vi "App Linker Info.vi"() -> ()   [LabVIEW 2020]
panel:
  out "Array 2":T1(array[cluster])=[{"Paths"=path "C:/dev/Vireo/PicoG/PicoG-App/picoG/Main UI.vi/38877c1a-f453-4dae-9d92-84bd5ba51cbc.vi", "error out"={"status"=TRUE, "code"=7, "source"="Invoke Node in App Linker Info.vi\n<APPEND>\nMethod Name: <b>Linker:Read Info From File</b>\n\nC:\\dev\\Vireo\\PicoG\\PicoG-App\\picoG\\Main UI.vi\\38877c1a-f453-4dae-9d92-84bd5ba51cbc.vi"}}, {"Paths"=path "C:/dev/Vireo/PicoG/PicoG-App/picoG/_Add App.vi/4267f4de-baa5-4d76-a96e-fc062378f624.vi", "error out"={"status"=TRUE, "code"=7, "source"="Invoke Node in App Linker Info.vi\n<APPEND>\nMethod Name: <b>Linker:Read Info From File</b>\n\nC:\\dev\\Vireo\\PicoG\\PicoG-App\\picoG\\_Add App.vi\\4267f4de-baa5-4d76-a96e-fc062378f624.vi"}}, {"Paths"=path "C:/dev/Vireo/PicoG/PicoG-App/picoG/_Add App.vi/0", "error out"={"status"=TRUE, "code"=7, "source"="Invoke Node in App Linker Info.vi\n<APPEND>\nMethod Name: <b>Linker:Read Info From File</b>\n\nC:\\dev\\Vireo\\PicoG\\PicoG-App\\picoG\\_Add App.vi\\0"}}, {"Paths"=path "C:/dev/Vireo/PicoG/Builds/picoG/ppl/PicoG-Core.lvlibp/PicoG-Processor/PicoG-Core/PlatformPluginManager/Platform by Name.vi", "error out"={"status"=TRUE, "code"=7, "source"="Invoke Node in App Linker Info.vi\n<APPEND>\nMethod Name: <b>Linker:Read Info From File</b>\n\nC:\\dev\\Vireo\\PicoG\\Builds\\picoG\\ppl\\PicoG-Core.lvlibp\\PicoG-Processor\\PicoG-Core\\PlatformPluginManager\\Platform by Name.vi"}}, {"Paths"=path "C:/dev/Vireo/PicoG/Builds/picoG/ppl/PicoG-Core.lvlibp/1abvi3w/vi.lib/Utility/LVClass/Get LV Class Default Value.vi/LabVIEW", "error out"={"status"=TRUE, "code"=7, "source"="Invoke Node in App Linker Info.vi\n<APPEND>\nMethod Name: <b>Linker:Read Info From File</b>\n\nC:\\dev\\Vireo\\PicoG\\Builds\\picoG\\ppl\\PicoG-Core.lvlibp\\1abvi3w\\vi.lib\\Utility\\LVClass\\Get LV Class Default Value.vi\\LabVIEW"}}]
  out "Array":T2(array[cluster])=[{"Path"=path "C:/dev/Vireo/PicoG/PicoG-App/picoG Main.vi", "Name"="PicoG-App.lvlib:picoG Main.vi", "Referrer"=path "C:/dev/Vireo/PicoG/PicoG-App/picoG Main.vi"}, {"Path"=path "../PicoG-App.lvlib", "Name"="PicoG-App.lvlib", "Referrer"=path "C:/dev/Vireo/PicoG/PicoG-App/picoG Main.vi"}, {"Path"=path "<vilib>/Utility/error.llb/Clear Errors.vi", "Name"="Clear Errors.vi", "Referrer"=path "C:/dev/Vireo/PicoG/PicoG-App/picoG Main.vi"}, {"Path"=path "../picoG/Ctor.vi", "Name"="PicoG-App.lvlib:picoG.lvclass:Ctor.vi", "Referrer"=path "C:/dev/Vireo/PicoG/PicoG-App/picoG Main.vi"}, {"Path"=path "../picoG/Run.vi", "Name"="PicoG-App.lvlib:picoG.lvclass:Run.vi", "Referrer"=path "C:/dev/Vireo/PicoG/PicoG-App/picoG Main.vi"}, {"Path"=path "../picoG/Cleanup.vi", "Name"="PicoG-App.lvlib:picoG.lvclass:Cleanup.vi", "Referrer"=path "C:/dev/Vireo/PicoG/PicoG-App/picoG Main.vi"}, {"Path"=path "<vilib>/Utility/error.llb/Simple Error Handler.vi", "Name"="Simple Error Handler.vi", "Referrer"=path "C:/dev/Vireo/PicoG/PicoG-App/picoG Main.vi"}, {"Path"=path "C:/dev/Vireo/PicoG/PicoG-App/PicoG-App.lvlib", "Name"="PicoG-App.lvlib", "Referrer"=path "C:/dev/Vireo/PicoG/PicoG-App/PicoG-App.lvlib"}, {"Path"=path "C:/dev/Vireo/PicoG/PicoG-App/Device/Device.lvclass", "Name"="PicoG-App.lvlib:Device.lvclass", "Referrer"=path "C:/dev/Vireo/PicoG/PicoG-App/PicoG-App.lvlib"}, {"Path"=path "C:/dev/Vireo/PicoG/PicoG-App/ViaApp/ViaApp.lvclass", "Name"="PicoG-App.lvlib:ViaApp.lvclass", "Referrer"=path "C:/dev/Vireo/PicoG/PicoG-App/PicoG-App.lvlib"}, {"Path"=path "C:/dev/Vireo/PicoG/PicoG-App/AppDetailPanel/AppDetailPanel.lvclass", "Name"="PicoG-App.lvlib:AppDetailPanel.lvclass", "Referrer"=path "C:/dev/Vireo/PicoG/PicoG-App/PicoG-App.lvlib"}, {"Path"=path "C:/dev/Vireo/PicoG/PicoG-App/DeviceDetailPanel/DeviceDetailPanel.lvclass", "Name"="PicoG-App.lvlib:DeviceDetailPanel.lvclass", "Referrer"=path "C:/dev/Vireo/PicoG/PicoG-App/PicoG-App.lvlib"}, {"Path"=path "C:/dev/Vireo/PicoG/PicoG-App/PlatformConfigPanel/PlatformConfigPanel.lvclass", "Name"="PicoG-App.lvlib:PlatformConfigPanel.lvclass", "Referrer"=path "C:/dev/Vireo/PicoG/PicoG-App/PicoG-App.lvlib"}, {"Path"=path "C:/dev/Vireo/PicoG/PicoG-App/AppListPanel/AppListPanel.lvclass", "Name"="PicoG-App.lvlib:AppListPanel.lvclass", "Referrer"=path "C:/dev/Vireo/PicoG/PicoG-App/PicoG-App.lvlib"}, {"Path"=path "C:/dev/Vireo/PicoG/PicoG-App/DeviceListPanel/DeviceListPanel.lvclass", "Name"="PicoG-App.lvlib:DeviceListPanel.lvclass", "Referrer"=path "C:/dev/Vireo/PicoG/PicoG-App/PicoG-App.lvlib"}, {"Path"=path "C:/dev/Vireo/PicoG/PicoG-App/PlatformListPanel/PlatformListPanel.lvclass", "Name"="PicoG-App.lvlib:PlatformListPanel.lvclass", "Referrer"=path "C:/dev/Vireo/PicoG/PicoG-App/PicoG-App.lvlib"}, {"Path"=path "C:/dev/Vireo/PicoG/PicoG-App/BoardArrayPanel/BoardArrayPanel.lvclass", "Name"="PicoG-App.lvlib:BoardArrayPanel.lvclass", "Referrer"=path "C:/dev/Vireo/PicoG/PicoG-App/PicoG-App.lvlib"}, {"Path"=path "C:/dev/Vireo/PicoG/PicoG-App/DeviceArrayPanel/DeviceArrayPanel.lvclass", "Name"="PicoG-App.lvlib:DeviceArrayPanel.lvclass", "Referrer"=path "C:/dev/Vireo/PicoG/PicoG-App/PicoG-App.lvlib"}, {"Path"=path "C:/dev/Vireo/PicoG/PicoG-App/GWebAppArrayPanel/GWebAppArrayPanel.lvclass", "Name"="PicoG-App.lvlib:GWebAppArrayPanel.lvclass", "Referrer"=path "C:/dev/Vireo/PicoG/PicoG-App/PicoG-App.lvlib"}, {"Path"=path "C:/dev/Vireo/PicoG/PicoG-App/PlatformArrayPanel/PlatformArrayPanel.lvclass", "Name"="PicoG-App.lvlib:PlatformArrayPanel.lvclass", "Referrer"=path "C:/dev/Vireo/PicoG/PicoG-App/PicoG-App.lvlib"}, {"Path"=path "C:/dev/Vireo/PicoG/PicoG-App/GettingStarted/GettingStarted.lvclass", "Name"="PicoG-App.lvlib:GettingStarted.lvclass", "Referrer"=path "C:/dev/Vireo/PicoG/PicoG-App/PicoG-App.lvlib"}, {"Path"=path "C:/dev/Vireo/PicoG/PicoG-App/Config Paths.vi", "Name"="PicoG-App.lvlib:Config Paths.vi", "Referrer"=path "C:/dev/Vireo/PicoG/PicoG-App/PicoG-App.lvlib"}, {"Path"=path "C:/dev/Vireo/PicoG/PicoG-App/Paths.ctl", "Name"="PicoG-App.lvlib:Paths.ctl", "Referrer"=path "C:/dev/Vireo/PicoG/PicoG-App/PicoG-App.lvlib"}, {"Path"=path "C:/dev/Vireo/PicoG/PicoG-App/picoG/Top VI FG.vi", "Name"="PicoG-App.lvlib:Top VI FG.vi", "Referrer"=path "C:/dev/Vireo/PicoG/PicoG-App/PicoG-App.lvlib"}, {"Path"=path "C:/dev/Vireo/PicoG/PicoG-App/App Watcher/App Watcher.lvclass", "Name"="PicoG-App.lvlib:App Watcher.lvclass", "Referrer"=path "C:/dev/Vireo/PicoG/PicoG-App/PicoG-App.lvlib"}, {"Path"=path "C:/dev/Vireo/PicoG/PicoG-App/Device Watcher/Device Watcher.lvclass", "Name"="PicoG-App.lvlib:Device Watcher.lvclass", "Referrer"=path "C:/dev/Vireo/PicoG/PicoG-App/PicoG-App.lvlib"}, {"Path"=path "C:/dev/Vireo/PicoG/PicoG-App/picoG Main.vi", "Name"="PicoG-App.lvlib:picoG Main.vi", "Referrer"=path "C:/dev/Vireo/PicoG/PicoG-App/PicoG-App.lvlib"}, {"Path"=path "C:/dev/Vireo/PicoG/PicoG-App/picoG/picoG.lvclass", "Name"="PicoG-App.lvlib:picoG.lvclass", "Referrer"=path "C:/dev/Vireo/PicoG/PicoG-App/PicoG-App.lvlib"}, {"Path"=path "C:/dev/Vireo/PicoG/PicoG-App/picoG/Ctor.vi", "Name"="PicoG-App.lvlib:picoG.lvclass:Ctor.vi", "Referrer"=path "C:/dev/Vireo/PicoG/PicoG-App/picoG/Ctor.vi"}, {"Path"=path "../picoG.lvclass", "Name"="PicoG-App.lvlib:picoG.lvclass", "Referrer"=path "C:/dev/Vireo/PicoG/PicoG-App/picoG/Ctor.vi"}, {"Path"=path "../picoG.lvclass/picoG.ctl", "Name"="PicoG-App.lvlib:picoG.lvclass:picoG.ctl", "Referrer"=path "C:/dev/Vireo/PicoG/PicoG-App/picoG/Ctor.vi"}, {"Path"=path "../Init Platform Plugins.vi", "Name"="PicoG-App.lvlib:picoG.lvclass:Init Platform Plugins.vi", "Referrer"=path "C:/dev/Vireo/PicoG/PicoG-App/picoG/Ctor.vi"}, {"Path"=path "../Init Events.vi", "Name"="PicoG-App.lvlib:picoG.lvclass:Init Events.vi", "Referrer"=path "C:/dev/Vireo/PicoG/PicoG-App/picoG/Ctor.vi"}, {"Path"=path "../Init Panels.vi", "Name"="PicoG-App.lvlib:picoG.lvclass:Init Panels.vi", "Referrer"=path "C:/dev/Vireo/PicoG/PicoG-App/picoG/Ctor.vi"}, {"Path"=path "../Init App Watcher.vi", "Name"="PicoG-App.lvlib:picoG.lvclass:Init App Watcher.vi", "Referrer"=path "C:/dev/Vireo/PicoG/PicoG-App/picoG/Ctor.vi"}, {"Path"=path "../Init Device Watcher.vi", "Name"="PicoG-App.lvlib:picoG.lvclass:Init Device Watcher.vi", "Referrer"=path "C:/dev/Vireo/PicoG/PicoG-App/picoG/Ctor.vi"}, {"Path"=path "../Init Config.vi", "Name"="PicoG-App.lvlib:picoG.lvclass:Init Config.vi", "Referrer"=path "C:/dev/Vireo/PicoG/PicoG-App/picoG/Ctor.vi"}, {"Path"=path "../Instance FG.vi", "Name"="PicoG-App.lvlib:picoG.lvclass:Instance FG.vi", "Referrer"=path "C:/dev/Vireo/PicoG/PicoG-App/picoG/Ctor.vi"}, {"Path"=path "C:/dev/Vireo/PicoG/PicoG-App/picoG/Run.vi", "Name"="PicoG-App.lvlib:picoG.lvclass:Run.vi", "Referrer"=path "C:/dev/Vireo/PicoG/PicoG-App/picoG/Run.vi"}, {"Path"=path "../picoG.lvclass", "Name"="PicoG-App.lvlib:picoG.lvclass", "Referrer"=path "C:/dev/Vireo/PicoG/PicoG-App/picoG/Run.vi"}, {"Path"=path "../Main UI.vi", "Name"="PicoG-App.lvlib:picoG.lvclass:Main UI.vi", "Referrer"=path "C:/dev/Vireo/PicoG/PicoG-App/picoG/Run.vi"}, {"Path"=path "../../App Watcher/Start.vi", "Name"="PicoG-App.lvlib:App Watcher.lvclass:Start.vi", "Referrer"=path "C:/dev/Vireo/PicoG/PicoG-App/picoG/Run.vi"}, {"Path"=path "C:/dev/Vireo/PicoG/PicoG-App/picoG/Cleanup.vi", "Name"="PicoG-App.lvlib:picoG.lvclass:Cleanup.vi", "Referrer"=path "C:/dev/Vireo/PicoG/PicoG-App/picoG/Cleanup.vi"}, {"Path"=path "../picoG.lvclass", "Name"="PicoG-App.lvlib:picoG.lvclass", "Referrer"=path "C:/dev/Vireo/PicoG/PicoG-App/picoG/Cleanup.vi"}, {"Path"=path "../picoG.lvclass/picoG.ctl", "Name"="PicoG-App.lvlib:picoG.lvclass:picoG.ctl", "Referrer"=path "C:/dev/Vireo/PicoG/PicoG-App/picoG/Cleanup.vi"}, {"Path"=path "../../App Watcher/Cleanup.vi", "Name"="PicoG-App.lvlib:App Watcher.lvclass:Cleanup.vi", "Referrer"=path "C:/dev/Vireo/PicoG/PicoG-App/picoG/Cleanup.vi"}, {"Path"=path "<vilib>/IlluminatedG/IG OOPanel/OOPanel/Manager/Cleanup.vi", "Name"="OOPanel.lvlib:Manager.lvclass:Cleanup.vi", "Referrer"=path "C:/dev/Vireo/PicoG/PicoG-App/picoG/Cleanup.vi"}, {"Path"=path "../../../Builds/picoG/ppl/PicoG-Core.lvlibp/PicoG-Processor/PicoG-Core/PlatformManager/Cleanup.vi", "Name"="PicoG-Core.lvlibp:PlatformManager.lvclass:Cleanup.vi", "Referrer"=path "C:/dev/Vireo/PicoG/PicoG-App/picoG/Cleanup.vi"}, {"Path"=path "C:/dev/Vireo/PicoG/PicoG-App/picoG/picoG.lvclass", "Name"="PicoG-App.lvlib:picoG.lvclass", "Referrer"=path "C:/dev/Vireo/PicoG/PicoG-App/picoG/picoG.lvclass"}, {"Path"=path "C:/dev/Vireo/PicoG/PicoG-App/PicoG-App.lvlib", "Name"="PicoG-App.lvlib", "Referrer"=path "C:/dev/Vireo/PicoG/PicoG-App/picoG/picoG.lvclass"}, {"Path"=path "C:/dev/Vireo/PicoG/PicoG-App/picoG/picoG.lvclass/picoG.ctl", "Name"="PicoG-App.lvlib:picoG.lvclass:picoG.ctl", "Referrer"=path "C:/dev/Vireo/PicoG/PicoG-App/picoG/picoG.lvclass"}, {"Path"=path "C:/dev/Vireo/PicoG/PicoG-App/picoG/Check Configs Exist.vi", "Name"="PicoG-App.lvlib:picoG.lvclass:Check Configs Exist.vi", "Referrer"=path "C:/dev/Vireo/PicoG/PicoG-App/picoG/picoG.lvclass"}, {"Path"=path "C:/dev/Vireo/PicoG/PicoG-App/picoG/Create Default System Config.vi", "Name"="PicoG-App.lvlib:picoG.lvclass:Create Default System Config.vi", "Referrer"=path "C:/dev/Vireo/PicoG/PicoG-App/picoG/picoG.lvclass"}, {"Path"=path "C:/dev/Vireo/PicoG/PicoG-App/picoG/Create Default User Config.vi", "Name"="PicoG-App.lvlib:picoG.lvclass:Create Default User Config.vi", "Referrer"=path "C:/dev/Vireo/PicoG/PicoG-App/picoG/picoG.lvclass"}, {"Path"=path "C:/dev/Vireo/PicoG/PicoG-App/picoG/Init Config.vi", "Name"="PicoG-App.lvlib:picoG.lvclass:Init Config.vi", "Referrer"=path "C:/dev/Vireo/PicoG/PicoG-App/picoG/picoG.lvclass"}, {"Path"=path "C:/dev/Vireo/PicoG/PicoG-App/picoG/Load Platform Config.vi", "Name"="PicoG-App.lvlib:picoG.lvclass:Load Platform Config.vi", "Referrer"=path "C:/dev/Vireo/PicoG/PicoG-App/picoG/picoG.lvclass"}, {"Path"=path "C:/dev/Vireo/PicoG/PicoG-App/picoG/Load User Apps.vi", "Name"="PicoG-App.lvlib:picoG.lvclass:Load User Apps.vi", "Referrer"=path "C:/dev/Vireo/PicoG/PicoG-App/picoG/picoG.lvclass"}, {"Path"=path "C:/dev/Vireo/PicoG/PicoG-App/picoG/Load User Devices.vi", "Name"="PicoG-App.lvlib:picoG.lvclass:Load User Devices.vi", "Referrer"=path "C:/dev/Vireo/PicoG/PicoG-App/picoG/picoG.lvclass"}, {"Path"=path "C:/dev/Vireo/PicoG/PicoG-App/picoG/Load User Preferences.vi", "Name"="PicoG-App.lvlib:picoG.lvclass:Load User Preferences.vi", "Referrer"=path "C:/dev/Vireo/PicoG/PicoG-App/picoG/picoG.lvclass"}, {"Path"=path "C:/dev/Vireo/PicoG/PicoG-App/picoG/Read Single Device.vi", "Name"="PicoG-App.lvlib:picoG.lvclass:Read Single Device.vi", "Referrer"=path "C:/dev/Vireo/PicoG/PicoG-App/picoG/picoG.lvclass"}, {"Path"=path "C:/dev/Vireo/PicoG/PicoG-App/picoG/Read User Apps.vi", "Name"="PicoG-App.lvlib:picoG.lvclass:Read User Apps.vi", "Referrer"=path "C:/dev/Vireo/PicoG/PicoG-App/picoG/picoG.lvclass"}, {"Path"=path "C:/dev/Vireo/PicoG/PicoG-App/picoG/Read User Devices.vi", "Name"="PicoG-App.lvlib:picoG.lvclass:Read User Devices.vi", "Referrer"=path "C:/dev/Vireo/PicoG/PicoG-App/picoG/picoG.lvclass"}, {"Path"=path "C:/dev/Vireo/PicoG/PicoG-App/picoG/Save Config.vi", "Name"="PicoG-App.lvlib:picoG.lvclass:Save Config.vi", "Referrer"=path "C:/dev/Vireo/PicoG/PicoG-App/picoG/picoG.lvclass"}, {"Path"=path "C:/dev/Vireo/PicoG/PicoG-App/picoG/Save User Apps.vi", "Name"="PicoG-App.lvlib:picoG.lvclass:Save User Apps.vi", "Referrer"=path "C:/dev/Vireo/PicoG/PicoG-App/picoG/picoG.lvclass"}, {"Path"=path "C:/dev/Vireo/PicoG/PicoG-App/picoG/Save User Devices.vi", "Name"="PicoG-App.lvlib:picoG.lvclass:Save User Devices.vi", "Referrer"=path "C:/dev/Vireo/PicoG/PicoG-App/picoG/picoG.lvclass"}, {"Path"=path "C:/dev/Vireo/PicoG/PicoG-App/picoG/Write Single Device.vi", "Name"="PicoG-App.lvlib:picoG.lvclass:Write Single Device.vi", "Referrer"=path "C:/dev/Vireo/PicoG/PicoG-App/picoG/picoG.lvclass"}, {"Path"=path "C:/dev/Vireo/PicoG/PicoG-App/picoG/Inbound Events.ctl", "Name"="PicoG-App.lvlib:picoG.lvclass:Inbound Events.ctl", "Referrer"=path "C:/dev/Vireo/PicoG/PicoG-App/picoG/picoG.lvclass"}, {"Path"=path "C:/dev/Vireo/PicoG/PicoG-App/picoG/List Panels.ctl", "Name"="PicoG-App.lvlib:picoG.lvclass:List Panels.ctl", "Referrer"=path "C:/dev/Vireo/PicoG/PicoG-App/picoG/picoG.lvclass"}, {"Path"=path "C:/dev/Vireo/PicoG/PicoG-App/picoG/Main Panels.ctl", "Name"="PicoG-App.lvlib:picoG.lvclass:Main Panels.ctl", "Referrer"=path "C:/dev/Vireo/PicoG/PicoG-App/picoG/picoG.lvclass"}, {"Path"=path "C:/dev/Vireo/PicoG/PicoG-App/picoG/Panels.ctl", "Name"="PicoG-App.lvlib:picoG.lvclass:Panels.ctl", "Referrer"=path "C:/dev/Vireo/PicoG/PicoG-App/picoG/picoG.lvclass"}, {"Path"=path "C:/dev/Vireo/PicoG/PicoG-App/picoG/UI State.ctl", "Name"="PicoG-App.lvlib:picoG.lvclass:UI State.ctl", "Referrer"=path "C:/dev/Vireo/PicoG/PicoG-App/picoG/picoG.lvclass"}, {"Path"=path "C:/dev/Vireo/PicoG/PicoG-App/picoG/Add Device.vi", "Name"="PicoG-App.lvlib:picoG.lvclass:Add Device.vi", "Referrer"=path "C:/dev/Vireo/PicoG/PicoG-App/picoG/picoG.lvclass"}, {"Path"=path "C:/dev/Vireo/PicoG/PicoG-App/picoG/Init Device Watcher.vi", "Name"="PicoG-App.lvlib:picoG.lvclass:Init Device Watcher.vi", "Referrer"=path "C:/dev/Vireo/PicoG/PicoG-App/picoG/picoG.lvclass"}, {"Path"=path "C:/dev/Vireo/PicoG/PicoG-App/picoG/Init Events.vi", "Name"="PicoG-App.lvlib:picoG.lvclass:Init Events.vi", "Referrer"=path "C:/dev/Vireo/PicoG/PicoG-App/picoG/picoG.lvclass"}, {"Path"=path "C:/dev/Vireo/PicoG/PicoG-App/picoG/Confirm Device UI.vi", "Name"="PicoG-App.lvlib:picoG.lvclass:Confirm Device UI.vi", "Referrer"=path "C:/dev/Vireo/PicoG/PicoG-App/picoG/picoG.lvclass"}, {"Path"=path "C:/dev/Vireo/PicoG/PicoG-App/picoG/Dock UI.vi", "Name"="PicoG-App.lvlib:picoG.lvclass:Dock UI.vi", "Referrer"=path "C:/dev/Vireo/PicoG/PicoG-App/picoG/picoG.lvclass"}, {"Path"=path "C:/dev/Vireo/PicoG/PicoG-App/picoG/Main UI.vi", "Name"="PicoG-App.lvlib:picoG.lvclass:Main UI.vi", "Referrer"=path "C:/dev/Vireo/PicoG/PicoG-App/picoG/picoG.lvclass"}, {"Path"=path "C:/dev/Vireo/PicoG/PicoG-App/picoG/Select Platform UI.vi", "Name"="PicoG-App.lvlib:picoG.lvclass:Select Platform UI.vi", "Referrer"=path "C:/dev/Vireo/PicoG/PicoG-App/picoG/picoG.lvclass"}, {"Path"=path "C:/dev/Vireo/PicoG/PicoG-App/picoG/Init List Panels.vi", "Name"="PicoG-App.lvlib:picoG.lvclass:Init List Panels.vi", "Referrer"=path "C:/dev/Vireo/PicoG/PicoG-App/picoG/picoG.lvclass"}, {"Path"=path "C:/dev/Vireo/PicoG/PicoG-App/picoG/Init Main Panels.vi", "Name"="PicoG-App.lvlib:picoG.lvclass:Init Main Panels.vi", "Referrer"=path "C:/dev/Vireo/PicoG/PicoG-App/picoG/picoG.lvclass"}, {"Path"=path "C:/dev/Vireo/PicoG/PicoG-App/picoG/Init Panels.vi", "Name"="PicoG-App.lvlib:picoG.lvclass:Init Panels.vi", "Referrer"=path "C:/dev/Vireo/PicoG/PicoG-App/picoG/picoG.lvclass"}, {"Path"=path "C:/dev/Vireo/PicoG/PicoG-App/picoG/Init Platform Plugins.vi", "Name"="PicoG-App.lvlib:picoG.lvclass:Init Platform Plugins.vi", "Referrer"=path "C:/dev/Vireo/PicoG/PicoG-App/picoG/picoG.lvclass"}, {"Path"=path "C:/dev/Vireo/PicoG/PicoG-App/picoG/Init App Watcher.vi", "Name"="PicoG-App.lvlib:picoG.lvclass:Init App Watcher.vi", "Referrer"=path "C:/dev/Vireo/PicoG/PicoG-App/picoG/picoG.lvclass"}, {"Path"=path "C:/dev/Vireo/PicoG/PicoG-App/picoG/_Add App.vi", "Name"="PicoG-App.lvlib:picoG.lvclass:_Add App.vi", "Referrer"=path "C:/dev/Vireo/PicoG/PicoG-App/picoG/picoG.lvclass"}, {"Path"=path "C:/dev/Vireo/PicoG/PicoG-App/picoG/Check Broken VIs.vi", "Name"="PicoG-App.lvlib:picoG.lvclass:Check Broken VIs.vi", "Referrer"=path "C:/dev/Vireo/PicoG/PicoG-App/picoG/picoG.lvclass"}, {"Path"=path "C:/dev/Vireo/PicoG/PicoG-App/picoG/Close Splash.vi", "Name"="PicoG-App.lvlib:picoG.lvclass:Close Splash.vi", "Referrer"=path "C:/dev/Vireo/PicoG/PicoG-App/picoG/picoG.lvclass"}, {"Path"=path "C:/dev/Vireo/PicoG/PicoG-App/picoG/Instance FG.vi", "Name"="PicoG-App.lvlib:picoG.lvclass:Instance FG.vi", "Referrer"=path "C:/dev/Vireo/PicoG/PicoG-App/picoG/picoG.lvclass"}, {"Path"=path "C:/dev/Vireo/PicoG/PicoG-App/picoG/Main Menu.rtm", "Name"="PicoG-App.lvlib:picoG.lvclass:Main Menu.rtm", "Referrer"=path "C:/dev/Vireo/PicoG/PicoG-App/picoG/picoG.lvclass"}, {"Path"=path "C:/dev/Vireo/PicoG/PicoG-App/picoG/Add App.vi", "Name"="PicoG-App.lvlib:picoG.lvclass:Add App.vi", "Referrer"=path "C:/dev/Vireo/PicoG/PicoG-App/picoG/picoG.lvclass"}, {"Path"=path "C:/dev/Vireo/PicoG/PicoG-App/picoG/Remove App.vi", "Name"="PicoG-App.lvlib:picoG.lvclass:Remove App.vi", "Referrer"=path "C:/dev/Vireo/PicoG/PicoG-App/picoG/picoG.lvclass"}, {"Path"=path "C:/dev/Vireo/PicoG/PicoG-App/picoG/Select Device.vi", "Name"="PicoG-App.lvlib:picoG.lvclass:Select Device.vi", "Referrer"=path "C:/dev/Vireo/PicoG/PicoG-App/picoG/picoG.lvclass"}, {"Path"=path "C:/dev/Vireo/PicoG/PicoG-App/picoG/Cleanup.vi", "Name"="PicoG-App.lvlib:picoG.lvclass:Cleanup.vi", "Referrer"=path "C:/dev/Vireo/PicoG/PicoG-App/picoG/picoG.lvclass"}, {"Path"=path "C:/dev/Vireo/PicoG/PicoG-App/picoG/Ctor.vi", "Name"="PicoG-App.lvlib:picoG.lvclass:Ctor.vi", "Referrer"=path "C:/dev/Vireo/PicoG/PicoG-App/picoG/picoG.lvclass"}, {"Path"=path "C:/dev/Vireo/PicoG/PicoG-App/picoG/Instance.vi", "Name"="PicoG-App.lvlib:picoG.lvclass:Instance.vi", "Referrer"=path "C:/dev/Vireo/PicoG/PicoG-App/picoG/picoG.lvclass"}, {"Path"=path "C:/dev/Vireo/PicoG/PicoG-App/picoG/Run.vi", "Name"="PicoG-App.lvlib:picoG.lvclass:Run.vi", "Referrer"=path "C:/dev/Vireo/PicoG/PicoG-App/picoG/picoG.lvclass"}, {"Path"=path "C:/dev/Vireo/PicoG/PicoG-App/picoG/picoG.lvclass/picoG.ctl", "Name"="PicoG-App.lvlib:picoG.lvclass:picoG.ctl", "Referrer"=path "C:/dev/Vireo/PicoG/PicoG-App/picoG/picoG.lvclass/picoG.ctl"}, {"Path"=path "..", "Name"="PicoG-App.lvlib:picoG.lvclass", "Referrer"=path "C:/dev/Vireo/PicoG/PicoG-App/picoG/picoG.lvclass/picoG.ctl"}, {"Path"=path "../../Inbound Events.ctl", "Name"="PicoG-App.lvlib:picoG.lvclass:Inbound Events.ctl", "Referrer"=path "C:/dev/Vireo/PicoG/PicoG-App/picoG/picoG.lvclass/picoG.ctl"}, {"Path"=path "../../../App Watcher/App Update Data.ctl", "Name"="PicoG-App.lvlib:App Watcher.lvclass:App Update Data.ctl", "Referrer"=path "C:/dev/Vireo/PicoG/PicoG-App/picoG/picoG.lvclass/picoG.ctl"}, {"Path"=path "../../../ViaApp/ViaApp.lvclass", "Name"="PicoG-App.lvlib:ViaApp.lvclass", "Referrer"=path "C:/dev/Vireo/PicoG/PicoG-App/picoG/picoG.lvclass/picoG.ctl"}, {"Path"=path "../../../../Builds/picoG/ppl/PicoG-Core.lvlibp/PicoG-Processor/PicoG-Core/Platform/Platform.lvclass", "Name"="PicoG-Core.lvlibp:Platform.lvclass", "Referrer"=path "C:/dev/Vireo/PicoG/PicoG-App/picoG/picoG.lvclass/picoG.ctl"}, {"Path"=path "../../../Device/Device.lvclass", "Name"="PicoG-App.lvlib:Device.lvclass", "Referrer"=path "C:/dev/Vireo/PicoG/PicoG-App/picoG/picoG.lvclass/picoG.ctl"}, {"Path"=path "../../../../Builds/picoG/ppl/PicoG-Core.lvlibp/PicoG-Processor/PicoG-Core/PlatformManager/PlatformManager.lvclass", "Name"="PicoG-Core.lvlibp:PlatformManager.lvclass", "Referrer"=path "C:/dev/Vireo/PicoG/PicoG-App/picoG/picoG.lvclass/picoG.ctl"}, {"Path"=path "../../Panels.ctl", "Name"="PicoG-App.lvlib:picoG.lvclass:Panels.ctl", "Referrer"=path "C:/dev/Vireo/PicoG/PicoG-App/picoG/picoG.lvclass/picoG.ctl"}, {"Path"=path "<vilib>/IlluminatedG/IG OOPanel/OOPanel/Manager/Manager.lvclass", "Name"="OOPanel.lvlib:Manager.lvclass", "Referrer"=path "C:/dev/Vireo/PicoG/PicoG-App/picoG/picoG.lvclass/picoG.ctl"}, {"Path"=path "../../List Panels.ctl", "Name"="PicoG-App.lvlib:picoG.lvclass:List Panels.ctl", "Referrer"=path "C:/dev/Vireo/PicoG/PicoG-App/picoG/picoG.lvclass/picoG.ctl"}, {"Path"=path "../../../AppListPanel/AppListPanel.lvclass", "Name"="PicoG-App.lvlib:AppListPanel.lvclass", "Referrer"=path "C:/dev/Vireo/PicoG/PicoG-App/picoG/picoG.lvclass/picoG.ctl"}, {"Path"=path "../../../DeviceListPanel/DeviceListPanel.lvclass", "Name"="PicoG-App.lvlib:DeviceListPanel.lvclass", "Referrer"=path "C:/dev/Vireo/PicoG/PicoG-App/picoG/picoG.lvclass/picoG.ctl"}, {"Path"=path "../../../PlatformListPanel/PlatformListPanel.lvclass", "Name"="PicoG-App.lvlib:PlatformListPanel.lvclass", "Referrer"=path "C:/dev/Vireo/PicoG/PicoG-App/picoG/picoG.lvclass/picoG.ctl"}, {"Path"=path "../../Main Panels.ctl", "Name"="PicoG-App.lvlib:picoG.lvclass:Main Panels.ctl", "Referrer"=path "C:/dev/Vireo/PicoG/PicoG-App/picoG/picoG.lvclass/picoG.ctl"}, {"Path"=path "../../../GettingStarted/GettingStarted.lvclass", "Name"="PicoG-App.lvlib:GettingStarted.lvclass", "Referrer"=path "C:/dev/Vireo/PicoG/PicoG-App/picoG/picoG.lvclass/picoG.ctl"}, {"Path"=path "../../../AppDetailPanel/AppDetailPanel.lvclass", "Name"="PicoG-App.lvlib:AppDetailPanel.lvclass", "Referrer"=path "C:/dev/Vireo/PicoG/PicoG-App/picoG/picoG.lvclass/picoG.ctl"}, {"Path"=path "../../../PlatformConfigPanel/PlatformConfigPanel.lvclass", "Name"="PicoG-App.lvlib:PlatformConfigPanel.lvclass", "Referrer"=path "C:/dev/Vireo/PicoG/PicoG-App/picoG/picoG.lvclass/picoG.ctl"}, {"Path"=path "../../../DeviceDetailPanel/DeviceDetailPanel.lvclass", "Name"="PicoG-App.lvlib:DeviceDetailPanel.lvclass", "Referrer"=path "C:/dev/Vireo/PicoG/PicoG-App/picoG/picoG.lvclass/picoG.ctl"}, {"Path"=path "../../../App Watcher/App Watcher.lvclass", "Name"="PicoG-App.lvlib:App Watcher.lvclass", "Referrer"=path "C:/dev/Vireo/PicoG/PicoG-App/picoG/picoG.lvclass/picoG.ctl"}, {"Path"=path "../../../Device Watcher/Device Watcher.lvclass", "Name"="PicoG-App.lvlib:Device Watcher.lvclass", "Referrer"=path "C:/dev/Vireo/PicoG/PicoG-App/picoG/picoG.lvclass/picoG.ctl"}, {"Path"=path "C:/dev/Vireo/PicoG/PicoG-App/picoG/Init Platform Plugins.vi", "Name"="PicoG-App.lvlib:picoG.lvclass:Init Platform Plugins.vi", "Referrer"=path "C:/dev/Vireo/PicoG/PicoG-App/picoG/Init Platform Plugins.vi"}, {"Path"=path "../picoG.lvclass", "Name"="PicoG-App.lvlib:picoG.lvclass", "Referrer"=path "C:/dev/Vireo/PicoG/PicoG-App/picoG/Init Platform Plugins.vi"}, {"Path"=path "../picoG.lvclass/picoG.ctl", "Name"="PicoG-App.lvlib:picoG.lvclass:picoG.ctl", "Referrer"=path "C:/dev/Vireo/PicoG/PicoG-App/picoG/Init Platform Plugins.vi"}, {"Path"=path "../../../Builds/picoG/ppl/PicoG-Core.lvlibp/PicoG-Processor/PicoG-Core/PlatformManager/Ctor.vi", "Name"="PicoG-Core.lvlibp:PlatformManager.lvclass:Ctor.vi", "Referrer"=path "C:/dev/Vireo/PicoG/PicoG-App/picoG/Init Platform Plugins.vi"}, {"Path"=path "C:/dev/Vireo/PicoG/PicoG-App/picoG/Init Events.vi", "Name"="PicoG-App.lvlib:picoG.lvclass:Init Events.vi", "Referrer"=path "C:/dev/Vireo/PicoG/PicoG-App/picoG/Init Events.vi"}, {"Path"=path "../picoG.lvclass", "Name"="PicoG-App.lvlib:picoG.lvclass", "Referrer"=path "C:/dev/Vireo/PicoG/PicoG-App/picoG/Init Events.vi"}, {"Path"=path "../../App Watcher/App Update Data.ctl", "Name"="PicoG-App.lvlib:App Watcher.lvclass:App Update Data.ctl", "Referrer"=path "C:/dev/Vireo/PicoG/PicoG-App/picoG/Init Events.vi"}, {"Path"=path "../../ViaApp/ViaApp.lvclass", "Name"="PicoG-App.lvlib:ViaApp.lvclass", "Referrer"=path "C:/dev/Vireo/PicoG/PicoG-App/picoG/Init Events.vi"}, {"Path"=path "../../../Builds/picoG/ppl/PicoG-Core.lvlibp/PicoG-Processor/PicoG-Core/Platform/Platform.lvclass", "Name"="PicoG-Core.lvlibp:Platform.lvclass", "Referrer"=path "C:/dev/Vireo/PicoG/PicoG-App/picoG/Init Events.vi"}, {"Path"=path "../../Device/Device.lvclass", "Name"="PicoG-App.lvlib:Device.lvclass", "Referrer"=path "C:/dev/Vireo/PicoG/PicoG-App/picoG/Init Events.vi"}, {"Path"=path "../picoG.lvclass/picoG.ctl", "Name"="PicoG-App.lvlib:picoG.lvclass:picoG.ctl", "Referrer"=path "C:/dev/Vireo/PicoG/PicoG-App/picoG/Init Events.vi"}, {"Path"=path "C:/dev/Vireo/PicoG/PicoG-App/picoG/Init Panels.vi", "Name"="PicoG-App.lvlib:picoG.lvclass:Init Panels.vi", "Referrer"=path "C:/dev/Vireo/PicoG/PicoG-App/picoG/Init Panels.vi"}, {"Path"=path "../picoG.lvclass", "Name"="PicoG-App.lvlib:picoG.lvclass", "Referrer"=path "C:/dev/Vireo/PicoG/PicoG-App/picoG/Init Panels.vi"}, {"Path"=path "../picoG.lvclass/picoG.ctl", "Name"="PicoG-App.lvlib:picoG.lvclass:picoG.ctl", "Referrer"=path "C:/dev/Vireo/PicoG/PicoG-App/picoG/Init Panels.vi"}, {"Path"=path "<vilib>/IlluminatedG/IG OOPanel/OOPanel/Manager/Ctor.vi", "Name"="OOPanel.lvlib:Manager.lvclass:Ctor.vi", "Referrer"=path "C:/dev/Vireo/PicoG/PicoG-App/picoG/Init Panels.vi"}, {"Path"=path "../Init List Panels.vi", "Name"="PicoG-App.lvlib:picoG.lvclass:Init List Panels.vi", "Referrer"=path "C:/dev/Vireo/PicoG/PicoG-App/picoG/Init Panels.vi"}, {"Path"=path "../Init Main Panels.vi", "Name"="PicoG-App.lvlib:picoG.lvclass:Init Main Panels.vi", "Referrer"=path "C:/dev/Vireo/PicoG/PicoG-App/picoG/Init Panels.vi"}, {"Path"=path "C:/dev/Vireo/PicoG/PicoG-App/picoG/Init App Watcher.vi", "Name"="PicoG-App.lvlib:picoG.lvclass:Init App Watcher.vi", "Referrer"=path "C:/dev/Vireo/PicoG/PicoG-App/picoG/Init App Watcher.vi"}, {"Path"=path "../picoG.lvclass", "Name"="PicoG-App.lvlib:picoG.lvclass", "Referrer"=path "C:/dev/Vireo/PicoG/PicoG-App/picoG/Init App Watcher.vi"}, {"Path"=path "../picoG.lvclass/picoG.ctl", "Name"="PicoG-App.lvlib:picoG.lvclass:picoG.ctl", "Referrer"=path "C:/dev/Vireo/PicoG/PicoG-App/picoG/Init App Watcher.vi"}, {"Path"=path "../../App Watcher/Ctor.vi", "Name"="PicoG-App.lvlib:App Watcher.lvclass:Ctor.vi", "Referrer"=path "C:/dev/Vireo/PicoG/PicoG-App/picoG/Init App Watcher.vi"}, {"Path"=path "../../App Watcher/Set Update Event.vi", "Name"="PicoG-App.lvlib:App Watcher.lvclass:Set Update Event.vi", "Referrer"=path "C:/dev/Vireo/PicoG/PicoG-App/picoG/Init App Watcher.vi"}, {"Path"=path "C:/dev/Vireo/PicoG/PicoG-App/picoG/Init Device Watcher.vi", "Name"="PicoG-App.lvlib:picoG.lvclass:Init Device Watcher.vi", "Referrer"=path "C:/dev/Vireo/PicoG/PicoG-App/picoG/Init Device Watcher.vi"}, {"Path"=path "../picoG.lvclass", "Name"="PicoG-App.lvlib:picoG.lvclass", "Referrer"=path "C:/dev/Vireo/PicoG/PicoG-App/picoG/Init Device Watcher.vi"}, {"Path"=path "C:/dev/Vireo/PicoG/PicoG-App/picoG/Init Config.vi", "Name"="PicoG-App.lvlib:picoG.lvclass:Init Config.vi", "Referrer"=path "C:/dev/Vireo/PicoG/PicoG-App/picoG/Init Config.vi"}, {"Path"=path "../picoG.lvclass", "Name"="PicoG-App.lvlib:picoG.lvclass", "Referrer"=path "C:/dev/Vireo/PicoG/PicoG-App/picoG/Init Config.vi"}, {"Path"=path "../Check Configs Exist.vi", "Name"="PicoG-App.lvlib:picoG.lvclass:Check Configs Exist.vi", "Referrer"=path "C:/dev/Vireo/PicoG/PicoG-App/picoG/Init Config.vi"}, {"Path"=path "../Load Platform Config.vi", "Name"="PicoG-App.lvlib:picoG.lvclass:Load Platform Config.vi", "Referrer"=path "C:/dev/Vireo/PicoG/PicoG-App/picoG/Init Config.vi"}, {"Path"=path "../Load User Devices.vi", "Name"="PicoG-App.lvlib:picoG.lvclass:Load User Devices.vi", "Referrer"=path "C:/dev/Vireo/PicoG/PicoG-App/picoG/Init Config.vi"}, {"Path"=path "../Load User Apps.vi", "Name"="PicoG-App.lvlib:picoG.lvclass:Load User Apps.vi", "Referrer"=path "C:/dev/Vireo/PicoG/PicoG-App/picoG/Init Config.vi"}, {"Path"=path "../Load User Preferences.vi", "Name"="PicoG-App.lvlib:picoG.lvclass:Load User Preferences.vi", "Referrer"=path "C:/dev/Vireo/PicoG/PicoG-App/picoG/Init Config.vi"}, {"Path"=path "C:/dev/Vireo/PicoG/PicoG-App/picoG/Instance FG.vi", "Name"="PicoG-App.lvlib:picoG.lvclass:Instance FG.vi", "Referrer"=path "C:/dev/Vireo/PicoG/PicoG-App/picoG/Instance FG.vi"}, {"Path"=path "../picoG.lvclass", "Name"="PicoG-App.lvlib:picoG.lvclass", "Referrer"=path "C:/dev/Vireo/PicoG/PicoG-App/picoG/Instance FG.vi"}, {"Path"=path "C:/dev/Vireo/PicoG/PicoG-App/picoG/Main UI.vi", "Name"="PicoG-App.lvlib:picoG.lvclass:Main UI.vi", "Referrer"=path "C:/dev/Vireo/PicoG/PicoG-App/picoG/Main UI.vi"}, {"Path"=path "../picoG.lvclass", "Name"="PicoG-App.lvlib:picoG.lvclass", "Referrer"=path "C:/dev/Vireo/PicoG/PicoG-App/picoG/Main UI.vi"}, {"Path"=path "../UI State.ctl", "Name"="PicoG-App.lvlib:picoG.lvclass:UI State.ctl", "Referrer"=path "C:/dev/Vireo/PicoG/PicoG-App/picoG/Main UI.vi"}, {"Path"=path "../Close Splash.vi", "Name"="PicoG-App.lvlib:picoG.lvclass:Close Splash.vi", "Referrer"=path "C:/dev/Vireo/PicoG/PicoG-App/picoG/Main UI.vi"}, {"Path"=path "<vilib>/IlluminatedG/IG OOPanel/OOPanel/Manager/Insert Panel into SubPanel.vi", "Name"="OOPanel.lvlib:Manager.lvclass:Insert Panel into SubPanel.vi", "Referrer"=path "C:/dev/Vireo/PicoG/PicoG-App/picoG/Main UI.vi"}, {"Path"=path "../_Add App.vi", "Name"="PicoG-App.lvlib:picoG.lvclass:_Add App.vi", "Referrer"=path "C:/dev/Vireo/PicoG/PicoG-App/picoG/Main UI.vi"}, {"Path"=path "../Top VI FG.vi", "Name"="PicoG-App.lvlib:Top VI FG.vi", "Referrer"=path "C:/dev/Vireo/PicoG/PicoG-App/picoG/Main UI.vi"}, {"Path"=path "../../AppListPanel/Update App.vi", "Name"="PicoG-App.lvlib:AppListPanel.lvclass:Update App.vi", "Referrer"=path "C:/dev/Vireo/PicoG/PicoG-App/picoG/Main UI.vi"}, {"Path"=path "../Save Config.vi", "Name"="PicoG-App.lvlib:picoG.lvclass:Save Config.vi", "Referrer"=path "C:/dev/Vireo/PicoG/PicoG-App/picoG/Main UI.vi"}, {"Path"=path "<vilib>/Utility/error.llb/Simple Error Handler.vi", "Name"="Simple Error Handler.vi", "Referrer"=path "C:/dev/Vireo/PicoG/PicoG-App/picoG/Main UI.vi"}, {"Path"=path "../../AppListPanel/Select App.vi", "Name"="PicoG-App.lvlib:AppListPanel.lvclass:Select App.vi", "Referrer"=path "C:/dev/Vireo/PicoG/PicoG-App/picoG/Main UI.vi"}, {"Path"=path "../../PlatformListPanel/Deselect Platform.vi", "Name"="PicoG-App.lvlib:PlatformListPanel.lvclass:Deselect Platform.vi", "Referrer"=path "C:/dev/Vireo/PicoG/PicoG-App/picoG/Main UI.vi"}, {"Path"=path "../../PlatformListPanel/Select Platform.vi", "Name"="PicoG-App.lvlib:PlatformListPanel.lvclass:Select Platform.vi", "Referrer"=path "C:/dev/Vireo/PicoG/PicoG-App/picoG/Main UI.vi"}, {"Path"=path "../../AppListPanel/Deselect Apps.vi", "Name"="PicoG-App.lvlib:AppListPanel.lvclass:Deselect Apps.vi", "Referrer"=path "C:/dev/Vireo/PicoG/PicoG-App/picoG/Main UI.vi"}, {"Path"=path "../../AppDetailPanel/Set App.vi", "Name"="PicoG-App.lvlib:AppDetailPanel.lvclass:Set App.vi", "Referrer"=path "C:/dev/Vireo/PicoG/PicoG-App/picoG/Main UI.vi"}, {"Path"=path "../../AppListPanel/Panel.vi", "Name"="PicoG-App.lvlib:AppListPanel.lvclass:Panel.vi", "Referrer"=path "C:/dev/Vireo/PicoG/PicoG-App/picoG/Main UI.vi"}, {"Path"=path "../Check Broken VIs.vi", "Name"="PicoG-App.lvlib:picoG.lvclass:Check Broken VIs.vi", "Referrer"=path "C:/dev/Vireo/PicoG/PicoG-App/picoG/Main UI.vi"}, {"Path"=path "<vilib>/IlluminatedG/IG OOPanel/OOPanel/Manager/Remove Panel from SubPanel.vi", "Name"="OOPanel.lvlib:Manager.lvclass:Remove Panel from SubPanel.vi", "Referrer"=path "C:/dev/Vireo/PicoG/PicoG-App/picoG/Main UI.vi"}, {"Path"=path "<vilib>/IlluminatedG/IG OOPanel/OOPanel/Manager/Get Panel from SubPanel.vi", "Name"="OOPanel.lvlib:Manager.lvclass:Get Panel from SubPanel.vi", "Referrer"=path "C:/dev/Vireo/PicoG/PicoG-App/picoG/Main UI.vi"}, {"Path"=path "../Add Device.vi", "Name"="PicoG-App.lvlib:picoG.lvclass:Add Device.vi", "Referrer"=path "C:/dev/Vireo/PicoG/PicoG-App/picoG/Main UI.vi"}, {"Path"=path "../../DeviceListPanel/Deselect Devices.vi", "Name"="PicoG-App.lvlib:DeviceListPanel.lvclass:Deselect Devices.vi", "Referrer"=path "C:/dev/Vireo/PicoG/PicoG-App/picoG/Main UI.vi"}, {"Path"=path "../../DeviceListPanel/Select Device.vi", "Name"="PicoG-App.lvlib:DeviceListPanel.lvclass:Select Device.vi", "Referrer"=path "C:/dev/Vireo/PicoG/PicoG-App/picoG/Main UI.vi"}, {"Path"=path "../../DeviceDetailPanel/Set Device.vi", "Name"="PicoG-App.lvlib:DeviceDetailPanel.lvclass:Set Device.vi", "Referrer"=path "C:/dev/Vireo/PicoG/PicoG-App/picoG/Main UI.vi"}, {"Path"=path "../../AppListPanel/Remove App.vi", "Name"="PicoG-App.lvlib:AppListPanel.lvclass:Remove App.vi", "Referrer"=path "C:/dev/Vireo/PicoG/PicoG-App/picoG/Main UI.vi"}, {"Path"=path "../../App Watcher/Remove App.vi", "Name"="PicoG-App.lvlib:App Watcher.lvclass:Remove App.vi", "Referrer"=path "C:/dev/Vireo/PicoG/PicoG-App/picoG/Main UI.vi"}, {"Path"=path "../../DeviceListPanel/Get Devices.vi", "Name"="PicoG-App.lvlib:DeviceListPanel.lvclass:Get Devices.vi", "Referrer"=path "C:/dev/Vireo/PicoG/PicoG-App/picoG/Main UI.vi"}, {"Path"=path "../../AppListPanel/Get Apps.vi", "Name"="PicoG-App.lvlib:AppListPanel.lvclass:Get Apps.vi", "Referrer"=path "C:/dev/Vireo/PicoG/PicoG-App/picoG/Main UI.vi"}, {"Path"=path "../../AppListPanel/AppListPanel.lvclass", "Name"="PicoG-App.lvlib:AppListPanel.lvclass", "Referrer"=path "C:/dev/Vireo/PicoG/PicoG-App/picoG/Main UI.vi"}, {"Path"=path "../../DeviceListPanel/DeviceListPanel.lvclass", "Name"="PicoG-App.lvlib:DeviceListPanel.lvclass", "Referrer"=path "C:/dev/Vireo/PicoG/PicoG-App/picoG/Main UI.vi"}, {"Path"=path "38877c1a-f453-4dae-9d92-84bd5ba51cbc.vi", "Name"="PicoG-App.lvlib:picoG.lvclass:Main UI.vi:Instance:38877c1a-f453-4dae-9d92-84bd5ba51cbc.vi", "Referrer"=path "C:/dev/Vireo/PicoG/PicoG-App/picoG/Main UI.vi"}, {"Path"=path "../../GettingStarted/GettingStarted.lvclass", "Name"="PicoG-App.lvlib:GettingStarted.lvclass", "Referrer"=path "C:/dev/Vireo/PicoG/PicoG-App/picoG/Main UI.vi"}, {"Path"=path "../../PlatformListPanel/PlatformListPanel.lvclass", "Name"="PicoG-App.lvlib:PlatformListPanel.lvclass", "Referrer"=path "C:/dev/Vireo/PicoG/PicoG-App/picoG/Main UI.vi"}, {"Path"=path "../../AppDetailPanel/AppDetailPanel.lvclass", "Name"="PicoG-App.lvlib:AppDetailPanel.lvclass", "Referrer"=path "C:/dev/Vireo/PicoG/PicoG-App/picoG/Main UI.vi"}, {"Path"=path "../../DeviceDetailPanel/DeviceDetailPanel.lvclass", "Name"="PicoG-App.lvlib:DeviceDetailPanel.lvclass", "Referrer"=path "C:/dev/Vireo/PicoG/PicoG-App/picoG/Main UI.vi"}, {"Path"=path "../../PlatformConfigPanel/PlatformConfigPanel.lvclass", "Name"="PicoG-App.lvlib:PlatformConfigPanel.lvclass", "Referrer"=path "C:/dev/Vireo/PicoG/PicoG-App/picoG/Main UI.vi"}, {"Path"=path "../Main Menu.rtm", "Name"="Main Menu.rtm", "Referrer"=path "C:/dev/Vireo/PicoG/PicoG-App/picoG/Main UI.vi"}, {"Path"=path "C:/dev/Vireo/PicoG/PicoG-App/App Watcher/Start.vi", "Name"="PicoG-App.lvlib:App Watcher.lvclass:Start.vi", "Referrer"=path "C:/dev/Vireo/PicoG/PicoG-App/App Watcher/Start.vi"}, {"Path"=path "../App Watcher.lvclass", "Name"="PicoG-App.lvlib:App Watcher.lvclass", "Referrer"=path "C:/dev/Vireo/PicoG/PicoG-App/App Watcher/Start.vi"}, {"Path"=path "../Watcher Loop Async.vi", "Name"="PicoG-App.lvlib:App Watcher.lvclass:Watcher Loop Async.vi", "Referrer"=path "C:/dev/Vireo/PicoG/PicoG-App/App Watcher/Start.vi"}, {"Path"=path "C:/dev/Vireo/PicoG/PicoG-App/App Watcher/Cleanup.vi", "Name"="PicoG-App.lvlib:App Watcher.lvclass:Cleanup.vi", "Referrer"=path "C:/dev/Vireo/PicoG/PicoG-App/App Watcher/Cleanup.vi"}, {"Path"=path "../App Watcher.lvclass", "Name"="PicoG-App.lvlib:App Watcher.lvclass", "Referrer"=path "C:/dev/Vireo/PicoG/PicoG-App/App Watcher/Cleanup.vi"}, {"Path"=path "../App Watcher.lvclass/App Watcher.ctl", "Name"="PicoG-App.lvlib:App Watcher.lvclass:App Watcher.ctl", "Referrer"=path "C:/dev/Vireo/PicoG/PicoG-App/App Watcher/Cleanup.vi"}, {"Path"=path "C:/dev/Vireo/PicoG/Builds/picoG/ppl/PicoG-Core.lvlibp/PicoG-Processor/PicoG-Core/PlatformManager/Cleanup.vi", "Name"="PicoG-Core.lvlibp:PlatformManager.lvclass:Cleanup.vi", "Referrer"=path "C:/dev/Vireo/PicoG/Builds/picoG/ppl/PicoG-Core.lvlibp/PicoG-Processor/PicoG-Core/PlatformManager/Cleanup.vi"}, {"Path"=path "../PlatformManager.lvclass", "Name"="PicoG-Core.lvlibp:PlatformManager.lvclass", "Referrer"=path "C:/dev/Vireo/PicoG/Builds/picoG/ppl/PicoG-Core.lvlibp/PicoG-Processor/PicoG-Core/PlatformManager/Cleanup.vi"}, {"Path"=path "../PlatformManager.lvclass/PlatformManager.ctl", "Name"="PicoG-Core.lvlibp:PlatformManager.lvclass:PlatformManager.ctl", "Referrer"=path "C:/dev/Vireo/PicoG/Builds/picoG/ppl/PicoG-Core.lvlibp/PicoG-Processor/PicoG-Core/PlatformManager/Cleanup.vi"}, {"Path"=path "C:/dev/Vireo/PicoG/PicoG-App/picoG/Inbound Events.ctl", "Name"="PicoG-App.lvlib:picoG.lvclass:Inbound Events.ctl", "Referrer"=path "C:/dev/Vireo/PicoG/PicoG-App/picoG/Inbound Events.ctl"}, {"Path"=path "../picoG.lvclass", "Name"="PicoG-App.lvlib:picoG.lvclass", "Referrer"=path "C:/dev/Vireo/PicoG/PicoG-App/picoG/Inbound Events.ctl"}, {"Path"=path "../../App Watcher/App Update Data.ctl", "Name"="PicoG-App.lvlib:App Watcher.lvclass:App Update Data.ctl", "Referrer"=path "C:/dev/Vireo/PicoG/PicoG-App/picoG/Inbound Events.ctl"}, {"Path"=path "../../ViaApp/ViaApp.lvclass", "Name"="PicoG-App.lvlib:ViaApp.lvclass", "Referrer"=path "C:/dev/Vireo/PicoG/PicoG-App/picoG/Inbound Events.ctl"}, {"Path"=path "../../../Builds/picoG/ppl/PicoG-Core.lvlibp/PicoG-Processor/PicoG-Core/Platform/Platform.lvclass", "Name"="PicoG-Core.lvlibp:Platform.lvclass", "Referrer"=path "C:/dev/Vireo/PicoG/PicoG-App/picoG/Inbound Events.ctl"}, {"Path"=path "../../Device/Device.lvclass", "Name"="PicoG-App.lvlib:Device.lvclass", "Referrer"=path "C:/dev/Vireo/PicoG/PicoG-App/picoG/Inbound Events.ctl"}, {"Path"=path "C:/dev/Vireo/PicoG/PicoG-App/App Watcher/App Update Data.ctl", "Name"="PicoG-App.lvlib:App Watcher.lvclass:App Update Data.ctl", "Referrer"=path "C:/dev/Vireo/PicoG/PicoG-App/App Watcher/App Update Data.ctl"}, {"Path"=path "../App Watcher.lvclass", "Name"="PicoG-App.lvlib:App Watcher.lvclass", "Referrer"=path "C:/dev/Vireo/PicoG/PicoG-App/App Watcher/App Update Data.ctl"}, {"Path"=path "../../ViaApp/ViaApp.lvclass", "Name"="PicoG-App.lvlib:ViaApp.lvclass", "Referrer"=path "C:/dev/Vireo/PicoG/PicoG-App/App Watcher/App Update Data.ctl"}, {"Path"=path "C:/dev/Vireo/PicoG/PicoG-App/ViaApp/ViaApp.lvclass", "Name"="PicoG-App.lvlib:ViaApp.lvclass", "Referrer"=path "C:/dev/Vireo/PicoG/PicoG-App/ViaApp/ViaApp.lvclass"}, {"Path"=path "C:/dev/Vireo/PicoG/PicoG-App/PicoG-App.lvlib", "Name"="PicoG-App.lvlib", "Referrer"=path "C:/dev/Vireo/PicoG/PicoG-App/ViaApp/ViaApp.lvclass"}, {"Path"=path "C:/dev/Vireo/PicoG/PicoG-App/ViaApp/ViaApp.lvclass/ViaApp.ctl", "Name"="PicoG-App.lvlib:ViaApp.lvclass:ViaApp.ctl", "Referrer"=path "C:/dev/Vireo/PicoG/PicoG-App/ViaApp/ViaApp.lvclass"}, {"Path"=path "C:/dev/Vireo/PicoG/PicoG-App/ViaApp/Get Path.vi", "Name"="PicoG-App.lvlib:ViaApp.lvclass:Get Path.vi", "Referrer"=path "C:/dev/Vireo/PicoG/PicoG-App/ViaApp/ViaApp.lvclass"}, {"Path"=path "C:/dev/Vireo/PicoG/PicoG-App/ViaApp/Get Updated.vi", "Name"="PicoG-App.lvlib:ViaApp.lvclass:Get Updated.vi", "Referrer"=path "C:/dev/Vireo/PicoG/PicoG-App/ViaApp/ViaApp.lvclass"}, {"Path"=path "C:/dev/Vireo/PicoG/PicoG-App/ViaApp/Set Updated.vi", "Name"="PicoG-App.lvlib:ViaApp.lvclass:Set Updated.vi", "Referrer"=path "C:/dev/Vireo/PicoG/PicoG-App/ViaApp/ViaApp.lvclass"}, {"Path"=path "C:/dev/Vireo/PicoG/PicoG-App/ViaApp/Init.vi", "Name"="PicoG-App.lvlib:ViaApp.lvclass:Init.vi", "Referrer"=path "C:/dev/Vireo/PicoG/PicoG-App/ViaApp/ViaApp.lvclass"}, {"Path"=path "C:/dev/Vireo/PicoG/Builds/picoG/ppl/PicoG-Core.lvlibp/PicoG-Processor/PicoG-Core/Platform/Platform.lvclass", "Name"="PicoG-Core.lvlibp:Platform.lvclass", "Referrer"=path "C:/dev/Vireo/PicoG/Builds/picoG/ppl/PicoG-Core.lvlibp/PicoG-Processor/PicoG-Core/Platform/Platform.lvclass"}, {"Path"=path "C:/dev/Vireo/PicoG/Builds/picoG/ppl/PicoG-Core.lvlibp", "Name"="PicoG-Core.lvlibp", "Referrer"=path "C:/dev/Vireo/PicoG/Builds/picoG/ppl/PicoG-Core.lvlibp/PicoG-Processor/PicoG-Core/Platform/Platform.lvclass"}, {"Path"=path "C:/dev/Vireo/PicoG/Builds/picoG/ppl/PicoG-Core.lvlibp/PicoG-Processor/PicoG-Core/Platform/Platform.lvclass/Platform.ctl", "Name"="PicoG-Core.lvlibp:Platform.lvclass:Platform.ctl", "Referrer"=path "C:/dev/Vireo/PicoG/Builds/picoG/ppl/PicoG-Core.lvlibp/PicoG-Processor/PicoG-Core/Platform/Platform.lvclass"}, {"Path"=path "C:/dev/Vireo/PicoG/Builds/picoG/ppl/PicoG-Core.lvlibp/PicoG-Processor/PicoG-Core/Platform/Auto Resource.vi", "Name"="PicoG-Core.lvlibp:Platform.lvclass:Auto Resource.vi", "Referrer"=path "C:/dev/Vireo/PicoG/Builds/picoG/ppl/PicoG-Core.lvlibp/PicoG-Processor/PicoG-Core/Platform/Platform.lvclass"}, {"Path"=path "C:/dev/Vireo/PicoG/Builds/picoG/ppl/PicoG-Core.lvlibp/PicoG-Processor/PicoG-Core/Platform/Platform Name.vi", "Name"="PicoG-Core.lvlibp:Platform.lvclass:Platform Name.vi", "Referrer"=path "C:/dev/Vireo/PicoG/Builds/picoG/ppl/PicoG-Core.lvlibp/PicoG-Processor/PicoG-Core/Platform/Platform.lvclass"}, {"Path"=path "C:/dev/Vireo/PicoG/Builds/picoG/ppl/PicoG-Core.lvlibp/PicoG-Processor/PicoG-Core/Platform/Choose Resource.vi", "Name"="PicoG-Core.lvlibp:Platform.lvclass:Choose Resource.vi", "Referrer"=path "C:/dev/Vireo/PicoG/Builds/picoG/ppl/PicoG-Core.lvlibp/PicoG-Processor/PicoG-Core/Platform/Platform.lvclass"}, {"Path"=path "C:/dev/Vireo/PicoG/Builds/picoG/ppl/PicoG-Core.lvlibp/PicoG-Processor/PicoG-Core/Platform/Deploy to Resource.vi", "Name"="PicoG-Core.lvlibp:Platform.lvclass:Deploy to Resource.vi", "Referrer"=path "C:/dev/Vireo/PicoG/Builds/picoG/ppl/PicoG-Core.lvlibp/PicoG-Processor/PicoG-Core/Platform/Platform.lvclass"}, {"Path"=path "C:/dev/Vireo/PicoG/Builds/picoG/ppl/PicoG-Core.lvlibp/PicoG-Processor/PicoG-Core/Platform/List Resources.vi", "Name"="PicoG-Core.lvlibp:Platform.lvclass:List Resources.vi", "Referrer"=path "C:/dev/Vireo/PicoG/Builds/picoG/ppl/PicoG-Core.lvlibp/PicoG-Processor/PicoG-Core/Platform/Platform.lvclass"}, {"Path"=path "C:/dev/Vireo/PicoG/Builds/picoG/ppl/PicoG-Core.lvlibp/PicoG-Processor/PicoG-Core/Platform/Process VIA.vi", "Name"="PicoG-Core.lvlibp:Platform.lvclass:Process VIA.vi", "Referrer"=path "C:/dev/Vireo/PicoG/Builds/picoG/ppl/PicoG-Core.lvlibp/PicoG-Processor/PicoG-Core/Platform/Platform.lvclass"}, {"Path"=path "C:/dev/Vireo/PicoG/PicoG-App/Device/Device.lvclass", "Name"="PicoG-App.lvlib:Device.lvclass", "Referrer"=path "C:/dev/Vireo/PicoG/PicoG-App/Device/Device.lvclass"}, {"Path"=path "C:/dev/Vireo/PicoG/PicoG-App/PicoG-App.lvlib", "Name"="PicoG-App.lvlib", "Referrer"=path "C:/dev/Vireo/PicoG/PicoG-App/Device/Device.lvclass"}, {"Path"=path "C:/dev/Vireo/PicoG/PicoG-App/Device/Device.lvclass/Device.ctl", "Name"="PicoG-App.lvlib:Device.lvclass:Device.ctl", "Referrer"=path "C:/dev/Vireo/PicoG/PicoG-App/Device/Device.lvclass"}, {"Path"=path "C:/dev/Vireo/PicoG/PicoG-App/Device/Ref Data.ctl", "Name"="PicoG-App.lvlib:Device.lvclass:Ref Data.ctl", "Referrer"=path "C:/dev/Vireo/PicoG/PicoG-App/Device/Device.lvclass"}, {"Path"=path "C:/dev/Vireo/PicoG/PicoG-App/Device/Resource Ref.ctl", "Name"="PicoG-App.lvlib:Device.lvclass:Resource Ref.ctl", "Referrer"=path "C:/dev/Vireo/PicoG/PicoG-App/Device/Device.lvclass"}, {"Path"=path "C:/dev/Vireo/PicoG/PicoG-App/Device/Get Alias.vi", "Name"="PicoG-App.lvlib:Device.lvclass:Get Alias.vi", "Referrer"=path "C:/dev/Vireo/PicoG/PicoG-App/Device/Device.lvclass"}, {"Path"=path "C:/dev/Vireo/PicoG/PicoG-App/Device/Set Alias.vi", "Name"="PicoG-App.lvlib:Device.lvclass:Set Alias.vi", "Referrer"=path "C:/dev/Vireo/PicoG/PicoG-App/Device/Device.lvclass"}, {"Path"=path "C:/dev/Vireo/PicoG/PicoG-App/Device/Get Board.vi", "Name"="PicoG-App.lvlib:Device.lvclass:Get Board.vi", "Referrer"=path "C:/dev/Vireo/PicoG/PicoG-App/Device/Device.lvclass"}, {"Path"=path "C:/dev/Vireo/PicoG/PicoG-App/Device/Get Build.vi", "Name"="PicoG-App.lvlib:Device.lvclass:Get Build.vi", "Referrer"=path "C:/dev/Vireo/PicoG/PicoG-App/Device/Device.lvclass"}, {"Path"=path "C:/dev/Vireo/PicoG/PicoG-App/Device/Get ID.vi", "Name"="PicoG-App.lvlib:Device.lvclass:Get ID.vi", "Referrer"=path "C:/dev/Vireo/PicoG/PicoG-App/Device/Device.lvclass"}, {"Path"=path "C:/dev/Vireo/PicoG/PicoG-App/Device/Get Map Key.vi", "Name"="PicoG-App.lvlib:Device.lvclass:Get Map Key.vi", "Referrer"=path "C:/dev/Vireo/PicoG/PicoG-App/Device/Device.lvclass"}, {"Path"=path "C:/dev/Vireo/PicoG/PicoG-App/Device/Get Platform Name.vi", "Name"="PicoG-App.lvlib:Device.lvclass:Get Platform Name.vi", "Referrer"=path "C:/dev/Vireo/PicoG/PicoG-App/Device/Device.lvclass"}, {"Path"=path "C:/dev/Vireo/PicoG/PicoG-App/Device/Get Resource.vi", "Name"="PicoG-App.lvlib:Device.lvclass:Get Resource.vi", "Referrer"=path "C:/dev/Vireo/PicoG/PicoG-App/Device/Device.lvclass"}, {"Path"=path "C:/dev/Vireo/PicoG/PicoG-App/Device/Set Resource.vi", "Name"="PicoG-App.lvlib:Device.lvclass:Set Resource.vi", "Referrer"=path "C:/dev/Vireo/PicoG/PicoG-App/Device/Device.lvclass"}, {"Path"=path "C:/dev/Vireo/PicoG/PicoG-App/Device/Get Version String.vi", "Name"="PicoG-App.lvlib:Device.lvclass:Get Version String.vi", "Referrer"=path "C:/dev/Vireo/PicoG/PicoG-App/Device/Device.lvclass"}, {"Path"=path "C:/dev/Vireo/PicoG/PicoG-App/Device/Device Key.ctl", "Name"="PicoG-App.lvlib:Device.lvclass:Device Key.ctl", "Referrer"=path "C:/dev/Vireo/PicoG/PicoG-App/Device/Device.lvclass"}, {"Path"=path "C:/dev/Vireo/PicoG/PicoG-App/Device/Start Terminal.vi", "Name"="PicoG-App.lvlib:Device.lvclass:Start Terminal.vi", "Referrer"=path "C:/dev/Vireo/PicoG/PicoG-App/Device/Device.lvclass"}, {"Path"=path "C:/dev/Vireo/PicoG/PicoG-App/Device/Ctor.vi", "Name"="PicoG-App.lvlib:Device.lvclass:Ctor.vi", "Referrer"=path "C:/dev/Vireo/PicoG/PicoG-App/Device/Device.lvclass"}, {"Path"=path "C:/dev/Vireo/PicoG/PicoG-App/Device/Init from Config.vi", "Name"="PicoG-App.lvlib:Device.lvclass:Init from Config.vi", "Referrer"=path "C:/dev/Vireo/PicoG/PicoG-App/Device/Device.lvclass"}, {"Path"=path "C:/dev/Vireo/PicoG/PicoG-App/Device/Init.vi", "Name"="PicoG-App.lvlib:Device.lvclass:Init.vi", "Referrer"=path "C:/dev/Vireo/PicoG/PicoG-App/Device/Device.lvclass"}, {"Path"=path "C:/dev/Vireo/PicoG/PicoG-App/Device/Refresh Device Info.vi", "Name"="PicoG-App.lvlib:Device.lvclass:Refresh Device Info.vi", "Referrer"=path "C:/dev/Vireo/PicoG/PicoG-App/Device/Device.lvclass"}, {"Path"=path "C:/dev/Vireo/PicoG/Builds/picoG/ppl/PicoG-Core.lvlibp/PicoG-Processor/PicoG-Core/PlatformManager/PlatformManager.lvclass", "Name"="PicoG-Core.lvlibp:PlatformManager.lvclass", "Referrer"=path "C:/dev/Vireo/PicoG/Builds/picoG/ppl/PicoG-Core.lvlibp/PicoG-Processor/PicoG-Core/PlatformManager/PlatformManager.lvclass"}, {"Path"=path "C:/dev/Vireo/PicoG/Builds/picoG/ppl/PicoG-Core.lvlibp", "Name"="PicoG-Core.lvlibp", "Referrer"=path "C:/dev/Vireo/PicoG/Builds/picoG/ppl/PicoG-Core.lvlibp/PicoG-Processor/PicoG-Core/PlatformManager/PlatformManager.lvclass"}, {"Path"=path "C:/dev/Vireo/PicoG/Builds/picoG/ppl/PicoG-Core.lvlibp/PicoG-Processor/PicoG-Core/PlatformManager/PlatformManager.lvclass/PlatformManager.ctl", "Name"="PicoG-Core.lvlibp:PlatformManager.lvclass:PlatformManager.ctl", "Referrer"=path "C:/dev/Vireo/PicoG/Builds/picoG/ppl/PicoG-Core.lvlibp/PicoG-Processor/PicoG-Core/PlatformManager/PlatformManager.lvclass"}, {"Path"=path "C:/dev/Vireo/PicoG/Builds/picoG/ppl/PicoG-Core.lvlibp/PicoG-Processor/PicoG-Core/PlatformManager/Ref Data.ctl", "Name"="PicoG-Core.lvlibp:PlatformManager.lvclass:Ref Data.ctl", "Referrer"=path "C:/dev/Vireo/PicoG/Builds/picoG/ppl/PicoG-Core.lvlibp/PicoG-Processor/PicoG-Core/PlatformManager/PlatformManager.lvclass"}, {"Path"=path "C:/dev/Vireo/PicoG/Builds/picoG/ppl/PicoG-Core.lvlibp/PicoG-Processor/PicoG-Core/PlatformManager/Load Plugins.vi", "Name"="PicoG-Core.lvlibp:PlatformManager.lvclass:Load Plugins.vi", "Referrer"=path "C:/dev/Vireo/PicoG/Builds/picoG/ppl/PicoG-Core.lvlibp/PicoG-Processor/PicoG-Core/PlatformManager/PlatformManager.lvclass"}, {"Path"=path "C:/dev/Vireo/PicoG/Builds/picoG/ppl/PicoG-Core.lvlibp/PicoG-Processor/PicoG-Core/PlatformManager/Platform Plugin Folder.vi", "Name"="PicoG-Core.lvlibp:PlatformManager.lvclass:Platform Plugin Folder.vi", "Referrer"=path "C:/dev/Vireo/PicoG/Builds/picoG/ppl/PicoG-Core.lvlibp/PicoG-Processor/PicoG-Core/PlatformManager/PlatformManager.lvclass"}, {"Path"=path "C:/dev/Vireo/PicoG/Builds/picoG/ppl/PicoG-Core.lvlibp/PicoG-Processor/PicoG-Core/PlatformManager/Get All Platforms.vi", "Name"="PicoG-Core.lvlibp:PlatformManager.lvclass:Get All Platforms.vi", "Referrer"=path "C:/dev/Vireo/PicoG/Builds/picoG/ppl/PicoG-Core.lvlibp/PicoG-Processor/PicoG-Core/PlatformManager/PlatformManager.lvclass"}, {"Path"=path "C:/dev/Vireo/PicoG/Builds/picoG/ppl/PicoG-Core.lvlibp/PicoG-Processor/PicoG-Core/PlatformManager/Platform Names.vi", "Name"="PicoG-Core.lvlibp:PlatformManager.lvclass:Platform Names.vi", "Referrer"=path "C:/dev/Vireo/PicoG/Builds/picoG/ppl/PicoG-Core.lvlibp/PicoG-Processor/PicoG-Core/PlatformManager/PlatformManager.lvclass"}, {"Path"=path "C:/dev/Vireo/PicoG/Builds/picoG/ppl/PicoG-Core.lvlibp/PicoG-Processor/PicoG-Core/PlatformManager/Cleanup.vi", "Name"="PicoG-Core.lvlibp:PlatformManager.lvclass:Cleanup.vi", "Referrer"=path "C:/dev/Vireo/PicoG/Builds/picoG/ppl/PicoG-Core.lvlibp/PicoG-Processor/PicoG-Core/PlatformManager/PlatformManager.lvclass"}, {"Path"=path "C:/dev/Vireo/PicoG/Builds/picoG/ppl/PicoG-Core.lvlibp/PicoG-Processor/PicoG-Core/PlatformManager/Ctor.vi", "Name"="PicoG-Core.lvlibp:PlatformManager.lvclass:Ctor.vi", "Referrer"=path "C:/dev/Vireo/PicoG/Builds/picoG/ppl/PicoG-Core.lvlibp/PicoG-Processor/PicoG-Core/PlatformManager/PlatformManager.lvclass"}, {"Path"=path "C:/dev/Vireo/PicoG/Builds/picoG/ppl/PicoG-Core.lvlibp/PicoG-Processor/PicoG-Core/PlatformManager/Single Platform.vi", "Name"="PicoG-Core.lvlibp:PlatformManager.lvclass:Single Platform.vi", "Referrer"=path "C:/dev/Vireo/PicoG/Builds/picoG/ppl/PicoG-Core.lvlibp/PicoG-Processor/PicoG-Core/PlatformManager/PlatformManager.lvclass"}, {"Path"=path "C:/dev/Vireo/PicoG/PicoG-App/picoG/Panels.ctl", "Name"="PicoG-App.lvlib:picoG.lvclass:Panels.ctl", "Referrer"=path "C:/dev/Vireo/PicoG/PicoG-App/picoG/Panels.ctl"}, {"Path"=path "../picoG.lvclass", "Name"="PicoG-App.lvlib:picoG.lvclass", "Referrer"=path "C:/dev/Vireo/PicoG/PicoG-App/picoG/Panels.ctl"}, {"Path"=path "<vilib>/IlluminatedG/IG OOPanel/OOPanel/Manager/Manager.lvclass", "Name"="OOPanel.lvlib:Manager.lvclass", "Referrer"=path "C:/dev/Vireo/PicoG/PicoG-App/picoG/Panels.ctl"}, {"Path"=path "../List Panels.ctl", "Name"="PicoG-App.lvlib:picoG.lvclass:List Panels.ctl", "Referrer"=path "C:/dev/Vireo/PicoG/PicoG-App/picoG/Panels.ctl"}, {"Path"=path "../../AppListPanel/AppListPanel.lvclass", "Name"="PicoG-App.lvlib:AppListPanel.lvclass", "Referrer"=path "C:/dev/Vireo/PicoG/PicoG-App/picoG/Panels.ctl"}, {"Path"=path "../../DeviceListPanel/DeviceListPanel.lvclass", "Name"="PicoG-App.lvlib:DeviceListPanel.lvclass", "Referrer"=path "C:/dev/Vireo/PicoG/PicoG-App/picoG/Panels.ctl"}, {"Path"=path "../../PlatformListPanel/PlatformListPanel.lvclass", "Name"="PicoG-App.lvlib:PlatformListPanel.lvclass", "Referrer"=path "C:/dev/Vireo/PicoG/PicoG-App/picoG/Panels.ctl"}, {"Path"=path "../Main Panels.ctl", "Name"="PicoG-App.lvlib:picoG.lvclass:Main Panels.ctl", "Referrer"=path "C:/dev/Vireo/PicoG/PicoG-App/picoG/Panels.ctl"}, {"Path"=path "../../GettingStarted/GettingStarted.lvclass", "Name"="PicoG-App.lvlib:GettingStarted.lvclass", "Referrer"=path "C:/dev/Vireo/PicoG/PicoG-App/picoG/Panels.ctl"}, {"Path"=path "../../AppDetailPanel/AppDetailPanel.lvclass", "Name"="PicoG-App.lvlib:AppDetailPanel.lvclass", "Referrer"=path "C:/dev/Vireo/PicoG/PicoG-App/picoG/Panels.ctl"}, {"Path"=path "../../PlatformConfigPanel/PlatformConfigPanel.lvclass", "Name"="PicoG-App.lvlib:PlatformConfigPanel.lvclass", "Referrer"=path "C:/dev/Vireo/PicoG/PicoG-App/picoG/Panels.ctl"}, {"Path"=path "../../DeviceDetailPanel/DeviceDetailPanel.lvclass", "Name"="PicoG-App.lvlib:DeviceDetailPanel.lvclass", "Referrer"=path "C:/dev/Vireo/PicoG/PicoG-App/picoG/Panels.ctl"}, {"Path"=path "C:/dev/Vireo/PicoG/PicoG-App/picoG/List Panels.ctl", "Name"="PicoG-App.lvlib:picoG.lvclass:List Panels.ctl", "Referrer"=path "C:/dev/Vireo/PicoG/PicoG-App/picoG/List Panels.ctl"}, {"Path"=path "../picoG.lvclass", "Name"="PicoG-App.lvlib:picoG.lvclass", "Referrer"=path "C:/dev/Vireo/PicoG/PicoG-App/picoG/List Panels.ctl"}, {"Path"=path "../../AppListPanel/AppListPanel.lvclass", "Name"="PicoG-App.lvlib:AppListPanel.lvclass", "Referrer"=path "C:/dev/Vireo/PicoG/PicoG-App/picoG/List Panels.ctl"}, {"Path"=path "../../DeviceListPanel/DeviceListPanel.lvclass", "Name"="PicoG-App.lvlib:DeviceListPanel.lvclass", "Referrer"=path "C:/dev/Vireo/PicoG/PicoG-App/picoG/List Panels.ctl"}, {"Path"=path "../../PlatformListPanel/PlatformListPanel.lvclass", "Name"="PicoG-App.lvlib:PlatformListPanel.lvclass", "Referrer"=path "C:/dev/Vireo/PicoG/PicoG-App/picoG/List Panels.ctl"}, {"Path"=path "C:/dev/Vireo/PicoG/PicoG-App/AppListPanel/AppListPanel.lvclass", "Name"="PicoG-App.lvlib:AppListPanel.lvclass", "Referrer"=path "C:/dev/Vireo/PicoG/PicoG-App/AppListPanel/AppListPanel.lvclass"}, {"Path"=path "C:/dev/Vireo/PicoG/PicoG-App/PicoG-App.lvlib", "Name"="PicoG-App.lvlib", "Referrer"=path "C:/dev/Vireo/PicoG/PicoG-App/AppListPanel/AppListPanel.lvclass"}, {"Path"=path "C:/dev/Vireo/PicoG/PicoG-App/AppListPanel/AppListPanel.lvclass/AppListPanel.ctl", "Name"="PicoG-App.lvlib:AppListPanel.lvclass:AppListPanel.ctl", "Referrer"=path "C:/dev/Vireo/PicoG/PicoG-App/AppListPanel/AppListPanel.lvclass"}, {"Path"=path "C:/dev/Vireo/PicoG/PicoG-App/AppListPanel/App Panel.ctl", "Name"="PicoG-App.lvlib:AppListPanel.lvclass:App Panel.ctl", "Referrer"=path "C:/dev/Vireo/PicoG/PicoG-App/AppListPanel/AppListPanel.lvclass"}, {"Path"=path "C:/dev/Vireo/PicoG/PicoG-App/AppListPanel/Inbound Events.ctl", "Name"="PicoG-App.lvlib:AppListPanel.lvclass:Inbound Events.ctl", "Referrer"=path "C:/dev/Vireo/PicoG/PicoG-App/AppListPanel/AppListPanel.lvclass"}, {"Path"=path "C:/dev/Vireo/PicoG/PicoG-App/AppListPanel/Outbound Events.ctl", "Name"="PicoG-App.lvlib:AppListPanel.lvclass:Outbound Events.ctl", "Referrer"=path "C:/dev/Vireo/PicoG/PicoG-App/AppListPanel/AppListPanel.lvclass"}, {"Path"=path "C:/dev/Vireo/PicoG/PicoG-App/AppListPanel/Ref Data.ctl", "Name"="PicoG-App.lvlib:AppListPanel.lvclass:Ref Data.ctl", "Referrer"=path "C:/dev/Vireo/PicoG/PicoG-App/AppListPanel/AppListPanel.lvclass"}, {"Path"=path "C:/dev/Vireo/PicoG/PicoG-App/AppListPanel/Sort Order.ctl", "Name"="PicoG-App.lvlib:AppListPanel.lvclass:Sort Order.ctl", "Referrer"=path "C:/dev/Vireo/PicoG/PicoG-App/AppListPanel/AppListPanel.lvclass"}, {"Path"=path "C:/dev/Vireo/PicoG/PicoG-App/AppListPanel/Init Events.vi", "Name"="PicoG-App.lvlib:AppListPanel.lvclass:Init Events.vi", "Referrer"=path "C:/dev/Vireo/PicoG/PicoG-App/AppListPanel/AppListPanel.lvclass"}, {"Path"=path "C:/dev/Vireo/PicoG/PicoG-App/AppListPanel/Handle Update App.vi", "Name"="PicoG-App.lvlib:AppListPanel.lvclass:Handle Update App.vi", "Referrer"=path "C:/dev/Vireo/PicoG/PicoG-App/AppListPanel/AppListPanel.lvclass"}, {"Path"=path "C:/dev/Vireo/PicoG/PicoG-App/AppListPanel/Sort Panels.vi", "Name"="PicoG-App.lvlib:AppListPanel.lvclass:Sort Panels.vi", "Referrer"=path "C:/dev/Vireo/PicoG/PicoG-App/AppListPanel/AppListPanel.lvclass"}, {"Path"=path "C:/dev/Vireo/PicoG/PicoG-App/AppListPanel/Get Apps.vi", "Name"="PicoG-App.lvlib:AppListPanel.lvclass:Get Apps.vi", "Referrer"=path "C:/dev/Vireo/PicoG/PicoG-App/AppListPanel/AppListPanel.lvclass"}, {"Path"=path "C:/dev/Vireo/PicoG/PicoG-App/AppListPanel/Get PanelArray.vi", "Name"="PicoG-App.lvlib:AppListPanel.lvclass:Get PanelArray.vi", "Referrer"=path "C:/dev/Vireo/PicoG/PicoG-App/AppListPanel/AppListPanel.lvclass"}, {"Path"=path "C:/dev/Vireo/PicoG/PicoG-App/AppListPanel/Set Select App Event.vi", "Name"="PicoG-App.lvlib:AppListPanel.lvclass:Set Select App Event.vi", "Referrer"=path "C:/dev/Vireo/PicoG/PicoG-App/AppListPanel/AppListPanel.lvclass"}, {"Path"=path "C:/dev/Vireo/PicoG/PicoG-App/AppListPanel/Cleanup.vi", "Name"="PicoG-App.lvlib:AppListPanel.lvclass:Cleanup.vi", "Referrer"=path "C:/dev/Vireo/PicoG/PicoG-App/AppListPanel/AppListPanel.lvclass"}, {"Path"=path "C:/dev/Vireo/PicoG/PicoG-App/AppListPanel/Ctor.vi", "Name"="PicoG-App.lvlib:AppListPanel.lvclass:Ctor.vi", "Referrer"=path "C:/dev/Vireo/PicoG/PicoG-App/AppListPanel/AppListPanel.lvclass"}, {"Path"=path "C:/dev/Vireo/PicoG/PicoG-App/AppListPanel/Deselect Apps.vi", "Name"="PicoG-App.lvlib:AppListPanel.lvclass:Deselect Apps.vi", "Referrer"=path "C:/dev/Vireo/PicoG/PicoG-App/AppListPanel/AppListPanel.lvclass"}, {"Path"=path "C:/dev/Vireo/PicoG/PicoG-App/AppListPanel/Remove App.vi", "Name"="PicoG-App.lvlib:AppListPanel.lvclass:Remove App.vi", "Referrer"=path "C:/dev/Vireo/PicoG/PicoG-App/AppListPanel/AppListPanel.lvclass"}, {"Path"=path "C:/dev/Vireo/PicoG/PicoG-App/AppListPanel/Select App.vi", "Name"="PicoG-App.lvlib:AppListPanel.lvclass:Select App.vi", "Referrer"=path "C:/dev/Vireo/PicoG/PicoG-App/AppListPanel/AppListPanel.lvclass"}, {"Path"=path "C:/dev/Vireo/PicoG/PicoG-App/AppListPanel/Update App.vi", "Name"="PicoG-App.lvlib:AppListPanel.lvclass:Update App.vi", "Referrer"=path "C:/dev/Vireo/PicoG/PicoG-App/AppListPanel/AppListPanel.lvclass"}, {"Path"=path "C:/dev/Vireo/PicoG/PicoG-App/AppListPanel/Sort By Name.vi", "Name"="PicoG-App.lvlib:AppListPanel.lvclass:Sort By Name.vi", "Referrer"=path "C:/dev/Vireo/PicoG/PicoG-App/AppListPanel/AppListPanel.lvclass"}, {"Path"=path "C:/dev/Vireo/PicoG/PicoG-App/AppListPanel/Sort By Updated.vi", "Name"="PicoG-App.lvlib:AppListPanel.lvclass:Sort By Updated.vi", "Referrer"=path "C:/dev/Vireo/PicoG/PicoG-App/AppListPanel/AppListPanel.lvclass"}, {"Path"=path "C:/dev/Vireo/PicoG/PicoG-App/AppListPanel/Panel.vi", "Name"="PicoG-App.lvlib:AppListPanel.lvclass:Panel.vi", "Referrer"=path "C:/dev/Vireo/PicoG/PicoG-App/AppListPanel/AppListPanel.lvclass"}, {"Path"=path "C:/Program Files (x86)/National Instruments/LabVIEW 2020/vi.lib/IlluminatedG/IG OOPanel/OOPanel/Panel/Panel.lvclass", "Name"="OOPanel.lvlib:Panel.lvclass", "Referrer"=path "C:/dev/Vireo/PicoG/PicoG-App/AppListPanel/AppListPanel.lvclass"}, {"Path"=path "C:/dev/Vireo/PicoG/PicoG-App/DeviceListPanel/DeviceListPanel.lvclass", "Name"="PicoG-App.lvlib:DeviceListPanel.lvclass", "Referrer"=path "C:/dev/Vireo/PicoG/PicoG-App/DeviceListPanel/DeviceListPanel.lvclass"}, {"Path"=path "C:/dev/Vireo/PicoG/PicoG-App/PicoG-App.lvlib", "Name"="PicoG-App.lvlib", "Referrer"=path "C:/dev/Vireo/PicoG/PicoG-App/DeviceListPanel/DeviceListPanel.lvclass"}, {"Path"=path "C:/dev/Vireo/PicoG/PicoG-App/DeviceListPanel/DeviceListPanel.lvclass/DeviceListPanel.ctl", "Name"="PicoG-App.lvlib:DeviceListPanel.lvclass:DeviceListPanel.ctl", "Referrer"=path "C:/dev/Vireo/PicoG/PicoG-App/DeviceListPanel/DeviceListPanel.lvclass"}, {"Path"=path "C:/dev/Vireo/PicoG/PicoG-App/DeviceListPanel/Device and Panel.ctl", "Name"="PicoG-App.lvlib:DeviceListPanel.lvclass:Device and Panel.ctl", "Referrer"=path "C:/dev/Vireo/PicoG/PicoG-App/DeviceListPanel/DeviceListPanel.lvclass"}, {"Path"=path "C:/dev/Vireo/PicoG/PicoG-App/DeviceListPanel/Device Update Action.ctl", "Name"="PicoG-App.lvlib:DeviceListPanel.lvclass:Device Update Action.ctl", "Referrer"=path "C:/dev/Vireo/PicoG/PicoG-App/DeviceListPanel/DeviceListPanel.lvclass"}, {"Path"=path "C:/dev/Vireo/PicoG/PicoG-App/DeviceListPanel/Inbound Events.ctl", "Name"="PicoG-App.lvlib:DeviceListPanel.lvclass:Inbound Events.ctl", "Referrer"=path "C:/dev/Vireo/PicoG/PicoG-App/DeviceListPanel/DeviceListPanel.lvclass"}, {"Path"=path "C:/dev/Vireo/PicoG/PicoG-App/DeviceListPanel/Outbound Events.ctl", "Name"="PicoG-App.lvlib:DeviceListPanel.lvclass:Outbound Events.ctl", "Referrer"=path "C:/dev/Vireo/PicoG/PicoG-App/DeviceListPanel/DeviceListPanel.lvclass"}, {"Path"=path "C:/dev/Vireo/PicoG/PicoG-App/DeviceListPanel/Ref Data.ctl", "Name"="PicoG-App.lvlib:DeviceListPanel.lvclass:Ref Data.ctl", "Referrer"=path "C:/dev/Vireo/PicoG/PicoG-App/DeviceListPanel/DeviceListPanel.lvclass"}, {"Path"=path "C:/dev/Vireo/PicoG/PicoG-App/DeviceListPanel/Init Events.vi", "Name"="PicoG-App.lvlib:DeviceListPanel.lvclass:Init Events.vi", "Referrer"=path "C:/dev/Vireo/PicoG/PicoG-App/DeviceListPanel/DeviceListPanel.lvclass"}, {"Path"=path "C:/dev/Vireo/PicoG/PicoG-App/DeviceListPanel/Confirm Device Update.vi", "Name"="PicoG-App.lvlib:DeviceListPanel.lvclass:Confirm Device Update.vi", "Referrer"=path "C:/dev/Vireo/PicoG/PicoG-App/DeviceListPanel/DeviceListPanel.lvclass"}, {"Path"=path "C:/dev/Vireo/PicoG/PicoG-App/DeviceListPanel/_Add Device.vi", "Name"="PicoG-App.lvlib:DeviceListPanel.lvclass:_Add Device.vi", "Referrer"=path "C:/dev/Vireo/PicoG/PicoG-App/DeviceListPanel/DeviceListPanel.lvclass"}, {"Path"=path "C:/dev/Vireo/PicoG/PicoG-App/DeviceListPanel/Set Add Device Event.vi", "Name"="PicoG-App.lvlib:DeviceListPanel.lvclass:Set Add Device Event.vi", "Referrer"=path "C:/dev/Vireo/PicoG/PicoG-App/DeviceListPanel/DeviceListPanel.lvclass"}, {"Path"=path "C:/dev/Vireo/PicoG/PicoG-App/DeviceListPanel/Get Devices.vi", "Name"="PicoG-App.lvlib:DeviceListPanel.lvclass:Get Devices.vi", "Referrer"=path "C:/dev/Vireo/PicoG/PicoG-App/DeviceListPanel/DeviceListPanel.lvclass"}, {"Path"=path "C:/dev/Vireo/PicoG/PicoG-App/DeviceListPanel/Set Select Device Event.vi", "Name"="PicoG-App.lvlib:DeviceListPanel.lvclass:Set Select Device Event.vi", "Referrer"=path "C:/dev/Vireo/PicoG/PicoG-App/DeviceListPanel/DeviceListPanel.lvclass"}, {"Path"=path "C:/dev/Vireo/PicoG/PicoG-App/DeviceListPanel/Cleanup.vi", "Name"="PicoG-App.lvlib:DeviceListPanel.lvclass:Cleanup.vi", "Referrer"=path "C:/dev/Vireo/PicoG/PicoG-App/DeviceListPanel/DeviceListPanel.lvclass"}, {"Path"=path "C:/dev/Vireo/PicoG/PicoG-App/DeviceListPanel/Ctor.vi", "Name"="PicoG-App.lvlib:DeviceListPanel.lvclass:Ctor.vi", "Referrer"=path "C:/dev/Vireo/PicoG/PicoG-App/DeviceListPanel/DeviceListPanel.lvclass"}, {"Path"=path "C:/dev/Vireo/PicoG/PicoG-App/DeviceListPanel/Add Device.vi", "Name"="PicoG-App.lvlib:DeviceListPanel.lvclass:Add Device.vi", "Referrer"=path "C:/dev/Vireo/PicoG/PicoG-App/DeviceListPanel/DeviceListPanel.lvclass"}, {"Path"=path "C:/dev/Vireo/PicoG/PicoG-App/DeviceListPanel/Deselect Devices.vi", "Name"="PicoG-App.lvlib:DeviceListPanel.lvclass:Deselect Devices.vi", "Referrer"=path "C:/dev/Vireo/PicoG/PicoG-App/DeviceListPanel/DeviceListPanel.lvclass"}, {"Path"=path "C:/dev/Vireo/PicoG/PicoG-App/DeviceListPanel/Select Device.vi", "Name"="PicoG-App.lvlib:DeviceListPanel.lvclass:Select Device.vi", "Referrer"=path "C:/dev/Vireo/PicoG/PicoG-App/DeviceListPanel/DeviceListPanel.lvclass"}, {"Path"=path "C:/dev/Vireo/PicoG/PicoG-App/DeviceListPanel/Panel.vi", "Name"="PicoG-App.lvlib:DeviceListPanel.lvclass:Panel.vi", "Referrer"=path "C:/dev/Vireo/PicoG/PicoG-App/DeviceListPanel/DeviceListPanel.lvclass"}, {"Path"=path "C:/Program Files (x86)/National Instruments/LabVIEW 2020/vi.lib/IlluminatedG/IG OOPanel/OOPanel/Panel/Panel.lvclass", "Name"="OOPanel.lvlib:Panel.lvclass", "Referrer"=path "C:/dev/Vireo/PicoG/PicoG-App/DeviceListPanel/DeviceListPanel.lvclass"}, {"Path"=path "C:/dev/Vireo/PicoG/PicoG-App/PlatformListPanel/PlatformListPanel.lvclass", "Name"="PicoG-App.lvlib:PlatformListPanel.lvclass", "Referrer"=path "C:/dev/Vireo/PicoG/PicoG-App/PlatformListPanel/PlatformListPanel.lvclass"}, {"Path"=path "C:/dev/Vireo/PicoG/PicoG-App/PicoG-App.lvlib", "Name"="PicoG-App.lvlib", "Referrer"=path "C:/dev/Vireo/PicoG/PicoG-App/PlatformListPanel/PlatformListPanel.lvclass"}, {"Path"=path "C:/dev/Vireo/PicoG/PicoG-App/PlatformListPanel/PlatformListPanel.lvclass/PlatformListPanel.ctl", "Name"="PicoG-App.lvlib:PlatformListPanel.lvclass:PlatformListPanel.ctl", "Referrer"=path "C:/dev/Vireo/PicoG/PicoG-App/PlatformListPanel/PlatformListPanel.lvclass"}, {"Path"=path "C:/dev/Vireo/PicoG/PicoG-App/PlatformListPanel/Set Platform Plugins.vi", "Name"="PicoG-App.lvlib:PlatformListPanel.lvclass:Set Platform Plugins.vi", "Referrer"=path "C:/dev/Vireo/PicoG/PicoG-App/PlatformListPanel/PlatformListPanel.lvclass"}, {"Path"=path "C:/dev/Vireo/PicoG/PicoG-App/PlatformListPanel/Set Select Platform Event.vi", "Name"="PicoG-App.lvlib:PlatformListPanel.lvclass:Set Select Platform Event.vi", "Referrer"=path "C:/dev/Vireo/PicoG/PicoG-App/PlatformListPanel/PlatformListPanel.lvclass"}, {"Path"=path "C:/dev/Vireo/PicoG/PicoG-App/PlatformListPanel/Cleanup.vi", "Name"="PicoG-App.lvlib:PlatformListPanel.lvclass:Cleanup.vi", "Referrer"=path "C:/dev/Vireo/PicoG/PicoG-App/PlatformListPanel/PlatformListPanel.lvclass"}, {"Path"=path "C:/dev/Vireo/PicoG/PicoG-App/PlatformListPanel/Ctor.vi", "Name"="PicoG-App.lvlib:PlatformListPanel.lvclass:Ctor.vi", "Referrer"=path "C:/dev/Vireo/PicoG/PicoG-App/PlatformListPanel/PlatformListPanel.lvclass"}, {"Path"=path "C:/dev/Vireo/PicoG/PicoG-App/PlatformListPanel/Deselect Platform.vi", "Name"="PicoG-App.lvlib:PlatformListPanel.lvclass:Deselect Platform.vi", "Referrer"=path "C:/dev/Vireo/PicoG/PicoG-App/PlatformListPanel/PlatformListPanel.lvclass"}, {"Path"=path "C:/dev/Vireo/PicoG/PicoG-App/PlatformListPanel/Select Platform.vi", "Name"="PicoG-App.lvlib:PlatformListPanel.lvclass:Select Platform.vi", "Referrer"=path "C:/dev/Vireo/PicoG/PicoG-App/PlatformListPanel/PlatformListPanel.lvclass"}, {"Path"=path "C:/dev/Vireo/PicoG/PicoG-App/PlatformListPanel/Panel.vi", "Name"="PicoG-App.lvlib:PlatformListPanel.lvclass:Panel.vi", "Referrer"=path "C:/dev/Vireo/PicoG/PicoG-App/PlatformListPanel/PlatformListPanel.lvclass"}, {"Path"=path "C:/Program Files (x86)/National Instruments/LabVIEW 2020/vi.lib/IlluminatedG/IG OOPanel/OOPanel/Panel/Panel.lvclass", "Name"="OOPanel.lvlib:Panel.lvclass", "Referrer"=path "C:/dev/Vireo/PicoG/PicoG-App/PlatformListPanel/PlatformListPanel.lvclass"}, {"Path"=path "C:/dev/Vireo/PicoG/PicoG-App/picoG/Main Panels.ctl", "Name"="PicoG-App.lvlib:picoG.lvclass:Main Panels.ctl", "Referrer"=path "C:/dev/Vireo/PicoG/PicoG-App/picoG/Main Panels.ctl"}, {"Path"=path "../picoG.lvclass", "Name"="PicoG-App.lvlib:picoG.lvclass", "Referrer"=path "C:/dev/Vireo/PicoG/PicoG-App/picoG/Main Panels.ctl"}, {"Path"=path "../../GettingStarted/GettingStarted.lvclass", "Name"="PicoG-App.lvlib:GettingStarted.lvclass", "Referrer"=path "C:/dev/Vireo/PicoG/PicoG-App/picoG/Main Panels.ctl"}, {"Path"=path "../../AppDetailPanel/AppDetailPanel.lvclass", "Name"="PicoG-App.lvlib:AppDetailPanel.lvclass", "Referrer"=path "C:/dev/Vireo/PicoG/PicoG-App/picoG/Main Panels.ctl"}, {"Path"=path "../../PlatformConfigPanel/PlatformConfigPanel.lvclass", "Name"="PicoG-App.lvlib:PlatformConfigPanel.lvclass", "Referrer"=path "C:/dev/Vireo/PicoG/PicoG-App/picoG/Main Panels.ctl"}, {"Path"=path "../../DeviceDetailPanel/DeviceDetailPanel.lvclass", "Name"="PicoG-App.lvlib:DeviceDetailPanel.lvclass", "Referrer"=path "C:/dev/Vireo/PicoG/PicoG-App/picoG/Main Panels.ctl"}, {"Path"=path "C:/dev/Vireo/PicoG/PicoG-App/GettingStarted/GettingStarted.lvclass", "Name"="PicoG-App.lvlib:GettingStarted.lvclass", "Referrer"=path "C:/dev/Vireo/PicoG/PicoG-App/GettingStarted/GettingStarted.lvclass"}, {"Path"=path "C:/dev/Vireo/PicoG/PicoG-App/PicoG-App.lvlib", "Name"="PicoG-App.lvlib", "Referrer"=path "C:/dev/Vireo/PicoG/PicoG-App/GettingStarted/GettingStarted.lvclass"}, {"Path"=path "C:/dev/Vireo/PicoG/PicoG-App/GettingStarted/GettingStarted.lvclass/GettingStarted.ctl", "Name"="PicoG-App.lvlib:GettingStarted.lvclass:GettingStarted.ctl", "Referrer"=path "C:/dev/Vireo/PicoG/PicoG-App/GettingStarted/GettingStarted.lvclass"}, {"Path"=path "C:/dev/Vireo/PicoG/PicoG-App/GettingStarted/Cleanup.vi", "Name"="PicoG-App.lvlib:GettingStarted.lvclass:Cleanup.vi", "Referrer"=path "C:/dev/Vireo/PicoG/PicoG-App/GettingStarted/GettingStarted.lvclass"}, {"Path"=path "C:/dev/Vireo/PicoG/PicoG-App/GettingStarted/Ctor.vi", "Name"="PicoG-App.lvlib:GettingStarted.lvclass:Ctor.vi", "Referrer"=path "C:/dev/Vireo/PicoG/PicoG-App/GettingStarted/GettingStarted.lvclass"}, {"Path"=path "C:/dev/Vireo/PicoG/PicoG-App/GettingStarted/Panel.vi", "Name"="PicoG-App.lvlib:GettingStarted.lvclass:Panel.vi", "Referrer"=path "C:/dev/Vireo/PicoG/PicoG-App/GettingStarted/GettingStarted.lvclass"}, {"Path"=path "C:/Program Files (x86)/National Instruments/LabVIEW 2020/vi.lib/IlluminatedG/IG OOPanel/OOPanel/Panel/Panel.lvclass", "Name"="OOPanel.lvlib:Panel.lvclass", "Referrer"=path "C:/dev/Vireo/PicoG/PicoG-App/GettingStarted/GettingStarted.lvclass"}, {"Path"=path "C:/dev/Vireo/PicoG/PicoG-App/AppDetailPanel/AppDetailPanel.lvclass", "Name"="PicoG-App.lvlib:AppDetailPanel.lvclass", "Referrer"=path "C:/dev/Vireo/PicoG/PicoG-App/AppDetailPanel/AppDetailPanel.lvclass"}, {"Path"=path "C:/dev/Vireo/PicoG/PicoG-App/PicoG-App.lvlib", "Name"="PicoG-App.lvlib", "Referrer"=path "C:/dev/Vireo/PicoG/PicoG-App/AppDetailPanel/AppDetailPanel.lvclass"}, {"Path"=path "C:/dev/Vireo/PicoG/PicoG-App/AppDetailPanel/AppDetailPanel.lvclass/AppDetailPanel.ctl", "Name"="PicoG-App.lvlib:AppDetailPanel.lvclass:AppDetailPanel.ctl", "Referrer"=path "C:/dev/Vireo/PicoG/PicoG-App/AppDetailPanel/AppDetailPanel.lvclass"}, {"Path"=path "C:/dev/Vireo/PicoG/PicoG-App/AppDetailPanel/Incoming Events.ctl", "Name"="PicoG-App.lvlib:AppDetailPanel.lvclass:Incoming Events.ctl", "Referrer"=path "C:/dev/Vireo/PicoG/PicoG-App/AppDetailPanel/AppDetailPanel.lvclass"}, {"Path"=path "C:/dev/Vireo/PicoG/PicoG-App/AppDetailPanel/Ref Data.ctl", "Name"="PicoG-App.lvlib:AppDetailPanel.lvclass:Ref Data.ctl", "Referrer"=path "C:/dev/Vireo/PicoG/PicoG-App/AppDetailPanel/AppDetailPanel.lvclass"}, {"Path"=path "C:/dev/Vireo/PicoG/PicoG-App/AppDetailPanel/Set App.vi", "Name"="PicoG-App.lvlib:AppDetailPanel.lvclass:Set App.vi", "Referrer"=path "C:/dev/Vireo/PicoG/PicoG-App/AppDetailPanel/AppDetailPanel.lvclass"}, {"Path"=path "C:/dev/Vireo/PicoG/PicoG-App/AppDetailPanel/Cleanup.vi", "Name"="PicoG-App.lvlib:AppDetailPanel.lvclass:Cleanup.vi", "Referrer"=path "C:/dev/Vireo/PicoG/PicoG-App/AppDetailPanel/AppDetailPanel.lvclass"}, {"Path"=path "C:/dev/Vireo/PicoG/PicoG-App/AppDetailPanel/Ctor.vi", "Name"="PicoG-App.lvlib:AppDetailPanel.lvclass:Ctor.vi", "Referrer"=path "C:/dev/Vireo/PicoG/PicoG-App/AppDetailPanel/AppDetailPanel.lvclass"}, {"Path"=path "C:/dev/Vireo/PicoG/PicoG-App/AppDetailPanel/Panel.vi", "Name"="PicoG-App.lvlib:AppDetailPanel.lvclass:Panel.vi", "Referrer"=path "C:/dev/Vireo/PicoG/PicoG-App/AppDetailPanel/AppDetailPanel.lvclass"}, {"Path"=path "C:/Program Files (x86)/National Instruments/LabVIEW 2020/vi.lib/IlluminatedG/IG OOPanel/OOPanel/Panel/Panel.lvclass", "Name"="OOPanel.lvlib:Panel.lvclass", "Referrer"=path "C:/dev/Vireo/PicoG/PicoG-App/AppDetailPanel/AppDetailPanel.lvclass"}, {"Path"=path "C:/dev/Vireo/PicoG/PicoG-App/PlatformConfigPanel/PlatformConfigPanel.lvclass", "Name"="PicoG-App.lvlib:PlatformConfigPanel.lvclass", "Referrer"=path "C:/dev/Vireo/PicoG/PicoG-App/PlatformConfigPanel/PlatformConfigPanel.lvclass"}, {"Path"=path "C:/dev/Vireo/PicoG/PicoG-App/PicoG-App.lvlib", "Name"="PicoG-App.lvlib", "Referrer"=path "C:/dev/Vireo/PicoG/PicoG-App/PlatformConfigPanel/PlatformConfigPanel.lvclass"}, {"Path"=path "C:/dev/Vireo/PicoG/PicoG-App/PlatformConfigPanel/PlatformConfigPanel.lvclass/PlatformConfigPanel.ctl", "Name"="PicoG-App.lvlib:PlatformConfigPanel.lvclass:PlatformConfigPanel.ctl", "Referrer"=path "C:/dev/Vireo/PicoG/PicoG-App/PlatformConfigPanel/PlatformConfigPanel.lvclass"}, {"Path"=path "C:/dev/Vireo/PicoG/PicoG-App/PlatformConfigPanel/Cleanup.vi", "Name"="PicoG-App.lvlib:PlatformConfigPanel.lvclass:Cleanup.vi", "Referrer"=path "C:/dev/Vireo/PicoG/PicoG-App/PlatformConfigPanel/PlatformConfigPanel.lvclass"}, {"Path"=path "C:/dev/Vireo/PicoG/PicoG-App/PlatformConfigPanel/Ctor.vi", "Name"="PicoG-App.lvlib:PlatformConfigPanel.lvclass:Ctor.vi", "Referrer"=path "C:/dev/Vireo/PicoG/PicoG-App/PlatformConfigPanel/PlatformConfigPanel.lvclass"}, {"Path"=path "C:/dev/Vireo/PicoG/PicoG-App/PlatformConfigPanel/Panel.vi", "Name"="PicoG-App.lvlib:PlatformConfigPanel.lvclass:Panel.vi", "Referrer"=path "C:/dev/Vireo/PicoG/PicoG-App/PlatformConfigPanel/PlatformConfigPanel.lvclass"}, {"Path"=path "C:/Program Files (x86)/National Instruments/LabVIEW 2020/vi.lib/IlluminatedG/IG OOPanel/OOPanel/Panel/Panel.lvclass", "Name"="OOPanel.lvlib:Panel.lvclass", "Referrer"=path "C:/dev/Vireo/PicoG/PicoG-App/PlatformConfigPanel/PlatformConfigPanel.lvclass"}, {"Path"=path "C:/dev/Vireo/PicoG/PicoG-App/DeviceDetailPanel/DeviceDetailPanel.lvclass", "Name"="PicoG-App.lvlib:DeviceDetailPanel.lvclass", "Referrer"=path "C:/dev/Vireo/PicoG/PicoG-App/DeviceDetailPanel/DeviceDetailPanel.lvclass"}, {"Path"=path "C:/dev/Vireo/PicoG/PicoG-App/PicoG-App.lvlib", "Name"="PicoG-App.lvlib", "Referrer"=path "C:/dev/Vireo/PicoG/PicoG-App/DeviceDetailPanel/DeviceDetailPanel.lvclass"}, {"Path"=path "C:/dev/Vireo/PicoG/PicoG-App/DeviceDetailPanel/DeviceDetailPanel.lvclass/DeviceDetailPanel.ctl", "Name"="PicoG-App.lvlib:DeviceDetailPanel.lvclass:DeviceDetailPanel.ctl", "Referrer"=path "C:/dev/Vireo/PicoG/PicoG-App/DeviceDetailPanel/DeviceDetailPanel.lvclass"}, {"Path"=path "C:/dev/Vireo/PicoG/PicoG-App/DeviceDetailPanel/Inbound Events.ctl", "Name"="PicoG-App.lvlib:DeviceDetailPanel.lvclass:Inbound Events.ctl", "Referrer"=path "C:/dev/Vireo/PicoG/PicoG-App/DeviceDetailPanel/DeviceDetailPanel.lvclass"}, {"Path"=path "C:/dev/Vireo/PicoG/PicoG-App/DeviceDetailPanel/Ref Data.ctl", "Name"="PicoG-App.lvlib:DeviceDetailPanel.lvclass:Ref Data.ctl", "Referrer"=path "C:/dev/Vireo/PicoG/PicoG-App/DeviceDetailPanel/DeviceDetailPanel.lvclass"}, {"Path"=path "C:/dev/Vireo/PicoG/PicoG-App/DeviceDetailPanel/Terminal State.ctl", "Name"="PicoG-App.lvlib:DeviceDetailPanel.lvclass:Terminal State.ctl", "Referrer"=path "C:/dev/Vireo/PicoG/PicoG-App/DeviceDetailPanel/DeviceDetailPanel.lvclass"}, {"Path"=path "C:/dev/Vireo/PicoG/PicoG-App/DeviceDetailPanel/Get Device.vi", "Name"="PicoG-App.lvlib:DeviceDetailPanel.lvclass:Get Device.vi", "Referrer"=path "C:/dev/Vireo/PicoG/PicoG-App/DeviceDetailPanel/DeviceDetailPanel.lvclass"}, {"Path"=path "C:/dev/Vireo/PicoG/PicoG-App/DeviceDetailPanel/Set Device.vi", "Name"="PicoG-App.lvlib:DeviceDetailPanel.lvclass:Set Device.vi", "Referrer"=path "C:/dev/Vireo/PicoG/PicoG-App/DeviceDetailPanel/DeviceDetailPanel.lvclass"}, {"Path"=path "C:/dev/Vireo/PicoG/PicoG-App/DeviceDetailPanel/Cleanup.vi", "Name"="PicoG-App.lvlib:DeviceDetailPanel.lvclass:Cleanup.vi", "Referrer"=path "C:/dev/Vireo/PicoG/PicoG-App/DeviceDetailPanel/DeviceDetailPanel.lvclass"}, {"Path"=path "C:/dev/Vireo/PicoG/PicoG-App/DeviceDetailPanel/Ctor.vi", "Name"="PicoG-App.lvlib:DeviceDetailPanel.lvclass:Ctor.vi", "Referrer"=path "C:/dev/Vireo/PicoG/PicoG-App/DeviceDetailPanel/DeviceDetailPanel.lvclass"}, {"Path"=path "C:/dev/Vireo/PicoG/PicoG-App/DeviceDetailPanel/Panel.vi", "Name"="PicoG-App.lvlib:DeviceDetailPanel.lvclass:Panel.vi", "Referrer"=path "C:/dev/Vireo/PicoG/PicoG-App/DeviceDetailPanel/DeviceDetailPanel.lvclass"}, {"Path"=path "C:/Program Files (x86)/National Instruments/LabVIEW 2020/vi.lib/IlluminatedG/IG OOPanel/OOPanel/Panel/Panel.lvclass", "Name"="OOPanel.lvlib:Panel.lvclass", "Referrer"=path "C:/dev/Vireo/PicoG/PicoG-App/DeviceDetailPanel/DeviceDetailPanel.lvclass"}, {"Path"=path "C:/dev/Vireo/PicoG/PicoG-App/App Watcher/App Watcher.lvclass", "Name"="PicoG-App.lvlib:App Watcher.lvclass", "Referrer"=path "C:/dev/Vireo/PicoG/PicoG-App/App Watcher/App Watcher.lvclass"}, {"Path"=path "C:/dev/Vireo/PicoG/PicoG-App/PicoG-App.lvlib", "Name"="PicoG-App.lvlib", "Referrer"=path "C:/dev/Vireo/PicoG/PicoG-App/App Watcher/App Watcher.lvclass"}, {"Path"=path "C:/dev/Vireo/PicoG/PicoG-App/App Watcher/App Watcher.lvclass/App Watcher.ctl", "Name"="PicoG-App.lvlib:App Watcher.lvclass:App Watcher.ctl", "Referrer"=path "C:/dev/Vireo/PicoG/PicoG-App/App Watcher/App Watcher.lvclass"}, {"Path"=path "C:/dev/Vireo/PicoG/PicoG-App/App Watcher/Ref Data.ctl", "Name"="PicoG-App.lvlib:App Watcher.lvclass:Ref Data.ctl", "Referrer"=path "C:/dev/Vireo/PicoG/PicoG-App/App Watcher/App Watcher.lvclass"}, {"Path"=path "C:/dev/Vireo/PicoG/PicoG-App/App Watcher/Check Apps.vi", "Name"="PicoG-App.lvlib:App Watcher.lvclass:Check Apps.vi", "Referrer"=path "C:/dev/Vireo/PicoG/PicoG-App/App Watcher/App Watcher.lvclass"}, {"Path"=path "C:/dev/Vireo/PicoG/PicoG-App/App Watcher/Watcher Loop Async.vi", "Name"="PicoG-App.lvlib:App Watcher.lvclass:Watcher Loop Async.vi", "Referrer"=path "C:/dev/Vireo/PicoG/PicoG-App/App Watcher/App Watcher.lvclass"}, {"Path"=path "C:/dev/Vireo/PicoG/PicoG-App/App Watcher/Set Update Event.vi", "Name"="PicoG-App.lvlib:App Watcher.lvclass:Set Update Event.vi", "Referrer"=path "C:/dev/Vireo/PicoG/PicoG-App/App Watcher/App Watcher.lvclass"}, {"Path"=path "C:/dev/Vireo/PicoG/PicoG-App/App Watcher/App Update Data.ctl", "Name"="PicoG-App.lvlib:App Watcher.lvclass:App Update Data.ctl", "Referrer"=path "C:/dev/Vireo/PicoG/PicoG-App/App Watcher/App Watcher.lvclass"}, {"Path"=path "C:/dev/Vireo/PicoG/PicoG-App/App Watcher/Add App.vi", "Name"="PicoG-App.lvlib:App Watcher.lvclass:Add App.vi", "Referrer"=path "C:/dev/Vireo/PicoG/PicoG-App/App Watcher/App Watcher.lvclass"}, {"Path"=path "C:/dev/Vireo/PicoG/PicoG-App/App Watcher/Cleanup.vi", "Name"="PicoG-App.lvlib:App Watcher.lvclass:Cleanup.vi", "Referrer"=path "C:/dev/Vireo/PicoG/PicoG-App/App Watcher/App Watcher.lvclass"}, {"Path"=path "C:/dev/Vireo/PicoG/PicoG-App/App Watcher/Ctor.vi", "Name"="PicoG-App.lvlib:App Watcher.lvclass:Ctor.vi", "Referrer"=path "C:/dev/Vireo/PicoG/PicoG-App/App Watcher/App Watcher.lvclass"}, {"Path"=path "C:/dev/Vireo/PicoG/PicoG-App/App Watcher/Remove App.vi", "Name"="PicoG-App.lvlib:App Watcher.lvclass:Remove App.vi", "Referrer"=path "C:/dev/Vireo/PicoG/PicoG-App/App Watcher/App Watcher.lvclass"}, {"Path"=path "C:/dev/Vireo/PicoG/PicoG-App/App Watcher/Start.vi", "Name"="PicoG-App.lvlib:App Watcher.lvclass:Start.vi", "Referrer"=path "C:/dev/Vireo/PicoG/PicoG-App/App Watcher/App Watcher.lvclass"}, {"Path"=path "C:/dev/Vireo/PicoG/PicoG-App/Device Watcher/Device Watcher.lvclass", "Name"="PicoG-App.lvlib:Device Watcher.lvclass", "Referrer"=path "C:/dev/Vireo/PicoG/PicoG-App/Device Watcher/Device Watcher.lvclass"}, {"Path"=path "C:/dev/Vireo/PicoG/PicoG-App/PicoG-App.lvlib", "Name"="PicoG-App.lvlib", "Referrer"=path "C:/dev/Vireo/PicoG/PicoG-App/Device Watcher/Device Watcher.lvclass"}, {"Path"=path "C:/dev/Vireo/PicoG/PicoG-App/Device Watcher/Device Watcher.lvclass/Device Watcher.ctl", "Name"="PicoG-App.lvlib:Device Watcher.lvclass:Device Watcher.ctl", "Referrer"=path "C:/dev/Vireo/PicoG/PicoG-App/Device Watcher/Device Watcher.lvclass"}, {"Path"=path "C:/dev/Vireo/PicoG/Builds/picoG/ppl/PicoG-Core.lvlibp/PicoG-Processor/PicoG-Core/PlatformManager/Ctor.vi", "Name"="PicoG-Core.lvlibp:PlatformManager.lvclass:Ctor.vi", "Referrer"=path "C:/dev/Vireo/PicoG/Builds/picoG/ppl/PicoG-Core.lvlibp/PicoG-Processor/PicoG-Core/PlatformManager/Ctor.vi"}, {"Path"=path "../PlatformManager.lvclass", "Name"="PicoG-Core.lvlibp:PlatformManager.lvclass", "Referrer"=path "C:/dev/Vireo/PicoG/Builds/picoG/ppl/PicoG-Core.lvlibp/PicoG-Processor/PicoG-Core/PlatformManager/Ctor.vi"}, {"Path"=path "../Ref Data.ctl", "Name"="PicoG-Core.lvlibp:PlatformManager.lvclass:Ref Data.ctl", "Referrer"=path "C:/dev/Vireo/PicoG/Builds/picoG/ppl/PicoG-Core.lvlibp/PicoG-Processor/PicoG-Core/PlatformManager/Ctor.vi"}, {"Path"=path "../../Platform/Platform.lvclass", "Name"="PicoG-Core.lvlibp:Platform.lvclass", "Referrer"=path "C:/dev/Vireo/PicoG/Builds/picoG/ppl/PicoG-Core.lvlibp/PicoG-Processor/PicoG-Core/PlatformManager/Ctor.vi"}, {"Path"=path "../PlatformManager.lvclass/PlatformManager.ctl", "Name"="PicoG-Core.lvlibp:PlatformManager.lvclass:PlatformManager.ctl", "Referrer"=path "C:/dev/Vireo/PicoG/Builds/picoG/ppl/PicoG-Core.lvlibp/PicoG-Processor/PicoG-Core/PlatformManager/Ctor.vi"}, {"Path"=path "../Load Plugins.vi", "Name"="PicoG-Core.lvlibp:PlatformManager.lvclass:Load Plugins.vi", "Referrer"=path "C:/dev/Vireo/PicoG/Builds/picoG/ppl/PicoG-Core.lvlibp/PicoG-Processor/PicoG-Core/PlatformManager/Ctor.vi"}, {"Path"=path "C:/dev/Vireo/PicoG/PicoG-App/picoG/Init List Panels.vi", "Name"="PicoG-App.lvlib:picoG.lvclass:Init List Panels.vi", "Referrer"=path "C:/dev/Vireo/PicoG/PicoG-App/picoG/Init List Panels.vi"}, {"Path"=path "../picoG.lvclass", "Name"="PicoG-App.lvlib:picoG.lvclass", "Referrer"=path "C:/dev/Vireo/PicoG/PicoG-App/picoG/Init List Panels.vi"}, {"Path"=path "../../AppListPanel/AppListPanel.lvclass", "Name"="PicoG-App.lvlib:AppListPanel.lvclass", "Referrer"=path "C:/dev/Vireo/PicoG/PicoG-App/picoG/Init List Panels.vi"}, {"Path"=path "../../DeviceListPanel/DeviceListPanel.lvclass", "Name"="PicoG-App.lvlib:DeviceListPanel.lvclass", "Referrer"=path "C:/dev/Vireo/PicoG/PicoG-App/picoG/Init List Panels.vi"}, {"Path"=path "../../PlatformListPanel/PlatformListPanel.lvclass", "Name"="PicoG-App.lvlib:PlatformListPanel.lvclass", "Referrer"=path "C:/dev/Vireo/PicoG/PicoG-App/picoG/Init List Panels.vi"}, {"Path"=path "../picoG.lvclass/picoG.ctl", "Name"="PicoG-App.lvlib:picoG.lvclass:picoG.ctl", "Referrer"=path "C:/dev/Vireo/PicoG/PicoG-App/picoG/Init List Panels.vi"}, {"Path"=path "../../AppListPanel/Set Select App Event.vi", "Name"="PicoG-App.lvlib:AppListPanel.lvclass:Set Select App Event.vi", "Referrer"=path "C:/dev/Vireo/PicoG/PicoG-App/picoG/Init List Panels.vi"}, {"Path"=path "<vilib>/IlluminatedG/IG OOPanel/OOPanel/Manager/Create Panel by Type.vi", "Name"="OOPanel.lvlib:Manager.lvclass:Create Panel by Type.vi", "Referrer"=path "C:/dev/Vireo/PicoG/PicoG-App/picoG/Init List Panels.vi"}, {"Path"=path "../../DeviceListPanel/Set Select Device Event.vi", "Name"="PicoG-App.lvlib:DeviceListPanel.lvclass:Set Select Device Event.vi", "Referrer"=path "C:/dev/Vireo/PicoG/PicoG-App/picoG/Init List Panels.vi"}, {"Path"=path "../../DeviceListPanel/Set Add Device Event.vi", "Name"="PicoG-App.lvlib:DeviceListPanel.lvclass:Set Add Device Event.vi", "Referrer"=path "C:/dev/Vireo/PicoG/PicoG-App/picoG/Init List Panels.vi"}, {"Path"=path "../../PlatformListPanel/Set Select Platform Event.vi", "Name"="PicoG-App.lvlib:PlatformListPanel.lvclass:Set Select Platform Event.vi", "Referrer"=path "C:/dev/Vireo/PicoG/PicoG-App/picoG/Init List Panels.vi"}, {"Path"=path "../../PlatformListPanel/Set Platform Plugins.vi", "Name"="PicoG-App.lvlib:PlatformListPanel.lvclass:Set Platform Plugins.vi", "Referrer"=path "C:/dev/Vireo/PicoG/PicoG-App/picoG/Init List Panels.vi"}, {"Path"=path "C:/dev/Vireo/PicoG/PicoG-App/picoG/Init Main Panels.vi", "Name"="PicoG-App.lvlib:picoG.lvclass:Init Main Panels.vi", "Referrer"=path "C:/dev/Vireo/PicoG/PicoG-App/picoG/Init Main Panels.vi"}, {"Path"=path "../picoG.lvclass", "Name"="PicoG-App.lvlib:picoG.lvclass", "Referrer"=path "C:/dev/Vireo/PicoG/PicoG-App/picoG/Init Main Panels.vi"}, {"Path"=path "../../GettingStarted/GettingStarted.lvclass", "Name"="PicoG-App.lvlib:GettingStarted.lvclass", "Referrer"=path "C:/dev/Vireo/PicoG/PicoG-App/picoG/Init Main Panels.vi"}, {"Path"=path "../../AppDetailPanel/AppDetailPanel.lvclass", "Name"="PicoG-App.lvlib:AppDetailPanel.lvclass", "Referrer"=path "C:/dev/Vireo/PicoG/PicoG-App/picoG/Init Main Panels.vi"}, {"Path"=path "../../PlatformConfigPanel/PlatformConfigPanel.lvclass", "Name"="PicoG-App.lvlib:PlatformConfigPanel.lvclass", "Referrer"=path "C:/dev/Vireo/PicoG/PicoG-App/picoG/Init Main Panels.vi"}, {"Path"=path "../../DeviceDetailPanel/DeviceDetailPanel.lvclass", "Name"="PicoG-App.lvlib:DeviceDetailPanel.lvclass", "Referrer"=path "C:/dev/Vireo/PicoG/PicoG-App/picoG/Init Main Panels.vi"}, {"Path"=path "../picoG.lvclass/picoG.ctl", "Name"="PicoG-App.lvlib:picoG.lvclass:picoG.ctl", "Referrer"=path "C:/dev/Vireo/PicoG/PicoG-App/picoG/Init Main Panels.vi"}, {"Path"=path "<vilib>/IlluminatedG/IG OOPanel/OOPanel/Manager/Create Panel by Type.vi", "Name"="OOPanel.lvlib:Manager.lvclass:Create Panel by Type.vi", "Referrer"=path "C:/dev/Vireo/PicoG/PicoG-App/picoG/Init Main Panels.vi"}, {"Path"=path "C:/dev/Vireo/PicoG/PicoG-App/App Watcher/Ctor.vi", "Name"="PicoG-App.lvlib:App Watcher.lvclass:Ctor.vi", "Referrer"=path "C:/dev/Vireo/PicoG/PicoG-App/App Watcher/Ctor.vi"}, {"Path"=path "../App Watcher.lvclass", "Name"="PicoG-App.lvlib:App Watcher.lvclass", "Referrer"=path "C:/dev/Vireo/PicoG/PicoG-App/App Watcher/Ctor.vi"}, {"Path"=path "../Ref Data.ctl", "Name"="PicoG-App.lvlib:App Watcher.lvclass:Ref Data.ctl", "Referrer"=path "C:/dev/Vireo/PicoG/PicoG-App/App Watcher/Ctor.vi"}, {"Path"=path "../../ViaApp/ViaApp.lvclass", "Name"="PicoG-App.lvlib:ViaApp.lvclass", "Referrer"=path "C:/dev/Vireo/PicoG/PicoG-App/App Watcher/Ctor.vi"}, {"Path"=path "../App Update Data.ctl", "Name"="PicoG-App.lvlib:App Watcher.lvclass:App Update Data.ctl", "Referrer"=path "C:/dev/Vireo/PicoG/PicoG-App/App Watcher/Ctor.vi"}, {"Path"=path "../App Watcher.lvclass/App Watcher.ctl", "Name"="PicoG-App.lvlib:App Watcher.lvclass:App Watcher.ctl", "Referrer"=path "C:/dev/Vireo/PicoG/PicoG-App/App Watcher/Ctor.vi"}, {"Path"=path "C:/dev/Vireo/PicoG/PicoG-App/App Watcher/Set Update Event.vi", "Name"="PicoG-App.lvlib:App Watcher.lvclass:Set Update Event.vi", "Referrer"=path "C:/dev/Vireo/PicoG/PicoG-App/App Watcher/Set Update Event.vi"}, {"Path"=path "../App Watcher.lvclass", "Name"="PicoG-App.lvlib:App Watcher.lvclass", "Referrer"=path "C:/dev/Vireo/PicoG/PicoG-App/App Watcher/Set Update Event.vi"}, {"Path"=path "../App Update Data.ctl", "Name"="PicoG-App.lvlib:App Watcher.lvclass:App Update Data.ctl", "Referrer"=path "C:/dev/Vireo/PicoG/PicoG-App/App Watcher/Set Update Event.vi"}, {"Path"=path "../../ViaApp/ViaApp.lvclass", "Name"="PicoG-App.lvlib:ViaApp.lvclass", "Referrer"=path "C:/dev/Vireo/PicoG/PicoG-App/App Watcher/Set Update Event.vi"}, {"Path"=path "../App Watcher.lvclass/App Watcher.ctl", "Name"="PicoG-App.lvlib:App Watcher.lvclass:App Watcher.ctl", "Referrer"=path "C:/dev/Vireo/PicoG/PicoG-App/App Watcher/Set Update Event.vi"}, {"Path"=path "C:/dev/Vireo/PicoG/PicoG-App/picoG/Check Configs Exist.vi", "Name"="PicoG-App.lvlib:picoG.lvclass:Check Configs Exist.vi", "Referrer"=path "C:/dev/Vireo/PicoG/PicoG-App/picoG/Check Configs Exist.vi"}, {"Path"=path "../picoG.lvclass", "Name"="PicoG-App.lvlib:picoG.lvclass", "Referrer"=path "C:/dev/Vireo/PicoG/PicoG-App/picoG/Check Configs Exist.vi"}, {"Path"=path "../../Config Paths.vi", "Name"="PicoG-App.lvlib:Config Paths.vi", "Referrer"=path "C:/dev/Vireo/PicoG/PicoG-App/picoG/Check Configs Exist.vi"}, {"Path"=path "../Create Default User Config.vi", "Name"="PicoG-App.lvlib:picoG.lvclass:Create Default User Config.vi", "Referrer"=path "C:/dev/Vireo/PicoG/PicoG-App/picoG/Check Configs Exist.vi"}, {"Path"=path "../Create Default System Config.vi", "Name"="PicoG-App.lvlib:picoG.lvclass:Create Default System Config.vi", "Referrer"=path "C:/dev/Vireo/PicoG/PicoG-App/picoG/Check Configs Exist.vi"}, {"Path"=path "<vilib>/Utility/error.llb/Error Cluster From Error Code.vi", "Name"="Error Cluster From Error Code.vi", "Referrer"=path "C:/dev/Vireo/PicoG/PicoG-App/picoG/Check Configs Exist.vi"}, {"Path"=path "C:/dev/Vireo/PicoG/PicoG-App/picoG/Load Platform Config.vi", "Name"="PicoG-App.lvlib:picoG.lvclass:Load Platform Config.vi", "Referrer"=path "C:/dev/Vireo/PicoG/PicoG-App/picoG/Load Platform Config.vi"}, {"Path"=path "../picoG.lvclass", "Name"="PicoG-App.lvlib:picoG.lvclass", "Referrer"=path "C:/dev/Vireo/PicoG/PicoG-App/picoG/Load Platform Config.vi"}, {"Path"=path "C:/dev/Vireo/PicoG/PicoG-App/picoG/Load User Devices.vi", "Name"="PicoG-App.lvlib:picoG.lvclass:Load User Devices.vi", "Referrer"=path "C:/dev/Vireo/PicoG/PicoG-App/picoG/Load User Devices.vi"}, {"Path"=path "../picoG.lvclass", "Name"="PicoG-App.lvlib:picoG.lvclass", "Referrer"=path "C:/dev/Vireo/PicoG/PicoG-App/picoG/Load User Devices.vi"}, {"Path"=path "../picoG.lvclass/picoG.ctl", "Name"="PicoG-App.lvlib:picoG.lvclass:picoG.ctl", "Referrer"=path "C:/dev/Vireo/PicoG/PicoG-App/picoG/Load User Devices.vi"}, {"Path"=path "../Read User Devices.vi", "Name"="PicoG-App.lvlib:picoG.lvclass:Read User Devices.vi", "Referrer"=path "C:/dev/Vireo/PicoG/PicoG-App/picoG/Load User Devices.vi"}, {"Path"=path "../../DeviceListPanel/Add Device.vi", "Name"="PicoG-App.lvlib:DeviceListPanel.lvclass:Add Device.vi", "Referrer"=path "C:/dev/Vireo/PicoG/PicoG-App/picoG/Load User Devices.vi"}, {"Path"=path "C:/dev/Vireo/PicoG/PicoG-App/picoG/Load User Apps.vi", "Name"="PicoG-App.lvlib:picoG.lvclass:Load User Apps.vi", "Referrer"=path "C:/dev/Vireo/PicoG/PicoG-App/picoG/Load User Apps.vi"}, {"Path"=path "../picoG.lvclass", "Name"="PicoG-App.lvlib:picoG.lvclass", "Referrer"=path "C:/dev/Vireo/PicoG/PicoG-App/picoG/Load User Apps.vi"}, {"Path"=path "../picoG.lvclass/picoG.ctl", "Name"="PicoG-App.lvlib:picoG.lvclass:picoG.ctl", "Referrer"=path "C:/dev/Vireo/PicoG/PicoG-App/picoG/Load User Apps.vi"}, {"Path"=path "../Read User Apps.vi", "Name"="PicoG-App.lvlib:picoG.lvclass:Read User Apps.vi", "Referrer"=path "C:/dev/Vireo/PicoG/PicoG-App/picoG/Load User Apps.vi"}, {"Path"=path "../../ViaApp/Init.vi", "Name"="PicoG-App.lvlib:ViaApp.lvclass:Init.vi", "Referrer"=path "C:/dev/Vireo/PicoG/PicoG-App/picoG/Load User Apps.vi"}, {"Path"=path "../../AppListPanel/Update App.vi", "Name"="PicoG-App.lvlib:AppListPanel.lvclass:Update App.vi", "Referrer"=path "C:/dev/Vireo/PicoG/PicoG-App/picoG/Load User Apps.vi"}, {"Path"=path "../../App Watcher/Add App.vi", "Name"="PicoG-App.lvlib:App Watcher.lvclass:Add App.vi", "Referrer"=path "C:/dev/Vireo/PicoG/PicoG-App/picoG/Load User Apps.vi"}, {"Path"=path "C:/dev/Vireo/PicoG/PicoG-App/picoG/Load User Preferences.vi", "Name"="PicoG-App.lvlib:picoG.lvclass:Load User Preferences.vi", "Referrer"=path "C:/dev/Vireo/PicoG/PicoG-App/picoG/Load User Preferences.vi"}, {"Path"=path "../picoG.lvclass", "Name"="PicoG-App.lvlib:picoG.lvclass", "Referrer"=path "C:/dev/Vireo/PicoG/PicoG-App/picoG/Load User Preferences.vi"}, {"Path"=path "C:/dev/Vireo/PicoG/PicoG-App/picoG/UI State.ctl", "Name"="PicoG-App.lvlib:picoG.lvclass:UI State.ctl", "Referrer"=path "C:/dev/Vireo/PicoG/PicoG-App/picoG/UI State.ctl"}, {"Path"=path "../picoG.lvclass", "Name"="PicoG-App.lvlib:picoG.lvclass", "Referrer"=path "C:/dev/Vireo/PicoG/PicoG-App/picoG/UI State.ctl"}, {"Path"=path "C:/dev/Vireo/PicoG/PicoG-App/picoG/Close Splash.vi", "Name"="PicoG-App.lvlib:picoG.lvclass:Close Splash.vi", "Referrer"=path "C:/dev/Vireo/PicoG/PicoG-App/picoG/Close Splash.vi"}, {"Path"=path "../picoG.lvclass", "Name"="PicoG-App.lvlib:picoG.lvclass", "Referrer"=path "C:/dev/Vireo/PicoG/PicoG-App/picoG/Close Splash.vi"}, {"Path"=path "../picoG.lvclass/picoG.ctl", "Name"="PicoG-App.lvlib:picoG.lvclass:picoG.ctl", "Referrer"=path "C:/dev/Vireo/PicoG/PicoG-App/picoG/Close Splash.vi"}, {"Path"=path "C:/dev/Vireo/PicoG/PicoG-App/picoG/_Add App.vi", "Name"="PicoG-App.lvlib:picoG.lvclass:_Add App.vi", "Referrer"=path "C:/dev/Vireo/PicoG/PicoG-App/picoG/_Add App.vi"}, {"Path"=path "../picoG.lvclass", "Name"="PicoG-App.lvlib:picoG.lvclass", "Referrer"=path "C:/dev/Vireo/PicoG/PicoG-App/picoG/_Add App.vi"}, {"Path"=path "../picoG.lvclass/picoG.ctl", "Name"="PicoG-App.lvlib:picoG.lvclass:picoG.ctl", "Referrer"=path "C:/dev/Vireo/PicoG/PicoG-App/picoG/_Add App.vi"}, {"Path"=path "4267f4de-baa5-4d76-a96e-fc062378f624.vi", "Name"="PicoG-App.lvlib:picoG.lvclass:_Add App.vi:Instance:4267f4de-baa5-4d76-a96e-fc062378f624.vi", "Referrer"=path "C:/dev/Vireo/PicoG/PicoG-App/picoG/_Add App.vi"}, {"Path"=path "0", "Name"="PicoG-App.lvlib:picoG.lvclass:_Add App.vi:Instance:0", "Referrer"=path "C:/dev/Vireo/PicoG/PicoG-App/picoG/_Add App.vi"}, {"Path"=path "../../ViaApp/Init.vi", "Name"="PicoG-App.lvlib:ViaApp.lvclass:Init.vi", "Referrer"=path "C:/dev/Vireo/PicoG/PicoG-App/picoG/_Add App.vi"}, {"Path"=path "../../App Watcher/Add App.vi", "Name"="PicoG-App.lvlib:App Watcher.lvclass:Add App.vi", "Referrer"=path "C:/dev/Vireo/PicoG/PicoG-App/picoG/_Add App.vi"}, {"Path"=path "../../AppListPanel/Update App.vi", "Name"="PicoG-App.lvlib:AppListPanel.lvclass:Update App.vi", "Referrer"=path "C:/dev/Vireo/PicoG/PicoG-App/picoG/_Add App.vi"}, {"Path"=path "C:/dev/Vireo/PicoG/PicoG-App/picoG/Top VI FG.vi", "Name"="PicoG-App.lvlib:Top VI FG.vi", "Referrer"=path "C:/dev/Vireo/PicoG/PicoG-App/picoG/Top VI FG.vi"}, {"Path"=path "../../PicoG-App.lvlib", "Name"="PicoG-App.lvlib", "Referrer"=path "C:/dev/Vireo/PicoG/PicoG-App/picoG/Top VI FG.vi"}, {"Path"=path "C:/dev/Vireo/PicoG/PicoG-App/AppListPanel/Update App.vi", "Name"="PicoG-App.lvlib:AppListPanel.lvclass:Update App.vi", "Referrer"=path "C:/dev/Vireo/PicoG/PicoG-App/AppListPanel/Update App.vi"}, {"Path"=path "../AppListPanel.lvclass", "Name"="PicoG-App.lvlib:AppListPanel.lvclass", "Referrer"=path "C:/dev/Vireo/PicoG/PicoG-App/AppListPanel/Update App.vi"}, {"Path"=path "../../ViaApp/ViaApp.lvclass", "Name"="PicoG-App.lvlib:ViaApp.lvclass", "Referrer"=path "C:/dev/Vireo/PicoG/PicoG-App/AppListPanel/Update App.vi"}, {"Path"=path "../AppListPanel.lvclass/AppListPanel.ctl", "Name"="PicoG-App.lvlib:AppListPanel.lvclass:AppListPanel.ctl", "Referrer"=path "C:/dev/Vireo/PicoG/PicoG-App/AppListPanel/Update App.vi"}, {"Path"=path "C:/dev/Vireo/PicoG/PicoG-App/picoG/Save Config.vi", "Name"="PicoG-App.lvlib:picoG.lvclass:Save Config.vi", "Referrer"=path "C:/dev/Vireo/PicoG/PicoG-App/picoG/Save Config.vi"}, {"Path"=path "../picoG.lvclass", "Name"="PicoG-App.lvlib:picoG.lvclass", "Referrer"=path "C:/dev/Vireo/PicoG/PicoG-App/picoG/Save Config.vi"}, {"Path"=path "../Save User Apps.vi", "Name"="PicoG-App.lvlib:picoG.lvclass:Save User Apps.vi", "Referrer"=path "C:/dev/Vireo/PicoG/PicoG-App/picoG/Save Config.vi"}, {"Path"=path "../Save User Devices.vi", "Name"="PicoG-App.lvlib:picoG.lvclass:Save User Devices.vi", "Referrer"=path "C:/dev/Vireo/PicoG/PicoG-App/picoG/Save Config.vi"}, {"Path"=path "C:/dev/Vireo/PicoG/PicoG-App/AppListPanel/Select App.vi", "Name"="PicoG-App.lvlib:AppListPanel.lvclass:Select App.vi", "Referrer"=path "C:/dev/Vireo/PicoG/PicoG-App/AppListPanel/Select App.vi"}, {"Path"=path "../AppListPanel.lvclass", "Name"="PicoG-App.lvlib:AppListPanel.lvclass", "Referrer"=path "C:/dev/Vireo/PicoG/PicoG-App/AppListPanel/Select App.vi"}, {"Path"=path "../../ViaApp/ViaApp.lvclass", "Name"="PicoG-App.lvlib:ViaApp.lvclass", "Referrer"=path "C:/dev/Vireo/PicoG/PicoG-App/AppListPanel/Select App.vi"}, {"Path"=path "../../GWebAppArrayPanel/GWebAppArrayPanel.lvclass", "Name"="PicoG-App.lvlib:GWebAppArrayPanel.lvclass", "Referrer"=path "C:/dev/Vireo/PicoG/PicoG-App/AppListPanel/Select App.vi"}, {"Path"=path "../AppListPanel.lvclass/AppListPanel.ctl", "Name"="PicoG-App.lvlib:AppListPanel.lvclass:AppListPanel.ctl", "Referrer"=path "C:/dev/Vireo/PicoG/PicoG-App/AppListPanel/Select App.vi"}, {"Path"=path "<vilib>/IlluminatedG/IG OOPanel/OOPanel/ArrayManager/Get All Panels.vi", "Name"="OOPanel.lvlib:ArrayManager.lvclass:Get All Panels.vi", "Referrer"=path "C:/dev/Vireo/PicoG/PicoG-App/AppListPanel/Select App.vi"}, {"Path"=path "../../ViaApp/Get Path.vi", "Name"="PicoG-App.lvlib:ViaApp.lvclass:Get Path.vi", "Referrer"=path "C:/dev/Vireo/PicoG/PicoG-App/AppListPanel/Select App.vi"}, {"Path"=path "../../GWebAppArrayPanel/Get Via App.vi", "Name"="PicoG-App.lvlib:GWebAppArrayPanel.lvclass:Get Via App.vi", "Referrer"=path "C:/dev/Vireo/PicoG/PicoG-App/AppListPanel/Select App.vi"}, {"Path"=path "../../GWebAppArrayPanel/Set Highlighted.vi", "Name"="PicoG-App.lvlib:GWebAppArrayPanel.lvclass:Set Highlighted.vi", "Referrer"=path "C:/dev/Vireo/PicoG/PicoG-App/AppListPanel/Select App.vi"}, {"Path"=path "C:/dev/Vireo/PicoG/PicoG-App/PlatformListPanel/Deselect Platform.vi", "Name"="PicoG-App.lvlib:PlatformListPanel.lvclass:Deselect Platform.vi", "Referrer"=path "C:/dev/Vireo/PicoG/PicoG-App/PlatformListPanel/Deselect Platform.vi"}, {"Path"=path "../PlatformListPanel.lvclass", "Name"="PicoG-App.lvlib:PlatformListPanel.lvclass", "Referrer"=path "C:/dev/Vireo/PicoG/PicoG-App/PlatformListPanel/Deselect Platform.vi"}, {"Path"=path "../PlatformListPanel.lvclass/PlatformListPanel.ctl", "Name"="PicoG-App.lvlib:PlatformListPanel.lvclass:PlatformListPanel.ctl", "Referrer"=path "C:/dev/Vireo/PicoG/PicoG-App/PlatformListPanel/Deselect Platform.vi"}, {"Path"=path "../../PlatformArrayPanel/PlatformArrayPanel.lvclass", "Name"="PicoG-App.lvlib:PlatformArrayPanel.lvclass", "Referrer"=path "C:/dev/Vireo/PicoG/PicoG-App/PlatformListPanel/Deselect Platform.vi"}, {"Path"=path "<vilib>/IlluminatedG/IG OOPanel/OOPanel/ArrayManager/Get All Panels.vi", "Name"="OOPanel.lvlib:ArrayManager.lvclass:Get All Panels.vi", "Referrer"=path "C:/dev/Vireo/PicoG/PicoG-App/PlatformListPanel/Deselect Platform.vi"}, {"Path"=path "../../PlatformArrayPanel/Set Highlighted.vi", "Name"="PicoG-App.lvlib:PlatformArrayPanel.lvclass:Set Highlighted.vi", "Referrer"=path "C:/dev/Vireo/PicoG/PicoG-App/PlatformListPanel/Deselect Platform.vi"}, {"Path"=path "C:/dev/Vireo/PicoG/PicoG-App/PlatformListPanel/Select Platform.vi", "Name"="PicoG-App.lvlib:PlatformListPanel.lvclass:Select Platform.vi", "Referrer"=path "C:/dev/Vireo/PicoG/PicoG-App/PlatformListPanel/Select Platform.vi"}, {"Path"=path "../PlatformListPanel.lvclass", "Name"="PicoG-App.lvlib:PlatformListPanel.lvclass", "Referrer"=path "C:/dev/Vireo/PicoG/PicoG-App/PlatformListPanel/Select Platform.vi"}, {"Path"=path "../../../Builds/picoG/ppl/PicoG-Core.lvlibp/PicoG-Processor/PicoG-Core/Platform/Platform.lvclass", "Name"="PicoG-Core.lvlibp:Platform.lvclass", "Referrer"=path "C:/dev/Vireo/PicoG/PicoG-App/PlatformListPanel/Select Platform.vi"}, {"Path"=path "../PlatformListPanel.lvclass/PlatformListPanel.ctl", "Name"="PicoG-App.lvlib:PlatformListPanel.lvclass:PlatformListPanel.ctl", "Referrer"=path "C:/dev/Vireo/PicoG/PicoG-App/PlatformListPanel/Select Platform.vi"}, {"Path"=path "../../PlatformArrayPanel/PlatformArrayPanel.lvclass", "Name"="PicoG-App.lvlib:PlatformArrayPanel.lvclass", "Referrer"=path "C:/dev/Vireo/PicoG/PicoG-App/PlatformListPanel/Select Platform.vi"}, {"Path"=path "<vilib>/IlluminatedG/IG OOPanel/OOPanel/ArrayManager/Get All Panels.vi", "Name"="OOPanel.lvlib:ArrayManager.lvclass:Get All Panels.vi", "Referrer"=path "C:/dev/Vireo/PicoG/PicoG-App/PlatformListPanel/Select Platform.vi"}, {"Path"=path "../../PlatformArrayPanel/Get Platform.vi", "Name"="PicoG-App.lvlib:PlatformArrayPanel.lvclass:Get Platform.vi", "Referrer"=path "C:/dev/Vireo/PicoG/PicoG-App/PlatformListPanel/Select Platform.vi"}, {"Path"=path "../../PlatformArrayPanel/Set Highlighted.vi", "Name"="PicoG-App.lvlib:PlatformArrayPanel.lvclass:Set Highlighted.vi", "Referrer"=path "C:/dev/Vireo/PicoG/PicoG-App/PlatformListPanel/Select Platform.vi"}, {"Path"=path "C:/dev/Vireo/PicoG/PicoG-App/AppListPanel/Deselect Apps.vi", "Name"="PicoG-App.lvlib:AppListPanel.lvclass:Deselect Apps.vi", "Referrer"=path "C:/dev/Vireo/PicoG/PicoG-App/AppListPanel/Deselect Apps.vi"}, {"Path"=path "../AppListPanel.lvclass", "Name"="PicoG-App.lvlib:AppListPanel.lvclass", "Referrer"=path "C:/dev/Vireo/PicoG/PicoG-App/AppListPanel/Deselect Apps.vi"}, {"Path"=path "../AppListPanel.lvclass/AppListPanel.ctl", "Name"="PicoG-App.lvlib:AppListPanel.lvclass:AppListPanel.ctl", "Referrer"=path "C:/dev/Vireo/PicoG/PicoG-App/AppListPanel/Deselect Apps.vi"}, {"Path"=path "../../GWebAppArrayPanel/GWebAppArrayPanel.lvclass", "Name"="PicoG-App.lvlib:GWebAppArrayPanel.lvclass", "Referrer"=path "C:/dev/Vireo/PicoG/PicoG-App/AppListPanel/Deselect Apps.vi"}, {"Path"=path "<vilib>/IlluminatedG/IG OOPanel/OOPanel/ArrayManager/Get All Panels.vi", "Name"="OOPanel.lvlib:ArrayManager.lvclass:Get All Panels.vi", "Referrer"=path "C:/dev/Vireo/PicoG/PicoG-App/AppListPanel/Deselect Apps.vi"}, {"Path"=path "../../GWebAppArrayPanel/Set Highlighted.vi", "Name"="PicoG-App.lvlib:GWebAppArrayPanel.lvclass:Set Highlighted.vi", "Referrer"=path "C:/dev/Vireo/PicoG/PicoG-App/AppListPanel/Deselect Apps.vi"}, {"Path"=path "C:/dev/Vireo/PicoG/PicoG-App/AppDetailPanel/Set App.vi", "Name"="PicoG-App.lvlib:AppDetailPanel.lvclass:Set App.vi", "Referrer"=path "C:/dev/Vireo/PicoG/PicoG-App/AppDetailPanel/Set App.vi"}, {"Path"=path "../AppDetailPanel.lvclass", "Name"="PicoG-App.lvlib:AppDetailPanel.lvclass", "Referrer"=path "C:/dev/Vireo/PicoG/PicoG-App/AppDetailPanel/Set App.vi"}, {"Path"=path "../../ViaApp/ViaApp.lvclass", "Name"="PicoG-App.lvlib:ViaApp.lvclass", "Referrer"=path "C:/dev/Vireo/PicoG/PicoG-App/AppDetailPanel/Set App.vi"}, {"Path"=path "../AppDetailPanel.lvclass/AppDetailPanel.ctl", "Name"="PicoG-App.lvlib:AppDetailPanel.lvclass:AppDetailPanel.ctl", "Referrer"=path "C:/dev/Vireo/PicoG/PicoG-App/AppDetailPanel/Set App.vi"}, {"Path"=path "C:/dev/Vireo/PicoG/PicoG-App/AppListPanel/Panel.vi", "Name"="PicoG-App.lvlib:AppListPanel.lvclass:Panel.vi", "Referrer"=path "C:/dev/Vireo/PicoG/PicoG-App/AppListPanel/Panel.vi"}, {"Path"=path "../AppListPanel.lvclass", "Name"="PicoG-App.lvlib:AppListPanel.lvclass", "Referrer"=path "C:/dev/Vireo/PicoG/PicoG-App/AppListPanel/Panel.vi"}, {"Path"=path "../Sort Order.ctl", "Name"="PicoG-App.lvlib:AppListPanel.lvclass:Sort Order.ctl", "Referrer"=path "C:/dev/Vireo/PicoG/PicoG-App/AppListPanel/Panel.vi"}, {"Path"=path "<vilib>/IlluminatedG/IG OOPanel/OOPanel/Panel/Basic UI State.ctl", "Name"="OOPanel.lvlib:Panel.lvclass:Basic UI State.ctl", "Referrer"=path "C:/dev/Vireo/PicoG/PicoG-App/AppListPanel/Panel.vi"}, {"Path"=path "../AppListPanel.lvclass/AppListPanel.ctl", "Name"="PicoG-App.lvlib:AppListPanel.lvclass:AppListPanel.ctl", "Referrer"=path "C:/dev/Vireo/PicoG/PicoG-App/AppListPanel/Panel.vi"}, {"Path"=path "../../GWebAppArrayPanel/GWebAppArrayPanel.lvclass", "Name"="PicoG-App.lvlib:GWebAppArrayPanel.lvclass", "Referrer"=path "C:/dev/Vireo/PicoG/PicoG-App/AppListPanel/Panel.vi"}, {"Path"=path "<vilib>/IlluminatedG/IG OOPanel/OOPanel/ArrayManager/Start.vi", "Name"="OOPanel.lvlib:ArrayManager.lvclass:Start.vi", "Referrer"=path "C:/dev/Vireo/PicoG/PicoG-App/AppListPanel/Panel.vi"}, {"Path"=path "<vilib>/IlluminatedG/IG OOPanel/OOPanel/ArrayManager/Set Background.vi", "Name"="OOPanel.lvlib:ArrayManager.lvclass:Set Background.vi", "Referrer"=path "C:/dev/Vireo/PicoG/PicoG-App/AppListPanel/Panel.vi"}, {"Path"=path "<vilib>/IlluminatedG/IG OOPanel/OOPanel/Panel/Get Panel Events.vi", "Name"="OOPanel.lvlib:Panel.lvclass:Get Panel Events.vi", "Referrer"=path "C:/dev/Vireo/PicoG/PicoG-App/AppListPanel/Panel.vi"}, {"Path"=path "<vilib>/IlluminatedG/IG OOPanel/OOPanel/Panel/Set Running.vi", "Name"="OOPanel.lvlib:Panel.lvclass:Set Running.vi", "Referrer"=path "C:/dev/Vireo/PicoG/PicoG-App/AppListPanel/Panel.vi"}, {"Path"=path "../Handle Update App.vi", "Name"="PicoG-App.lvlib:AppListPanel.lvclass:Handle Update App.vi", "Referrer"=path "C:/dev/Vireo/PicoG/PicoG-App/AppListPanel/Panel.vi"}, {"Path"=path "../../ViaApp/Get Path.vi", "Name"="PicoG-App.lvlib:ViaApp.lvclass:Get Path.vi", "Referrer"=path "C:/dev/Vireo/PicoG/PicoG-App/AppListPanel/Panel.vi"}, {"Path"=path "<vilib>/IlluminatedG/IG OOPanel/OOPanel/ArrayManager/Remove Panel.vi", "Name"="OOPanel.lvlib:ArrayManager.lvclass:Remove Panel.vi", "Referrer"=path "C:/dev/Vireo/PicoG/PicoG-App/AppListPanel/Panel.vi"}, {"Path"=path "<vilib>/IlluminatedG/IG OOPanel/OOPanel/ArrayManager/Close Panel.vi", "Name"="OOPanel.lvlib:ArrayManager.lvclass:Close Panel.vi", "Referrer"=path "C:/dev/Vireo/PicoG/PicoG-App/AppListPanel/Panel.vi"}, {"Path"=path "../../picoG/Instance.vi", "Name"="PicoG-App.lvlib:picoG.lvclass:Instance.vi", "Referrer"=path "C:/dev/Vireo/PicoG/PicoG-App/AppListPanel/Panel.vi"}, {"Path"=path "../../picoG/Add App.vi", "Name"="PicoG-App.lvlib:picoG.lvclass:Add App.vi", "Referrer"=path "C:/dev/Vireo/PicoG/PicoG-App/AppListPanel/Panel.vi"}, {"Path"=path "<vilib>/IlluminatedG/IG OOPanel/OOPanel/ArrayManager/Refresh.vi", "Name"="OOPanel.lvlib:ArrayManager.lvclass:Refresh.vi", "Referrer"=path "C:/dev/Vireo/PicoG/PicoG-App/AppListPanel/Panel.vi"}, {"Path"=path "<vilib>/IlluminatedG/IG OOPanel/OOPanel/ArrayManager/Empty Array.vi", "Name"="OOPanel.lvlib:ArrayManager.lvclass:Empty Array.vi", "Referrer"=path "C:/dev/Vireo/PicoG/PicoG-App/AppListPanel/Panel.vi"}, {"Path"=path "../Sort Panels.vi", "Name"="PicoG-App.lvlib:AppListPanel.lvclass:Sort Panels.vi", "Referrer"=path "C:/dev/Vireo/PicoG/PicoG-App/AppListPanel/Panel.vi"}, {"Path"=path "<vilib>/IlluminatedG/IG OOPanel/OOPanel/Panel/Visibility Timeout Helper.vi", "Name"="OOPanel.lvlib:Visibility Timeout Helper.vi", "Referrer"=path "C:/dev/Vireo/PicoG/PicoG-App/AppListPanel/Panel.vi"}, {"Path"=path "../../ViaApp/ViaApp.lvclass", "Name"="PicoG-App.lvlib:ViaApp.lvclass", "Referrer"=path "C:/dev/Vireo/PicoG/PicoG-App/AppListPanel/Panel.vi"}, {"Path"=path "C:/dev/Vireo/PicoG/PicoG-App/picoG/Check Broken VIs.vi", "Name"="PicoG-App.lvlib:picoG.lvclass:Check Broken VIs.vi", "Referrer"=path "C:/dev/Vireo/PicoG/PicoG-App/picoG/Check Broken VIs.vi"}, {"Path"=path "../picoG.lvclass", "Name"="PicoG-App.lvlib:picoG.lvclass", "Referrer"=path "C:/dev/Vireo/PicoG/PicoG-App/picoG/Check Broken VIs.vi"}, {"Path"=path "C:/dev/Vireo/PicoG/PicoG-App/picoG/Add Device.vi", "Name"="PicoG-App.lvlib:picoG.lvclass:Add Device.vi", "Referrer"=path "C:/dev/Vireo/PicoG/PicoG-App/picoG/Add Device.vi"}, {"Path"=path "../picoG.lvclass", "Name"="PicoG-App.lvlib:picoG.lvclass", "Referrer"=path "C:/dev/Vireo/PicoG/PicoG-App/picoG/Add Device.vi"}, {"Path"=path "../Select Platform UI.vi", "Name"="PicoG-App.lvlib:picoG.lvclass:Select Platform UI.vi", "Referrer"=path "C:/dev/Vireo/PicoG/PicoG-App/picoG/Add Device.vi"}, {"Path"=path "../../Device/Init.vi", "Name"="PicoG-App.lvlib:Device.lvclass:Init.vi", "Referrer"=path "C:/dev/Vireo/PicoG/PicoG-App/picoG/Add Device.vi"}, {"Path"=path "../../Device/Refresh Device Info.vi", "Name"="PicoG-App.lvlib:Device.lvclass:Refresh Device Info.vi", "Referrer"=path "C:/dev/Vireo/PicoG/PicoG-App/picoG/Add Device.vi"}, {"Path"=path "../Confirm Device UI.vi", "Name"="PicoG-App.lvlib:picoG.lvclass:Confirm Device UI.vi", "Referrer"=path "C:/dev/Vireo/PicoG/PicoG-App/picoG/Add Device.vi"}, {"Path"=path "../../DeviceListPanel/Add Device.vi", "Name"="PicoG-App.lvlib:DeviceListPanel.lvclass:Add Device.vi", "Referrer"=path "C:/dev/Vireo/PicoG/PicoG-App/picoG/Add Device.vi"}, {"Path"=path "../../../Builds/picoG/ppl/PicoG-Core.lvlibp/PicoG-Processor/PicoG-Core/PlatformPluginManager/Platform by Name.vi", "Name"="PicoG-Core.lvlibp:PlatformManager.lvclass:Platform by Name.vi", "Referrer"=path "C:/dev/Vireo/PicoG/PicoG-App/picoG/Add Device.vi"}, {"Path"=path "../../../Builds/picoG/ppl/PicoG-Core.lvlibp/PicoG-Processor/PicoG-Core/Platform/Platform.lvclass", "Name"="PicoG-Core.lvlibp:Platform.lvclass", "Referrer"=path "C:/dev/Vireo/PicoG/PicoG-App/picoG/Add Device.vi"}, {"Path"=path "C:/dev/Vireo/PicoG/PicoG-App/DeviceListPanel/Deselect Devices.vi", "Name"="PicoG-App.lvlib:DeviceListPanel.lvclass:Deselect Devices.vi", "Referrer"=path "C:/dev/Vireo/PicoG/PicoG-App/DeviceListPanel/Deselect Devices.vi"}, {"Path"=path "../DeviceListPanel.lvclass", "Name"="PicoG-App.lvlib:DeviceListPanel.lvclass", "Referrer"=path "C:/dev/Vireo/PicoG/PicoG-App/DeviceListPanel/Deselect Devices.vi"}, {"Path"=path "../DeviceListPanel.lvclass/DeviceListPanel.ctl", "Name"="PicoG-App.lvlib:DeviceListPanel.lvclass:DeviceListPanel.ctl", "Referrer"=path "C:/dev/Vireo/PicoG/PicoG-App/DeviceListPanel/Deselect Devices.vi"}, {"Path"=path "../../DeviceArrayPanel/DeviceArrayPanel.lvclass", "Name"="PicoG-App.lvlib:DeviceArrayPanel.lvclass", "Referrer"=path "C:/dev/Vireo/PicoG/PicoG-App/DeviceListPanel/Deselect Devices.vi"}, {"Path"=path "<vilib>/IlluminatedG/IG OOPanel/OOPanel/ArrayManager/Get All Panels.vi", "Name"="OOPanel.lvlib:ArrayManager.lvclass:Get All Panels.vi", "Referrer"=path "C:/dev/Vireo/PicoG/PicoG-App/DeviceListPanel/Deselect Devices.vi"}, {"Path"=path "../../DeviceArrayPanel/Set Highlighted.vi", "Name"="PicoG-App.lvlib:DeviceArrayPanel.lvclass:Set Highlighted.vi", "Referrer"=path "C:/dev/Vireo/PicoG/PicoG-App/DeviceListPanel/Deselect Devices.vi"}, {"Path"=path "C:/dev/Vireo/PicoG/PicoG-App/DeviceListPanel/Select Device.vi", "Name"="PicoG-App.lvlib:DeviceListPanel.lvclass:Select Device.vi", "Referrer"=path "C:/dev/Vireo/PicoG/PicoG-App/DeviceListPanel/Select Device.vi"}, {"Path"=path "../DeviceListPanel.lvclass", "Name"="PicoG-App.lvlib:DeviceListPanel.lvclass", "Referrer"=path "C:/dev/Vireo/PicoG/PicoG-App/DeviceListPanel/Select Device.vi"}, {"Path"=path "../../Device/Device.lvclass", "Name"="PicoG-App.lvlib:Device.lvclass", "Referrer"=path "C:/dev/Vireo/PicoG/PicoG-App/DeviceListPanel/Select Device.vi"}, {"Path"=path "../DeviceListPanel.lvclass/DeviceListPanel.ctl", "Name"="PicoG-App.lvlib:DeviceListPanel.lvclass:DeviceListPanel.ctl", "Referrer"=path "C:/dev/Vireo/PicoG/PicoG-App/DeviceListPanel/Select Device.vi"}, {"Path"=path "C:/dev/Vireo/PicoG/PicoG-App/DeviceDetailPanel/Set Device.vi", "Name"="PicoG-App.lvlib:DeviceDetailPanel.lvclass:Set Device.vi", "Referrer"=path "C:/dev/Vireo/PicoG/PicoG-App/DeviceDetailPanel/Set Device.vi"}, {"Path"=path "../DeviceDetailPanel.lvclass", "Name"="PicoG-App.lvlib:DeviceDetailPanel.lvclass", "Referrer"=path "C:/dev/Vireo/PicoG/PicoG-App/DeviceDetailPanel/Set Device.vi"}, {"Path"=path "../../Device/Device.lvclass", "Name"="PicoG-App.lvlib:Device.lvclass", "Referrer"=path "C:/dev/Vireo/PicoG/PicoG-App/DeviceDetailPanel/Set Device.vi"}, {"Path"=path "C:/dev/Vireo/PicoG/PicoG-App/AppListPanel/Remove App.vi", "Name"="PicoG-App.lvlib:AppListPanel.lvclass:Remove App.vi", "Referrer"=path "C:/dev/Vireo/PicoG/PicoG-App/AppListPanel/Remove App.vi"}, {"Path"=path "../AppListPanel.lvclass", "Name"="PicoG-App.lvlib:AppListPanel.lvclass", "Referrer"=path "C:/dev/Vireo/PicoG/PicoG-App/AppListPanel/Remove App.vi"}, {"Path"=path "../../ViaApp/ViaApp.lvclass", "Name"="PicoG-App.lvlib:ViaApp.lvclass", "Referrer"=path "C:/dev/Vireo/PicoG/PicoG-App/AppListPanel/Remove App.vi"}, {"Path"=path "../AppListPanel.lvclass/AppListPanel.ctl", "Name"="PicoG-App.lvlib:AppListPanel.lvclass:AppListPanel.ctl", "Referrer"=path "C:/dev/Vireo/PicoG/PicoG-App/AppListPanel/Remove App.vi"}, {"Path"=path "C:/dev/Vireo/PicoG/PicoG-App/App Watcher/Remove App.vi", "Name"="PicoG-App.lvlib:App Watcher.lvclass:Remove App.vi", "Referrer"=path "C:/dev/Vireo/PicoG/PicoG-App/App Watcher/Remove App.vi"}, {"Path"=path "../App Watcher.lvclass", "Name"="PicoG-App.lvlib:App Watcher.lvclass", "Referrer"=path "C:/dev/Vireo/PicoG/PicoG-App/App Watcher/Remove App.vi"}, {"Path"=path "../../ViaApp/ViaApp.lvclass", "Name"="PicoG-App.lvlib:ViaApp.lvclass", "Referrer"=path "C:/dev/Vireo/PicoG/PicoG-App/App Watcher/Remove App.vi"}, {"Path"=path "../App Watcher.lvclass/App Watcher.ctl", "Name"="PicoG-App.lvlib:App Watcher.lvclass:App Watcher.ctl", "Referrer"=path "C:/dev/Vireo/PicoG/PicoG-App/App Watcher/Remove App.vi"}, {"Path"=path "../../ViaApp/Get Path.vi", "Name"="PicoG-App.lvlib:ViaApp.lvclass:Get Path.vi", "Referrer"=path "C:/dev/Vireo/PicoG/PicoG-App/App Watcher/Remove App.vi"}, {"Path"=path "C:/dev/Vireo/PicoG/PicoG-App/DeviceListPanel/Get Devices.vi", "Name"="PicoG-App.lvlib:DeviceListPanel.lvclass:Get Devices.vi", "Referrer"=path "C:/dev/Vireo/PicoG/PicoG-App/DeviceListPanel/Get Devices.vi"}, {"Path"=path "../DeviceListPanel.lvclass", "Name"="PicoG-App.lvlib:DeviceListPanel.lvclass", "Referrer"=path "C:/dev/Vireo/PicoG/PicoG-App/DeviceListPanel/Get Devices.vi"}, {"Path"=path "../../Device/Device.lvclass", "Name"="PicoG-App.lvlib:Device.lvclass", "Referrer"=path "C:/dev/Vireo/PicoG/PicoG-App/DeviceListPanel/Get Devices.vi"}, {"Path"=path "../DeviceListPanel.lvclass/DeviceListPanel.ctl", "Name"="PicoG-App.lvlib:DeviceListPanel.lvclass:DeviceListPanel.ctl", "Referrer"=path "C:/dev/Vireo/PicoG/PicoG-App/DeviceListPanel/Get Devices.vi"}, {"Path"=path "C:/dev/Vireo/PicoG/PicoG-App/AppListPanel/Get Apps.vi", "Name"="PicoG-App.lvlib:AppListPanel.lvclass:Get Apps.vi", "Referrer"=path "C:/dev/Vireo/PicoG/PicoG-App/AppListPanel/Get Apps.vi"}, {"Path"=path "../AppListPanel.lvclass", "Name"="PicoG-App.lvlib:AppListPanel.lvclass", "Referrer"=path "C:/dev/Vireo/PicoG/PicoG-App/AppListPanel/Get Apps.vi"}, {"Path"=path "../../ViaApp/ViaApp.lvclass", "Name"="PicoG-App.lvlib:ViaApp.lvclass", "Referrer"=path "C:/dev/Vireo/PicoG/PicoG-App/AppListPanel/Get Apps.vi"}, {"Path"=path "../AppListPanel.lvclass/AppListPanel.ctl", "Name"="PicoG-App.lvlib:AppListPanel.lvclass:AppListPanel.ctl", "Referrer"=path "C:/dev/Vireo/PicoG/PicoG-App/AppListPanel/Get Apps.vi"}, {"Path"=path "../../GWebAppArrayPanel/GWebAppArrayPanel.lvclass", "Name"="PicoG-App.lvlib:GWebAppArrayPanel.lvclass", "Referrer"=path "C:/dev/Vireo/PicoG/PicoG-App/AppListPanel/Get Apps.vi"}, {"Path"=path "<vilib>/IlluminatedG/IG OOPanel/OOPanel/ArrayManager/Get All Panels.vi", "Name"="OOPanel.lvlib:ArrayManager.lvclass:Get All Panels.vi", "Referrer"=path "C:/dev/Vireo/PicoG/PicoG-App/AppListPanel/Get Apps.vi"}, {"Path"=path "../../GWebAppArrayPanel/Get Via App.vi", "Name"="PicoG-App.lvlib:GWebAppArrayPanel.lvclass:Get Via App.vi", "Referrer"=path "C:/dev/Vireo/PicoG/PicoG-App/AppListPanel/Get Apps.vi"}, {"Path"=path "C:/dev/Vireo/PicoG/PicoG-App/picoG/Main Menu.rtm", "Name"="", "Referrer"=path "C:/dev/Vireo/PicoG/PicoG-App/picoG/Main Menu.rtm"}, {"Path"=path "C:/dev/Vireo/PicoG/PicoG-App/App Watcher/Watcher Loop Async.vi", "Name"="PicoG-App.lvlib:App Watcher.lvclass:Watcher Loop Async.vi", "Referrer"=path "C:/dev/Vireo/PicoG/PicoG-App/App Watcher/Watcher Loop Async.vi"}, {"Path"=path "../App Watcher.lvclass", "Name"="PicoG-App.lvlib:App Watcher.lvclass", "Referrer"=path "C:/dev/Vireo/PicoG/PicoG-App/App Watcher/Watcher Loop Async.vi"}, {"Path"=path "../App Watcher.lvclass/App Watcher.ctl", "Name"="PicoG-App.lvlib:App Watcher.lvclass:App Watcher.ctl", "Referrer"=path "C:/dev/Vireo/PicoG/PicoG-App/App Watcher/Watcher Loop Async.vi"}, {"Path"=path "../Check Apps.vi", "Name"="PicoG-App.lvlib:App Watcher.lvclass:Check Apps.vi", "Referrer"=path "C:/dev/Vireo/PicoG/PicoG-App/App Watcher/Watcher Loop Async.vi"}, {"Path"=path "C:/dev/Vireo/PicoG/PicoG-App/App Watcher/App Watcher.lvclass/App Watcher.ctl", "Name"="PicoG-App.lvlib:App Watcher.lvclass:App Watcher.ctl", "Referrer"=path "C:/dev/Vireo/PicoG/PicoG-App/App Watcher/App Watcher.lvclass/App Watcher.ctl"}, {"Path"=path "..", "Name"="PicoG-App.lvlib:App Watcher.lvclass", "Referrer"=path "C:/dev/Vireo/PicoG/PicoG-App/App Watcher/App Watcher.lvclass/App Watcher.ctl"}, {"Path"=path "../../Ref Data.ctl", "Name"="PicoG-App.lvlib:App Watcher.lvclass:Ref Data.ctl", "Referrer"=path "C:/dev/Vireo/PicoG/PicoG-App/App Watcher/App Watcher.lvclass/App Watcher.ctl"}, {"Path"=path "../../../ViaApp/ViaApp.lvclass", "Name"="PicoG-App.lvlib:ViaApp.lvclass", "Referrer"=path "C:/dev/Vireo/PicoG/PicoG-App/App Watcher/App Watcher.lvclass/App Watcher.ctl"}, {"Path"=path "../../App Update Data.ctl", "Name"="PicoG-App.lvlib:App Watcher.lvclass:App Update Data.ctl", "Referrer"=path "C:/dev/Vireo/PicoG/PicoG-App/App Watcher/App Watcher.lvclass/App Watcher.ctl"}, {"Path"=path "C:/dev/Vireo/PicoG/Builds/picoG/ppl/PicoG-Core.lvlibp/PicoG-Processor/PicoG-Core/PlatformManager/PlatformManager.lvclass/PlatformManager.ctl", "Name"="PicoG-Core.lvlibp:PlatformManager.lvclass:PlatformManager.ctl", "Referrer"=path "C:/dev/Vireo/PicoG/Builds/picoG/ppl/PicoG-Core.lvlibp/PicoG-Processor/PicoG-Core/PlatformManager/PlatformManager.lvclass/PlatformManager.ctl"}, {"Path"=path "..", "Name"="PicoG-Core.lvlibp:PlatformManager.lvclass", "Referrer"=path "C:/dev/Vireo/PicoG/Builds/picoG/ppl/PicoG-Core.lvlibp/PicoG-Processor/PicoG-Core/PlatformManager/PlatformManager.lvclass/PlatformManager.ctl"}, {"Path"=path "../../Ref Data.ctl", "Name"="PicoG-Core.lvlibp:PlatformManager.lvclass:Ref Data.ctl", "Referrer"=path "C:/dev/Vireo/PicoG/Builds/picoG/ppl/PicoG-Core.lvlibp/PicoG-Processor/PicoG-Core/PlatformManager/PlatformManager.lvclass/PlatformManager.ctl"}, {"Path"=path "../../../Platform/Platform.lvclass", "Name"="PicoG-Core.lvlibp:Platform.lvclass", "Referrer"=path "C:/dev/Vireo/PicoG/Builds/picoG/ppl/PicoG-Core.lvlibp/PicoG-Processor/PicoG-Core/PlatformManager/PlatformManager.lvclass/PlatformManager.ctl"}, {"Path"=path "C:/dev/Vireo/PicoG/Builds/picoG/ppl/PicoG-Core.lvlibp/PicoG-Processor/PicoG-Core/PlatformManager/Ref Data.ctl", "Name"="PicoG-Core.lvlibp:PlatformManager.lvclass:Ref Data.ctl", "Referrer"=path "C:/dev/Vireo/PicoG/Builds/picoG/ppl/PicoG-Core.lvlibp/PicoG-Processor/PicoG-Core/PlatformManager/Ref Data.ctl"}, {"Path"=path "../PlatformManager.lvclass", "Name"="PicoG-Core.lvlibp:PlatformManager.lvclass", "Referrer"=path "C:/dev/Vireo/PicoG/Builds/picoG/ppl/PicoG-Core.lvlibp/PicoG-Processor/PicoG-Core/PlatformManager/Ref Data.ctl"}, {"Path"=path "../../Platform/Platform.lvclass", "Name"="PicoG-Core.lvlibp:Platform.lvclass", "Referrer"=path "C:/dev/Vireo/PicoG/Builds/picoG/ppl/PicoG-Core.lvlibp/PicoG-Processor/PicoG-Core/PlatformManager/Ref Data.ctl"}, {"Path"=path "C:/dev/Vireo/PicoG/Builds/picoG/ppl/PicoG-Core.lvlibp/PicoG-Processor/PicoG-Core/PlatformManager/Load Plugins.vi", "Name"="PicoG-Core.lvlibp:PlatformManager.lvclass:Load Plugins.vi", "Referrer"=path "C:/dev/Vireo/PicoG/Builds/picoG/ppl/PicoG-Core.lvlibp/PicoG-Processor/PicoG-Core/PlatformManager/Load Plugins.vi"}, {"Path"=path "../PlatformManager.lvclass", "Name"="PicoG-Core.lvlibp:PlatformManager.lvclass", "Referrer"=path "C:/dev/Vireo/PicoG/Builds/picoG/ppl/PicoG-Core.lvlibp/PicoG-Processor/PicoG-Core/PlatformManager/Load Plugins.vi"}, {"Path"=path "../PlatformManager.lvclass/PlatformManager.ctl", "Name"="PicoG-Core.lvlibp:PlatformManager.lvclass:PlatformManager.ctl", "Referrer"=path "C:/dev/Vireo/PicoG/Builds/picoG/ppl/PicoG-Core.lvlibp/PicoG-Processor/PicoG-Core/PlatformManager/Load Plugins.vi"}, {"Path"=path "../../Platform/Platform.lvclass", "Name"="PicoG-Core.lvlibp:Platform.lvclass", "Referrer"=path "C:/dev/Vireo/PicoG/Builds/picoG/ppl/PicoG-Core.lvlibp/PicoG-Processor/PicoG-Core/PlatformManager/Load Plugins.vi"}, {"Path"=path "../Platform Plugin Folder.vi", "Name"="PicoG-Core.lvlibp:PlatformManager.lvclass:Platform Plugin Folder.vi", "Referrer"=path "C:/dev/Vireo/PicoG/Builds/picoG/ppl/PicoG-Core.lvlibp/PicoG-Processor/PicoG-Core/PlatformManager/Load Plugins.vi"}, {"Path"=path "../../../../1abvi3w/vi.lib/Utility/LVLibp/Get Exported File List.vi", "Name"="PicoG-Core.lvlibp:NI_PackedLibraryUtility.lvlib:Get Exported File List.vi", "Referrer"=path "C:/dev/Vireo/PicoG/Builds/picoG/ppl/PicoG-Core.lvlibp/PicoG-Processor/PicoG-Core/PlatformManager/Load Plugins.vi"}, {"Path"=path "../../../../1abvi3w/vi.lib/Utility/LVClass/Get LV Class Default Value.vi", "Name"="PicoG-Core.lvlibp:Get LV Class Default Value.vi", "Referrer"=path "C:/dev/Vireo/PicoG/Builds/picoG/ppl/PicoG-Core.lvlibp/PicoG-Processor/PicoG-Core/PlatformManager/Load Plugins.vi"}, {"Path"=path "C:/dev/Vireo/PicoG/PicoG-App/AppListPanel/Set Select App Event.vi", "Name"="PicoG-App.lvlib:AppListPanel.lvclass:Set Select App Event.vi", "Referrer"=path "C:/dev/Vireo/PicoG/PicoG-App/AppListPanel/Set Select App Event.vi"}, {"Path"=path "../AppListPanel.lvclass", "Name"="PicoG-App.lvlib:AppListPanel.lvclass", "Referrer"=path "C:/dev/Vireo/PicoG/PicoG-App/AppListPanel/Set Select App Event.vi"}, {"Path"=path "../../ViaApp/ViaApp.lvclass", "Name"="PicoG-App.lvlib:ViaApp.lvclass", "Referrer"=path "C:/dev/Vireo/PicoG/PicoG-App/AppListPanel/Set Select App Event.vi"}, {"Path"=path "../AppListPanel.lvclass/AppListPanel.ctl", "Name"="PicoG-App.lvlib:AppListPanel.lvclass:AppListPanel.ctl", "Referrer"=path "C:/dev/Vireo/PicoG/PicoG-App/AppListPanel/Set Select App Event.vi"}, {"Path"=path "C:/dev/Vireo/PicoG/PicoG-App/DeviceListPanel/Set Select Device Event.vi", "Name"="PicoG-App.lvlib:DeviceListPanel.lvclass:Set Select Device Event.vi", "Referrer"=path "C:/dev/Vireo/PicoG/PicoG-App/DeviceListPanel/Set Select Device Event.vi"}, {"Path"=path "../DeviceListPanel.lvclass", "Name"="PicoG-App.lvlib:DeviceListPanel.lvclass", "Referrer"=path "C:/dev/Vireo/PicoG/PicoG-App/DeviceListPanel/Set Select Device Event.vi"}, {"Path"=path "../../Device/Device.lvclass", "Name"="PicoG-App.lvlib:Device.lvclass", "Referrer"=path "C:/dev/Vireo/PicoG/PicoG-App/DeviceListPanel/Set Select Device Event.vi"}, {"Path"=path "../DeviceListPanel.lvclass/DeviceListPanel.ctl", "Name"="PicoG-App.lvlib:DeviceListPanel.lvclass:DeviceListPanel.ctl", "Referrer"=path "C:/dev/Vireo/PicoG/PicoG-App/DeviceListPanel/Set Select Device Event.vi"}, {"Path"=path "C:/dev/Vireo/PicoG/PicoG-App/DeviceListPanel/Set Add Device Event.vi", "Name"="PicoG-App.lvlib:DeviceListPanel.lvclass:Set Add Device Event.vi", "Referrer"=path "C:/dev/Vireo/PicoG/PicoG-App/DeviceListPanel/Set Add Device Event.vi"}, {"Path"=path "../DeviceListPanel.lvclass", "Name"="PicoG-App.lvlib:DeviceListPanel.lvclass", "Referrer"=path "C:/dev/Vireo/PicoG/PicoG-App/DeviceListPanel/Set Add Device Event.vi"}, {"Path"=path "../DeviceListPanel.lvclass/DeviceListPanel.ctl", "Name"="PicoG-App.lvlib:DeviceListPanel.lvclass:DeviceListPanel.ctl", "Referrer"=path "C:/dev/Vireo/PicoG/PicoG-App/DeviceListPanel/Set Add Device Event.vi"}, {"Path"=path "C:/dev/Vireo/PicoG/PicoG-App/PlatformListPanel/Set Select Platform Event.vi", "Name"="PicoG-App.lvlib:PlatformListPanel.lvclass:Set Select Platform Event.vi", "Referrer"=path "C:/dev/Vireo/PicoG/PicoG-App/PlatformListPanel/Set Select Platform Event.vi"}, {"Path"=path "../PlatformListPanel.lvclass", "Name"="PicoG-App.lvlib:PlatformListPanel.lvclass", "Referrer"=path "C:/dev/Vireo/PicoG/PicoG-App/PlatformListPanel/Set Select Platform Event.vi"}, {"Path"=path "../../../Builds/picoG/ppl/PicoG-Core.lvlibp/PicoG-Processor/PicoG-Core/Platform/Platform.lvclass", "Name"="PicoG-Core.lvlibp:Platform.lvclass", "Referrer"=path "C:/dev/Vireo/PicoG/PicoG-App/PlatformListPanel/Set Select Platform Event.vi"}, {"Path"=path "../PlatformListPanel.lvclass/PlatformListPanel.ctl", "Name"="PicoG-App.lvlib:PlatformListPanel.lvclass:PlatformListPanel.ctl", "Referrer"=path "C:/dev/Vireo/PicoG/PicoG-App/PlatformListPanel/Set Select Platform Event.vi"}, {"Path"=path "C:/dev/Vireo/PicoG/PicoG-App/PlatformListPanel/Set Platform Plugins.vi", "Name"="PicoG-App.lvlib:PlatformListPanel.lvclass:Set Platform Plugins.vi", "Referrer"=path "C:/dev/Vireo/PicoG/PicoG-App/PlatformListPanel/Set Platform Plugins.vi"}, {"Path"=path "../PlatformListPanel.lvclass", "Name"="PicoG-App.lvlib:PlatformListPanel.lvclass", "Referrer"=path "C:/dev/Vireo/PicoG/PicoG-App/PlatformListPanel/Set Platform Plugins.vi"}, {"Path"=path "../../../Builds/picoG/ppl/PicoG-Core.lvlibp/PicoG-Processor/PicoG-Core/PlatformManager/PlatformManager.lvclass", "Name"="PicoG-Core.lvlibp:PlatformManager.lvclass", "Referrer"=path "C:/dev/Vireo/PicoG/PicoG-App/PlatformListPanel/Set Platform Plugins.vi"}, {"Path"=path "../PlatformListPanel.lvclass/PlatformListPanel.ctl", "Name"="PicoG-App.lvlib:PlatformListPanel.lvclass:PlatformListPanel.ctl", "Referrer"=path "C:/dev/Vireo/PicoG/PicoG-App/PlatformListPanel/Set Platform Plugins.vi"}, {"Path"=path "C:/dev/Vireo/PicoG/PicoG-App/App Watcher/Ref Data.ctl", "Name"="PicoG-App.lvlib:App Watcher.lvclass:Ref Data.ctl", "Referrer"=path "C:/dev/Vireo/PicoG/PicoG-App/App Watcher/Ref Data.ctl"}, {"Path"=path "../App Watcher.lvclass", "Name"="PicoG-App.lvlib:App Watcher.lvclass", "Referrer"=path "C:/dev/Vireo/PicoG/PicoG-App/App Watcher/Ref Data.ctl"}, {"Path"=path "../../ViaApp/ViaApp.lvclass", "Name"="PicoG-App.lvlib:ViaApp.lvclass", "Referrer"=path "C:/dev/Vireo/PicoG/PicoG-App/App Watcher/Ref Data.ctl"}, {"Path"=path "../App Update Data.ctl", "Name"="PicoG-App.lvlib:App Watcher.lvclass:App Update Data.ctl", "Referrer"=path "C:/dev/Vireo/PicoG/PicoG-App/App Watcher/Ref Data.ctl"}, {"Path"=path "C:/dev/Vireo/PicoG/PicoG-App/Config Paths.vi", "Name"="PicoG-App.lvlib:Config Paths.vi", "Referrer"=path "C:/dev/Vireo/PicoG/PicoG-App/Config Paths.vi"}, {"Path"=path "../PicoG-App.lvlib", "Name"="PicoG-App.lvlib", "Referrer"=path "C:/dev/Vireo/PicoG/PicoG-App/Config Paths.vi"}, {"Path"=path "../Paths.ctl", "Name"="PicoG-App.lvlib:Paths.ctl", "Referrer"=path "C:/dev/Vireo/PicoG/PicoG-App/Config Paths.vi"}, {"Path"=path "<vilib>/Utility/sysdir.llb/System Directory Type.ctl", "Name"="System Directory Type.ctl", "Referrer"=path "C:/dev/Vireo/PicoG/PicoG-App/Config Paths.vi"}, {"Path"=path "<vilib>/Utility/sysdir.llb/Get System Directory.vi", "Name"="Get System Directory.vi", "Referrer"=path "C:/dev/Vireo/PicoG/PicoG-App/Config Paths.vi"}, {"Path"=path "<vilib>/Utility/libraryn.llb/Create Directory Recursive.vi", "Name"="Create Directory Recursive.vi", "Referrer"=path "C:/dev/Vireo/PicoG/PicoG-App/Config Paths.vi"}, {"Path"=path "<vilib>/Utility/libraryn.llb/Check if File or Folder Exists.vi", "Name"="Check if File or Folder Exists.vi", "Referrer"=path "C:/dev/Vireo/PicoG/PicoG-App/Config Paths.vi"}, {"Path"=path "C:/dev/Vireo/PicoG/PicoG-App/picoG/Create Default User Config.vi", "Name"="PicoG-App.lvlib:picoG.lvclass:Create Default User Config.vi", "Referrer"=path "C:/dev/Vireo/PicoG/PicoG-App/picoG/Create Default User Config.vi"}, {"Path"=path "../picoG.lvclass", "Name"="PicoG-App.lvlib:picoG.lvclass", "Referrer"=path "C:/dev/Vireo/PicoG/PicoG-App/picoG/Create Default User Config.vi"}, {"Path"=path "<vilib>/Utility/config.llb/Open Config Data.vi", "Name"="NI_LVConfig.lvlib:Open Config Data.vi", "Referrer"=path "C:/dev/Vireo/PicoG/PicoG-App/picoG/Create Default User Config.vi"}, {"Path"=path "<vilib>/Utility/config.llb/Write Key.vi", "Name"="NI_LVConfig.lvlib:Write Key.vi", "Referrer"=path "C:/dev/Vireo/PicoG/PicoG-App/picoG/Create Default User Config.vi"}, {"Path"=path "<vilib>/Utility/config.llb/Write Key (I32).vi", "Name"="NI_LVConfig.lvlib:Write Key (I32).vi", "Referrer"=path "C:/dev/Vireo/PicoG/PicoG-App/picoG/Create Default User Config.vi"}, {"Path"=path "<vilib>/Utility/config.llb/Close Config Data.vi", "Name"="NI_LVConfig.lvlib:Close Config Data.vi", "Referrer"=path "C:/dev/Vireo/PicoG/PicoG-App/picoG/Create Default User Config.vi"}, {"Path"=path "C:/dev/Vireo/PicoG/PicoG-App/picoG/Create Default System Config.vi", "Name"="PicoG-App.lvlib:picoG.lvclass:Create Default System Config.vi", "Referrer"=path "C:/dev/Vireo/PicoG/PicoG-App/picoG/Create Default System Config.vi"}, {"Path"=path "../picoG.lvclass", "Name"="PicoG-App.lvlib:picoG.lvclass", "Referrer"=path "C:/dev/Vireo/PicoG/PicoG-App/picoG/Create Default System Config.vi"}, {"Path"=path "<vilib>/Utility/config.llb/Open Config Data.vi", "Name"="NI_LVConfig.lvlib:Open Config Data.vi", "Referrer"=path "C:/dev/Vireo/PicoG/PicoG-App/picoG/Create Default System Config.vi"}, {"Path"=path "<vilib>/Utility/config.llb/Write Key.vi", "Name"="NI_LVConfig.lvlib:Write Key.vi", "Referrer"=path "C:/dev/Vireo/PicoG/PicoG-App/picoG/Create Default System Config.vi"}, {"Path"=path "<vilib>/Utility/config.llb/Write Key (I32).vi", "Name"="NI_LVConfig.lvlib:Write Key (I32).vi", "Referrer"=path "C:/dev/Vireo/PicoG/PicoG-App/picoG/Create Default System Config.vi"}, {"Path"=path "<vilib>/Utility/config.llb/Close Config Data.vi", "Name"="NI_LVConfig.lvlib:Close Config Data.vi", "Referrer"=path "C:/dev/Vireo/PicoG/PicoG-App/picoG/Create Default System Config.vi"}, {"Path"=path "C:/dev/Vireo/PicoG/PicoG-App/picoG/Read User Devices.vi", "Name"="PicoG-App.lvlib:picoG.lvclass:Read User Devices.vi", "Referrer"=path "C:/dev/Vireo/PicoG/PicoG-App/picoG/Read User Devices.vi"}, {"Path"=path "../picoG.lvclass", "Name"="PicoG-App.lvlib:picoG.lvclass", "Referrer"=path "C:/dev/Vireo/PicoG/PicoG-App/picoG/Read User Devices.vi"}, {"Path"=path "../../Device/Device.lvclass", "Name"="PicoG-App.lvlib:Device.lvclass", "Referrer"=path "C:/dev/Vireo/PicoG/PicoG-App/picoG/Read User Devices.vi"}, {"Path"=path "../../Config Paths.vi", "Name"="PicoG-App.lvlib:Config Paths.vi", "Referrer"=path "C:/dev/Vireo/PicoG/PicoG-App/picoG/Read User Devices.vi"}, {"Path"=path "<vilib>/Utility/config.llb/Open Config Data.vi", "Name"="NI_LVConfig.lvlib:Open Config Data.vi", "Referrer"=path "C:/dev/Vireo/PicoG/PicoG-App/picoG/Read User Devices.vi"}, {"Path"=path "<vilib>/Utility/config.llb/Read Key.vi", "Name"="NI_LVConfig.lvlib:Read Key.vi", "Referrer"=path "C:/dev/Vireo/PicoG/PicoG-App/picoG/Read User Devices.vi"}, {"Path"=path "<vilib>/Utility/config.llb/Read Key (I32).vi", "Name"="NI_LVConfig.lvlib:Read Key (I32).vi", "Referrer"=path "C:/dev/Vireo/PicoG/PicoG-App/picoG/Read User Devices.vi"}, {"Path"=path "<vilib>/Utility/config.llb/Get Key Names.vi", "Name"="NI_LVConfig.lvlib:Get Key Names.vi", "Referrer"=path "C:/dev/Vireo/PicoG/PicoG-App/picoG/Read User Devices.vi"}, {"Path"=path "../Read Single Device.vi", "Name"="PicoG-App.lvlib:picoG.lvclass:Read Single Device.vi", "Referrer"=path "C:/dev/Vireo/PicoG/PicoG-App/picoG/Read User Devices.vi"}, {"Path"=path "<vilib>/Utility/config.llb/Close Config Data.vi", "Name"="NI_LVConfig.lvlib:Close Config Data.vi", "Referrer"=path "C:/dev/Vireo/PicoG/PicoG-App/picoG/Read User Devices.vi"}, {"Path"=path "C:/dev/Vireo/PicoG/PicoG-App/DeviceListPanel/Add Device.vi", "Name"="PicoG-App.lvlib:DeviceListPanel.lvclass:Add Device.vi", "Referrer"=path "C:/dev/Vireo/PicoG/PicoG-App/DeviceListPanel/Add Device.vi"}, {"Path"=path "../DeviceListPanel.lvclass", "Name"="PicoG-App.lvlib:DeviceListPanel.lvclass", "Referrer"=path "C:/dev/Vireo/PicoG/PicoG-App/DeviceListPanel/Add Device.vi"}, {"Path"=path "../../Device/Device.lvclass", "Name"="PicoG-App.lvlib:Device.lvclass", "Referrer"=path "C:/dev/Vireo/PicoG/PicoG-App/DeviceListPanel/Add Device.vi"}, {"Path"=path "../DeviceListPanel.lvclass/DeviceListPanel.ctl", "Name"="PicoG-App.lvlib:DeviceListPanel.lvclass:DeviceListPanel.ctl", "Referrer"=path "C:/dev/Vireo/PicoG/PicoG-App/DeviceListPanel/Add Device.vi"}, {"Path"=path "C:/dev/Vireo/PicoG/PicoG-App/picoG/Read User Apps.vi", "Name"="PicoG-App.lvlib:picoG.lvclass:Read User Apps.vi", "Referrer"=path "C:/dev/Vireo/PicoG/PicoG-App/picoG/Read User Apps.vi"}, {"Path"=path "../picoG.lvclass", "Name"="PicoG-App.lvlib:picoG.lvclass", "Referrer"=path "C:/dev/Vireo/PicoG/PicoG-App/picoG/Read User Apps.vi"}, {"Path"=path "../../Config Paths.vi", "Name"="PicoG-App.lvlib:Config Paths.vi", "Referrer"=path "C:/dev/Vireo/PicoG/PicoG-App/picoG/Read User Apps.vi"}, {"Path"=path "<vilib>/Utility/config.llb/Open Config Data.vi", "Name"="NI_LVConfig.lvlib:Open Config Data.vi", "Referrer"=path "C:/dev/Vireo/PicoG/PicoG-App/picoG/Read User Apps.vi"}, {"Path"=path "<vilib>/Utility/config.llb/Read Key.vi", "Name"="NI_LVConfig.lvlib:Read Key.vi", "Referrer"=path "C:/dev/Vireo/PicoG/PicoG-App/picoG/Read User Apps.vi"}, {"Path"=path "<vilib>/Utility/config.llb/Read Key (I32).vi", "Name"="NI_LVConfig.lvlib:Read Key (I32).vi", "Referrer"=path "C:/dev/Vireo/PicoG/PicoG-App/picoG/Read User Apps.vi"}, {"Path"=path "<vilib>/Utility/config.llb/Read Key (Path).vi", "Name"="NI_LVConfig.lvlib:Read Key (Path).vi", "Referrer"=path "C:/dev/Vireo/PicoG/PicoG-App/picoG/Read User Apps.vi"}, {"Path"=path "<vilib>/Utility/config.llb/Close Config Data.vi", "Name"="NI_LVConfig.lvlib:Close Config Data.vi", "Referrer"=path "C:/dev/Vireo/PicoG/PicoG-App/picoG/Read User Apps.vi"}, {"Path"=path "C:/dev/Vireo/PicoG/PicoG-App/ViaApp/Init.vi", "Name"="PicoG-App.lvlib:ViaApp.lvclass:Init.vi", "Referrer"=path "C:/dev/Vireo/PicoG/PicoG-App/ViaApp/Init.vi"}, {"Path"=path "../ViaApp.lvclass", "Name"="PicoG-App.lvlib:ViaApp.lvclass", "Referrer"=path "C:/dev/Vireo/PicoG/PicoG-App/ViaApp/Init.vi"}, {"Path"=path "../ViaApp.lvclass/ViaApp.ctl", "Name"="PicoG-App.lvlib:ViaApp.lvclass:ViaApp.ctl", "Referrer"=path "C:/dev/Vireo/PicoG/PicoG-App/ViaApp/Init.vi"}, {"Path"=path "C:/dev/Vireo/PicoG/PicoG-App/App Watcher/Add App.vi", "Name"="PicoG-App.lvlib:App Watcher.lvclass:Add App.vi", "Referrer"=path "C:/dev/Vireo/PicoG/PicoG-App/App Watcher/Add App.vi"}, {"Path"=path "../App Watcher.lvclass", "Name"="PicoG-App.lvlib:App Watcher.lvclass", "Referrer"=path "C:/dev/Vireo/PicoG/PicoG-App/App Watcher/Add App.vi"}, {"Path"=path "../../ViaApp/ViaApp.lvclass", "Name"="PicoG-App.lvlib:ViaApp.lvclass", "Referrer"=path "C:/dev/Vireo/PicoG/PicoG-App/App Watcher/Add App.vi"}, {"Path"=path "../App Watcher.lvclass/App Watcher.ctl", "Name"="PicoG-App.lvlib:App Watcher.lvclass:App Watcher.ctl", "Referrer"=path "C:/dev/Vireo/PicoG/PicoG-App/App Watcher/Add App.vi"}, {"Path"=path "../../ViaApp/Get Path.vi", "Name"="PicoG-App.lvlib:ViaApp.lvclass:Get Path.vi", "Referrer"=path "C:/dev/Vireo/PicoG/PicoG-App/App Watcher/Add App.vi"}, {"Path"=path "C:/dev/Vireo/PicoG/PicoG-App/AppListPanel/AppListPanel.lvclass/AppListPanel.ctl", "Name"="PicoG-App.lvlib:AppListPanel.lvclass:AppListPanel.ctl", "Referrer"=path "C:/dev/Vireo/PicoG/PicoG-App/AppListPanel/AppListPanel.lvclass/AppListPanel.ctl"}, {"Path"=path "..", "Name"="PicoG-App.lvlib:AppListPanel.lvclass", "Referrer"=path "C:/dev/Vireo/PicoG/PicoG-App/AppListPanel/AppListPanel.lvclass/AppListPanel.ctl"}, {"Path"=path "../../Ref Data.ctl", "Name"="PicoG-App.lvlib:AppListPanel.lvclass:Ref Data.ctl", "Referrer"=path "C:/dev/Vireo/PicoG/PicoG-App/AppListPanel/AppListPanel.lvclass/AppListPanel.ctl"}, {"Path"=path "../../App Panel.ctl", "Name"="PicoG-App.lvlib:AppListPanel.lvclass:App Panel.ctl", "Referrer"=path "C:/dev/Vireo/PicoG/PicoG-App/AppListPanel/AppListPanel.lvclass/AppListPanel.ctl"}, {"Path"=path "../../../ViaApp/ViaApp.lvclass", "Name"="PicoG-App.lvlib:ViaApp.lvclass", "Referrer"=path "C:/dev/Vireo/PicoG/PicoG-App/AppListPanel/AppListPanel.lvclass/AppListPanel.ctl"}, {"Path"=path "../../../GWebAppArrayPanel/GWebAppArrayPanel.lvclass", "Name"="PicoG-App.lvlib:GWebAppArrayPanel.lvclass", "Referrer"=path "C:/dev/Vireo/PicoG/PicoG-App/AppListPanel/AppListPanel.lvclass/AppListPanel.ctl"}, {"Path"=path "<vilib>/IlluminatedG/IG OOPanel/OOPanel/ArrayManager/ArrayManager.lvclass", "Name"="OOPanel.lvlib:ArrayManager.lvclass", "Referrer"=path "C:/dev/Vireo/PicoG/PicoG-App/AppListPanel/AppListPanel.lvclass/AppListPanel.ctl"}, {"Path"=path "../../Inbound Events.ctl", "Name"="PicoG-App.lvlib:AppListPanel.lvclass:Inbound Events.ctl", "Referrer"=path "C:/dev/Vireo/PicoG/PicoG-App/AppListPanel/AppListPanel.lvclass/AppListPanel.ctl"}, {"Path"=path "../../Outbound Events.ctl", "Name"="PicoG-App.lvlib:AppListPanel.lvclass:Outbound Events.ctl", "Referrer"=path "C:/dev/Vireo/PicoG/PicoG-App/AppListPanel/AppListPanel.lvclass/AppListPanel.ctl"}, {"Path"=path "C:/dev/Vireo/PicoG/PicoG-App/picoG/Save User Apps.vi", "Name"="PicoG-App.lvlib:picoG.lvclass:Save User Apps.vi", "Referrer"=path "C:/dev/Vireo/PicoG/PicoG-App/picoG/Save User Apps.vi"}, {"Path"=path "../picoG.lvclass", "Name"="PicoG-App.lvlib:picoG.lvclass", "Referrer"=path "C:/dev/Vireo/PicoG/PicoG-App/picoG/Save User Apps.vi"}, {"Path"=path "../picoG.lvclass/picoG.ctl", "Name"="PicoG-App.lvlib:picoG.lvclass:picoG.ctl", "Referrer"=path "C:/dev/Vireo/PicoG/PicoG-App/picoG/Save User Apps.vi"}, {"Path"=path "../../AppListPanel/Get Apps.vi", "Name"="PicoG-App.lvlib:AppListPanel.lvclass:Get Apps.vi", "Referrer"=path "C:/dev/Vireo/PicoG/PicoG-App/picoG/Save User Apps.vi"}, {"Path"=path "../../Config Paths.vi", "Name"="PicoG-App.lvlib:Config Paths.vi", "Referrer"=path "C:/dev/Vireo/PicoG/PicoG-App/picoG/Save User Apps.vi"}, {"Path"=path "<vilib>/Utility/config.llb/Open Config Data.vi", "Name"="NI_LVConfig.lvlib:Open Config Data.vi", "Referrer"=path "C:/dev/Vireo/PicoG/PicoG-App/picoG/Save User Apps.vi"}, {"Path"=path "<vilib>/Utility/config.llb/Remove Section.vi", "Name"="NI_LVConfig.lvlib:Remove Section.vi", "Referrer"=path "C:/dev/Vireo/PicoG/PicoG-App/picoG/Save User Apps.vi"}, {"Path"=path "<vilib>/Utility/config.llb/Write Key.vi", "Name"="NI_LVConfig.lvlib:Write Key.vi", "Referrer"=path "C:/dev/Vireo/PicoG/PicoG-App/picoG/Save User Apps.vi"}, {"Path"=path "<vilib>/Utility/config.llb/Write Key (I32).vi", "Name"="NI_LVConfig.lvlib:Write Key (I32).vi", "Referrer"=path "C:/dev/Vireo/PicoG/PicoG-App/picoG/Save User Apps.vi"}, {"Path"=path "../../ViaApp/Get Path.vi", "Name"="PicoG-App.lvlib:ViaApp.lvclass:Get Path.vi", "Referrer"=path "C:/dev/Vireo/PicoG/PicoG-App/picoG/Save User Apps.vi"}, {"Path"=path "<vilib>/Utility/config.llb/Write Key (Path).vi", "Name"="NI_LVConfig.lvlib:Write Key (Path).vi", "Referrer"=path "C:/dev/Vireo/PicoG/PicoG-App/picoG/Save User Apps.vi"}, {"Path"=path "<vilib>/Utility/config.llb/Close Config Data.vi", "Name"="NI_LVConfig.lvlib:Close Config Data.vi", "Referrer"=path "C:/dev/Vireo/PicoG/PicoG-App/picoG/Save User Apps.vi"}, {"Path"=path "C:/dev/Vireo/PicoG/PicoG-App/picoG/Save User Devices.vi", "Name"="PicoG-App.lvlib:picoG.lvclass:Save User Devices.vi", "Referrer"=path "C:/dev/Vireo/PicoG/PicoG-App/picoG/Save User Devices.vi"}, {"Path"=path "../picoG.lvclass", "Name"="PicoG-App.lvlib:picoG.lvclass", "Referrer"=path "C:/dev/Vireo/PicoG/PicoG-App/picoG/Save User Devices.vi"}, {"Path"=path "../picoG.lvclass/picoG.ctl", "Name"="PicoG-App.lvlib:picoG.lvclass:picoG.ctl", "Referrer"=path "C:/dev/Vireo/PicoG/PicoG-App/picoG/Save User Devices.vi"}, {"Path"=path "../../DeviceListPanel/Get Devices.vi", "Name"="PicoG-App.lvlib:DeviceListPanel.lvclass:Get Devices.vi", "Referrer"=path "C:/dev/Vireo/PicoG/PicoG-App/picoG/Save User Devices.vi"}, {"Path"=path "../../Config Paths.vi", "Name"="PicoG-App.lvlib:Config Paths.vi", "Referrer"=path "C:/dev/Vireo/PicoG/PicoG-App/picoG/Save User Devices.vi"}, {"Path"=path "<vilib>/Utility/config.llb/Open Config Data.vi", "Name"="NI_LVConfig.lvlib:Open Config Data.vi", "Referrer"=path "C:/dev/Vireo/PicoG/PicoG-App/picoG/Save User Devices.vi"}, {"Path"=path "<vilib>/Utility/config.llb/Remove Section.vi", "Name"="NI_LVConfig.lvlib:Remove Section.vi", "Referrer"=path "C:/dev/Vireo/PicoG/PicoG-App/picoG/Save User Devices.vi"}, {"Path"=path "<vilib>/Utility/config.llb/Write Key.vi", "Name"="NI_LVConfig.lvlib:Write Key.vi", "Referrer"=path "C:/dev/Vireo/PicoG/PicoG-App/picoG/Save User Devices.vi"}, {"Path"=path "<vilib>/Utility/config.llb/Write Key (I32).vi", "Name"="NI_LVConfig.lvlib:Write Key (I32).vi", "Referrer"=path "C:/dev/Vireo/PicoG/PicoG-App/picoG/Save User Devices.vi"}, {"Path"=path "../Write Single Device.vi", "Name"="PicoG-App.lvlib:picoG.lvclass:Write Single Device.vi", "Referrer"=path "C:/dev/Vireo/PicoG/PicoG-App/picoG/Save User Devices.vi"}, {"Path"=path "<vilib>/Utility/config.llb/Close Config Data.vi", "Name"="NI_LVConfig.lvlib:Close Config Data.vi", "Referrer"=path "C:/dev/Vireo/PicoG/PicoG-App/picoG/Save User Devices.vi"}, {"Path"=path "C:/dev/Vireo/PicoG/PicoG-App/GWebAppArrayPanel/GWebAppArrayPanel.lvclass", "Name"="PicoG-App.lvlib:GWebAppArrayPanel.lvclass", "Referrer"=path "C:/dev/Vireo/PicoG/PicoG-App/GWebAppArrayPanel/GWebAppArrayPanel.lvclass"}, {"Path"=path "C:/dev/Vireo/PicoG/PicoG-App/PicoG-App.lvlib", "Name"="PicoG-App.lvlib", "Referrer"=path "C:/dev/Vireo/PicoG/PicoG-App/GWebAppArrayPanel/GWebAppArrayPanel.lvclass"}, {"Path"=path "C:/dev/Vireo/PicoG/PicoG-App/GWebAppArrayPanel/GWebAppArrayPanel.lvclass/GWebAppArrayPanel.ctl", "Name"="PicoG-App.lvlib:GWebAppArrayPanel.lvclass:GWebAppArrayPanel.ctl", "Referrer"=path "C:/dev/Vireo/PicoG/PicoG-App/GWebAppArrayPanel/GWebAppArrayPanel.lvclass"}, {"Path"=path "C:/dev/Vireo/PicoG/PicoG-App/GWebAppArrayPanel/Outbound Events.ctl", "Name"="PicoG-App.lvlib:GWebAppArrayPanel.lvclass:Outbound Events.ctl", "Referrer"=path "C:/dev/Vireo/PicoG/PicoG-App/GWebAppArrayPanel/GWebAppArrayPanel.lvclass"}, {"Path"=path "C:/dev/Vireo/PicoG/PicoG-App/GWebAppArrayPanel/Panel Events.ctl", "Name"="PicoG-App.lvlib:GWebAppArrayPanel.lvclass:Panel Events.ctl", "Referrer"=path "C:/dev/Vireo/PicoG/PicoG-App/GWebAppArrayPanel/GWebAppArrayPanel.lvclass"}, {"Path"=path "C:/dev/Vireo/PicoG/PicoG-App/GWebAppArrayPanel/Ref Data.ctl", "Name"="PicoG-App.lvlib:GWebAppArrayPanel.lvclass:Ref Data.ctl", "Referrer"=path "C:/dev/Vireo/PicoG/PicoG-App/GWebAppArrayPanel/GWebAppArrayPanel.lvclass"}, {"Path"=path "C:/dev/Vireo/PicoG/PicoG-App/GWebAppArrayPanel/Init Events.vi", "Name"="PicoG-App.lvlib:GWebAppArrayPanel.lvclass:Init Events.vi", "Referrer"=path "C:/dev/Vireo/PicoG/PicoG-App/GWebAppArrayPanel/GWebAppArrayPanel.lvclass"}, {"Path"=path "C:/dev/Vireo/PicoG/PicoG-App/GWebAppArrayPanel/Select App.vi", "Name"="PicoG-App.lvlib:GWebAppArrayPanel.lvclass:Select App.vi", "Referrer"=path "C:/dev/Vireo/PicoG/PicoG-App/GWebAppArrayPanel/GWebAppArrayPanel.lvclass"}, {"Path"=path "C:/dev/Vireo/PicoG/PicoG-App/GWebAppArrayPanel/Get Via App.vi", "Name"="PicoG-App.lvlib:GWebAppArrayPanel.lvclass:Get Via App.vi", "Referrer"=path "C:/dev/Vireo/PicoG/PicoG-App/GWebAppArrayPanel/GWebAppArrayPanel.lvclass"}, {"Path"=path "C:/dev/Vireo/PicoG/PicoG-App/GWebAppArrayPanel/Set Via App.vi", "Name"="PicoG-App.lvlib:GWebAppArrayPanel.lvclass:Set Via App.vi", "Referrer"=path "C:/dev/Vireo/PicoG/PicoG-App/GWebAppArrayPanel/GWebAppArrayPanel.lvclass"}, {"Path"=path "C:/dev/Vireo/PicoG/PicoG-App/GWebAppArrayPanel/Get Desired Size.vi", "Name"="PicoG-App.lvlib:GWebAppArrayPanel.lvclass:Get Desired Size.vi", "Referrer"=path "C:/dev/Vireo/PicoG/PicoG-App/GWebAppArrayPanel/GWebAppArrayPanel.lvclass"}, {"Path"=path "C:/dev/Vireo/PicoG/PicoG-App/GWebAppArrayPanel/Set Highlighted.vi", "Name"="PicoG-App.lvlib:GWebAppArrayPanel.lvclass:Set Highlighted.vi", "Referrer"=path "C:/dev/Vireo/PicoG/PicoG-App/GWebAppArrayPanel/GWebAppArrayPanel.lvclass"}, {"Path"=path "C:/dev/Vireo/PicoG/PicoG-App/GWebAppArrayPanel/Set Select Event.vi", "Name"="PicoG-App.lvlib:GWebAppArrayPanel.lvclass:Set Select Event.vi", "Referrer"=path "C:/dev/Vireo/PicoG/PicoG-App/GWebAppArrayPanel/GWebAppArrayPanel.lvclass"}, {"Path"=path "C:/dev/Vireo/PicoG/PicoG-App/GWebAppArrayPanel/Cleanup.vi", "Name"="PicoG-App.lvlib:GWebAppArrayPanel.lvclass:Cleanup.vi", "Referrer"=path "C:/dev/Vireo/PicoG/PicoG-App/GWebAppArrayPanel/GWebAppArrayPanel.lvclass"}, {"Path"=path "C:/dev/Vireo/PicoG/PicoG-App/GWebAppArrayPanel/Ctor.vi", "Name"="PicoG-App.lvlib:GWebAppArrayPanel.lvclass:Ctor.vi", "Referrer"=path "C:/dev/Vireo/PicoG/PicoG-App/GWebAppArrayPanel/GWebAppArrayPanel.lvclass"}, {"Path"=path "C:/dev/Vireo/PicoG/PicoG-App/GWebAppArrayPanel/Panel.vi", "Name"="PicoG-App.lvlib:GWebAppArrayPanel.lvclass:Panel.vi", "Referrer"=path "C:/dev/Vireo/PicoG/PicoG-App/GWebAppArrayPanel/GWebAppArrayPanel.lvclass"}, {"Path"=path "C:/Program Files (x86)/National Instruments/LabVIEW 2020/vi.lib/IlluminatedG/IG OOPanel/OOPanel/ArrayPanel/ArrayPanel.lvclass", "Name"="OOPanel.lvlib:ArrayPanel.lvclass", "Referrer"=path "C:/dev/Vireo/PicoG/PicoG-App/GWebAppArrayPanel/GWebAppArrayPanel.lvclass"}, {"Path"=path "C:/dev/Vireo/PicoG/PicoG-App/ViaApp/Get Path.vi", "Name"="PicoG-App.lvlib:ViaApp.lvclass:Get Path.vi", "Referrer"=path "C:/dev/Vireo/PicoG/PicoG-App/ViaApp/Get Path.vi"}, {"Path"=path "../ViaApp.lvclass", "Name"="PicoG-App.lvlib:ViaApp.lvclass", "Referrer"=path "C:/dev/Vireo/PicoG/PicoG-App/ViaApp/Get Path.vi"}, {"Path"=path "../ViaApp.lvclass/ViaApp.ctl", "Name"="PicoG-App.lvlib:ViaApp.lvclass:ViaApp.ctl", "Referrer"=path "C:/dev/Vireo/PicoG/PicoG-App/ViaApp/Get Path.vi"}, {"Path"=path "C:/dev/Vireo/PicoG/PicoG-App/GWebAppArrayPanel/Get Via App.vi", "Name"="PicoG-App.lvlib:GWebAppArrayPanel.lvclass:Get Via App.vi", "Referrer"=path "C:/dev/Vireo/PicoG/PicoG-App/GWebAppArrayPanel/Get Via App.vi"}, {"Path"=path "../GWebAppArrayPanel.lvclass", "Name"="PicoG-App.lvlib:GWebAppArrayPanel.lvclass", "Referrer"=path "C:/dev/Vireo/PicoG/PicoG-App/GWebAppArrayPanel/Get Via App.vi"}, {"Path"=path "../../ViaApp/ViaApp.lvclass", "Name"="PicoG-App.lvlib:ViaApp.lvclass", "Referrer"=path "C:/dev/Vireo/PicoG/PicoG-App/GWebAppArrayPanel/Get Via App.vi"}, {"Path"=path "../GWebAppArrayPanel.lvclass/GWebAppArrayPanel.ctl", "Name"="PicoG-App.lvlib:GWebAppArrayPanel.lvclass:GWebAppArrayPanel.ctl", "Referrer"=path "C:/dev/Vireo/PicoG/PicoG-App/GWebAppArrayPanel/Get Via App.vi"}, {"Path"=path "C:/dev/Vireo/PicoG/PicoG-App/GWebAppArrayPanel/Set Highlighted.vi", "Name"="PicoG-App.lvlib:GWebAppArrayPanel.lvclass:Set Highlighted.vi", "Referrer"=path "C:/dev/Vireo/PicoG/PicoG-App/GWebAppArrayPanel/Set Highlighted.vi"}, {"Path"=path "../GWebAppArrayPanel.lvclass", "Name"="PicoG-App.lvlib:GWebAppArrayPanel.lvclass", "Referrer"=path "C:/dev/Vireo/PicoG/PicoG-App/GWebAppArrayPanel/Set Highlighted.vi"}, {"Path"=path "../GWebAppArrayPanel.lvclass/GWebAppArrayPanel.ctl", "Name"="PicoG-App.lvlib:GWebAppArrayPanel.lvclass:GWebAppArrayPanel.ctl", "Referrer"=path "C:/dev/Vireo/PicoG/PicoG-App/GWebAppArrayPanel/Set Highlighted.vi"}, {"Path"=path "C:/dev/Vireo/PicoG/PicoG-App/PlatformListPanel/PlatformListPanel.lvclass/PlatformListPanel.ctl", "Name"="PicoG-App.lvlib:PlatformListPanel.lvclass:PlatformListPanel.ctl", "Referrer"=path "C:/dev/Vireo/PicoG/PicoG-App/PlatformListPanel/PlatformListPanel.lvclass/PlatformListPanel.ctl"}, {"Path"=path "..", "Name"="PicoG-App.lvlib:PlatformListPanel.lvclass", "Referrer"=path "C:/dev/Vireo/PicoG/PicoG-App/PlatformListPanel/PlatformListPanel.lvclass/PlatformListPanel.ctl"}, {"Path"=path "<vilib>/IlluminatedG/IG OOPanel/OOPanel/ArrayManager/ArrayManager.lvclass", "Name"="OOPanel.lvlib:ArrayManager.lvclass", "Referrer"=path "C:/dev/Vireo/PicoG/PicoG-App/PlatformListPanel/PlatformListPanel.lvclass/PlatformListPanel.ctl"}, {"Path"=path "../../../../Builds/picoG/ppl/PicoG-Core.lvlibp/PicoG-Processor/PicoG-Core/PlatformManager/PlatformManager.lvclass", "Name"="PicoG-Core.lvlibp:PlatformManager.lvclass", "Referrer"=path "C:/dev/Vireo/PicoG/PicoG-App/PlatformListPanel/PlatformListPanel.lvclass/PlatformListPanel.ctl"}, {"Path"=path "../../../../Builds/picoG/ppl/PicoG-Core.lvlibp/PicoG-Processor/PicoG-Core/Platform/Platform.lvclass", "Name"="PicoG-Core.lvlibp:Platform.lvclass", "Referrer"=path "C:/dev/Vireo/PicoG/PicoG-App/PlatformListPanel/PlatformListPanel.lvclass/PlatformListPanel.ctl"}, {"Path"=path "C:/dev/Vireo/PicoG/PicoG-App/PlatformArrayPanel/PlatformArrayPanel.lvclass", "Name"="PicoG-App.lvlib:PlatformArrayPanel.lvclass", "Referrer"=path "C:/dev/Vireo/PicoG/PicoG-App/PlatformArrayPanel/PlatformArrayPanel.lvclass"}, {"Path"=path "C:/dev/Vireo/PicoG/PicoG-App/PicoG-App.lvlib", "Name"="PicoG-App.lvlib", "Referrer"=path "C:/dev/Vireo/PicoG/PicoG-App/PlatformArrayPanel/PlatformArrayPanel.lvclass"}, {"Path"=path "C:/dev/Vireo/PicoG/PicoG-App/PlatformArrayPanel/PlatformArrayPanel.lvclass/PlatformArrayPanel.ctl", "Name"="PicoG-App.lvlib:PlatformArrayPanel.lvclass:PlatformArrayPanel.ctl", "Referrer"=path "C:/dev/Vireo/PicoG/PicoG-App/PlatformArrayPanel/PlatformArrayPanel.lvclass"}, {"Path"=path "C:/dev/Vireo/PicoG/PicoG-App/PlatformArrayPanel/Outbound Events.ctl", "Name"="PicoG-App.lvlib:PlatformArrayPanel.lvclass:Outbound Events.ctl", "Referrer"=path "C:/dev/Vireo/PicoG/PicoG-App/PlatformArrayPanel/PlatformArrayPanel.lvclass"}, {"Path"=path "C:/dev/Vireo/PicoG/PicoG-App/PlatformArrayPanel/Panel Events.ctl", "Name"="PicoG-App.lvlib:PlatformArrayPanel.lvclass:Panel Events.ctl", "Referrer"=path "C:/dev/Vireo/PicoG/PicoG-App/PlatformArrayPanel/PlatformArrayPanel.lvclass"}, {"Path"=path "C:/dev/Vireo/PicoG/PicoG-App/PlatformArrayPanel/Init Events.vi", "Name"="PicoG-App.lvlib:PlatformArrayPanel.lvclass:Init Events.vi", "Referrer"=path "C:/dev/Vireo/PicoG/PicoG-App/PlatformArrayPanel/PlatformArrayPanel.lvclass"}, {"Path"=path "C:/dev/Vireo/PicoG/PicoG-App/PlatformArrayPanel/Get Desired Size.vi", "Name"="PicoG-App.lvlib:PlatformArrayPanel.lvclass:Get Desired Size.vi", "Referrer"=path "C:/dev/Vireo/PicoG/PicoG-App/PlatformArrayPanel/PlatformArrayPanel.lvclass"}, {"Path"=path "C:/dev/Vireo/PicoG/PicoG-App/PlatformArrayPanel/Set Highlighted.vi", "Name"="PicoG-App.lvlib:PlatformArrayPanel.lvclass:Set Highlighted.vi", "Referrer"=path "C:/dev/Vireo/PicoG/PicoG-App/PlatformArrayPanel/PlatformArrayPanel.lvclass"}, {"Path"=path "C:/dev/Vireo/PicoG/PicoG-App/PlatformArrayPanel/Get Platform.vi", "Name"="PicoG-App.lvlib:PlatformArrayPanel.lvclass:Get Platform.vi", "Referrer"=path "C:/dev/Vireo/PicoG/PicoG-App/PlatformArrayPanel/PlatformArrayPanel.lvclass"}, {"Path"=path "C:/dev/Vireo/PicoG/PicoG-App/PlatformArrayPanel/Set Platform.vi", "Name"="PicoG-App.lvlib:PlatformArrayPanel.lvclass:Set Platform.vi", "Referrer"=path "C:/dev/Vireo/PicoG/PicoG-App/PlatformArrayPanel/PlatformArrayPanel.lvclass"}, {"Path"=path "C:/dev/Vireo/PicoG/PicoG-App/PlatformArrayPanel/Set Select Platform Event.vi", "Name"="PicoG-App.lvlib:PlatformArrayPanel.lvclass:Set Select Platform Event.vi", "Referrer"=path "C:/dev/Vireo/PicoG/PicoG-App/PlatformArrayPanel/PlatformArrayPanel.lvclass"}, {"Path"=path "C:/dev/Vireo/PicoG/PicoG-App/PlatformArrayPanel/Cleanup.vi", "Name"="PicoG-App.lvlib:PlatformArrayPanel.lvclass:Cleanup.vi", "Referrer"=path "C:/dev/Vireo/PicoG/PicoG-App/PlatformArrayPanel/PlatformArrayPanel.lvclass"}, {"Path"=path "C:/dev/Vireo/PicoG/PicoG-App/PlatformArrayPanel/Ctor.vi", "Name"="PicoG-App.lvlib:PlatformArrayPanel.lvclass:Ctor.vi", "Referrer"=path "C:/dev/Vireo/PicoG/PicoG-App/PlatformArrayPanel/PlatformArrayPanel.lvclass"}, {"Path"=path "C:/dev/Vireo/PicoG/PicoG-App/PlatformArrayPanel/Panel.vi", "Name"="PicoG-App.lvlib:PlatformArrayPanel.lvclass:Panel.vi", "Referrer"=path "C:/dev/Vireo/PicoG/PicoG-App/PlatformArrayPanel/PlatformArrayPanel.lvclass"}, {"Path"=path "C:/Program Files (x86)/National Instruments/LabVIEW 2020/vi.lib/IlluminatedG/IG OOPanel/OOPanel/ArrayPanel/ArrayPanel.lvclass", "Name"="OOPanel.lvlib:ArrayPanel.lvclass", "Referrer"=path "C:/dev/Vireo/PicoG/PicoG-App/PlatformArrayPanel/PlatformArrayPanel.lvclass"}, {"Path"=path "C:/dev/Vireo/PicoG/PicoG-App/PlatformArrayPanel/Set Highlighted.vi", "Name"="PicoG-App.lvlib:PlatformArrayPanel.lvclass:Set Highlighted.vi", "Referrer"=path "C:/dev/Vireo/PicoG/PicoG-App/PlatformArrayPanel/Set Highlighted.vi"}, {"Path"=path "../PlatformArrayPanel.lvclass", "Name"="PicoG-App.lvlib:PlatformArrayPanel.lvclass", "Referrer"=path "C:/dev/Vireo/PicoG/PicoG-App/PlatformArrayPanel/Set Highlighted.vi"}, {"Path"=path "../PlatformArrayPanel.lvclass/PlatformArrayPanel.ctl", "Name"="PicoG-App.lvlib:PlatformArrayPanel.lvclass:PlatformArrayPanel.ctl", "Referrer"=path "C:/dev/Vireo/PicoG/PicoG-App/PlatformArrayPanel/Set Highlighted.vi"}, {"Path"=path "C:/dev/Vireo/PicoG/PicoG-App/PlatformArrayPanel/Get Platform.vi", "Name"="PicoG-App.lvlib:PlatformArrayPanel.lvclass:Get Platform.vi", "Referrer"=path "C:/dev/Vireo/PicoG/PicoG-App/PlatformArrayPanel/Get Platform.vi"}, {"Path"=path "../PlatformArrayPanel.lvclass", "Name"="PicoG-App.lvlib:PlatformArrayPanel.lvclass", "Referrer"=path "C:/dev/Vireo/PicoG/PicoG-App/PlatformArrayPanel/Get Platform.vi"}, {"Path"=path "../../../Builds/picoG/ppl/PicoG-Core.lvlibp/PicoG-Processor/PicoG-Core/Platform/Platform.lvclass", "Name"="PicoG-Core.lvlibp:Platform.lvclass", "Referrer"=path "C:/dev/Vireo/PicoG/PicoG-App/PlatformArrayPanel/Get Platform.vi"}, {"Path"=path "../PlatformArrayPanel.lvclass/PlatformArrayPanel.ctl", "Name"="PicoG-App.lvlib:PlatformArrayPanel.lvclass:PlatformArrayPanel.ctl", "Referrer"=path "C:/dev/Vireo/PicoG/PicoG-App/PlatformArrayPanel/Get Platform.vi"}, {"Path"=path "C:/dev/Vireo/PicoG/PicoG-App/AppDetailPanel/AppDetailPanel.lvclass/AppDetailPanel.ctl", "Name"="PicoG-App.lvlib:AppDetailPanel.lvclass:AppDetailPanel.ctl", "Referrer"=path "C:/dev/Vireo/PicoG/PicoG-App/AppDetailPanel/AppDetailPanel.lvclass/AppDetailPanel.ctl"}, {"Path"=path "..", "Name"="PicoG-App.lvlib:AppDetailPanel.lvclass", "Referrer"=path "C:/dev/Vireo/PicoG/PicoG-App/AppDetailPanel/AppDetailPanel.lvclass/AppDetailPanel.ctl"}, {"Path"=path "../../Ref Data.ctl", "Name"="PicoG-App.lvlib:AppDetailPanel.lvclass:Ref Data.ctl", "Referrer"=path "C:/dev/Vireo/PicoG/PicoG-App/AppDetailPanel/AppDetailPanel.lvclass/AppDetailPanel.ctl"}, {"Path"=path "../../../ViaApp/ViaApp.lvclass", "Name"="PicoG-App.lvlib:ViaApp.lvclass", "Referrer"=path "C:/dev/Vireo/PicoG/PicoG-App/AppDetailPanel/AppDetailPanel.lvclass/AppDetailPanel.ctl"}, {"Path"=path "../../Incoming Events.ctl", "Name"="PicoG-App.lvlib:AppDetailPanel.lvclass:Incoming Events.ctl", "Referrer"=path "C:/dev/Vireo/PicoG/PicoG-App/AppDetailPanel/AppDetailPanel.lvclass/AppDetailPanel.ctl"}, {"Path"=path "C:/dev/Vireo/PicoG/PicoG-App/AppListPanel/Sort Order.ctl", "Name"="PicoG-App.lvlib:AppListPanel.lvclass:Sort Order.ctl", "Referrer"=path "C:/dev/Vireo/PicoG/PicoG-App/AppListPanel/Sort Order.ctl"}, {"Path"=path "../AppListPanel.lvclass", "Name"="PicoG-App.lvlib:AppListPanel.lvclass", "Referrer"=path "C:/dev/Vireo/PicoG/PicoG-App/AppListPanel/Sort Order.ctl"}, {"Path"=path "C:/dev/Vireo/PicoG/PicoG-App/AppListPanel/Handle Update App.vi", "Name"="PicoG-App.lvlib:AppListPanel.lvclass:Handle Update App.vi", "Referrer"=path "C:/dev/Vireo/PicoG/PicoG-App/AppListPanel/Handle Update App.vi"}, {"Path"=path "../AppListPanel.lvclass", "Name"="PicoG-App.lvlib:AppListPanel.lvclass", "Referrer"=path "C:/dev/Vireo/PicoG/PicoG-App/AppListPanel/Handle Update App.vi"}, {"Path"=path "../../ViaApp/ViaApp.lvclass", "Name"="PicoG-App.lvlib:ViaApp.lvclass", "Referrer"=path "C:/dev/Vireo/PicoG/PicoG-App/AppListPanel/Handle Update App.vi"}, {"Path"=path "../Sort Order.ctl", "Name"="PicoG-App.lvlib:AppListPanel.lvclass:Sort Order.ctl", "Referrer"=path "C:/dev/Vireo/PicoG/PicoG-App/AppListPanel/Handle Update App.vi"}, {"Path"=path "../AppListPanel.lvclass/AppListPanel.ctl", "Name"="PicoG-App.lvlib:AppListPanel.lvclass:AppListPanel.ctl", "Referrer"=path "C:/dev/Vireo/PicoG/PicoG-App/AppListPanel/Handle Update App.vi"}, {"Path"=path "../../GWebAppArrayPanel/GWebAppArrayPanel.lvclass", "Name"="PicoG-App.lvlib:GWebAppArrayPanel.lvclass", "Referrer"=path "C:/dev/Vireo/PicoG/PicoG-App/AppListPanel/Handle Update App.vi"}, {"Path"=path "../App Panel.ctl", "Name"="PicoG-App.lvlib:AppListPanel.lvclass:App Panel.ctl", "Referrer"=path "C:/dev/Vireo/PicoG/PicoG-App/AppListPanel/Handle Update App.vi"}, {"Path"=path "../../ViaApp/Get Path.vi", "Name"="PicoG-App.lvlib:ViaApp.lvclass:Get Path.vi", "Referrer"=path "C:/dev/Vireo/PicoG/PicoG-App/AppListPanel/Handle Update App.vi"}, {"Path"=path "../../GWebAppArrayPanel/Set Via App.vi", "Name"="PicoG-App.lvlib:GWebAppArrayPanel.lvclass:Set Via App.vi", "Referrer"=path "C:/dev/Vireo/PicoG/PicoG-App/AppListPanel/Handle Update App.vi"}, {"Path"=path "<vilib>/IlluminatedG/IG OOPanel/OOPanel/ArrayManager/Insert Panel.vi", "Name"="OOPanel.lvlib:ArrayManager.lvclass:Insert Panel.vi", "Referrer"=path "C:/dev/Vireo/PicoG/PicoG-App/AppListPanel/Handle Update App.vi"}, {"Path"=path "../../GWebAppArrayPanel/Set Select Event.vi", "Name"="PicoG-App.lvlib:GWebAppArrayPanel.lvclass:Set Select Event.vi", "Referrer"=path "C:/dev/Vireo/PicoG/PicoG-App/AppListPanel/Handle Update App.vi"}, {"Path"=path "../Sort Panels.vi", "Name"="PicoG-App.lvlib:AppListPanel.lvclass:Sort Panels.vi", "Referrer"=path "C:/dev/Vireo/PicoG/PicoG-App/AppListPanel/Handle Update App.vi"}, {"Path"=path "C:/dev/Vireo/PicoG/PicoG-App/picoG/Instance.vi", "Name"="PicoG-App.lvlib:picoG.lvclass:Instance.vi", "Referrer"=path "C:/dev/Vireo/PicoG/PicoG-App/picoG/Instance.vi"}, {"Path"=path "../picoG.lvclass", "Name"="PicoG-App.lvlib:picoG.lvclass", "Referrer"=path "C:/dev/Vireo/PicoG/PicoG-App/picoG/Instance.vi"}, {"Path"=path "../picoG.lvclass/picoG.ctl", "Name"="PicoG-App.lvlib:picoG.lvclass:picoG.ctl", "Referrer"=path "C:/dev/Vireo/PicoG/PicoG-App/picoG/Instance.vi"}, {"Path"=path "../Instance FG.vi", "Name"="PicoG-App.lvlib:picoG.lvclass:Instance FG.vi", "Referrer"=path "C:/dev/Vireo/PicoG/PicoG-App/picoG/Instance.vi"}, {"Path"=path "<vilib>/Utility/error.llb/Error Cluster From Error Code.vi", "Name"="Error Cluster From Error Code.vi", "Referrer"=path "C:/dev/Vireo/PicoG/PicoG-App/picoG/Instance.vi"}, {"Path"=path "<vilib>/ErrorRing/Error Ring.xnode", "Name"="Error Ring.xnode", "Referrer"=path "C:/dev/Vireo/PicoG/PicoG-App/picoG/Instance.vi"}, {"Path"=path "C:/dev/Vireo/PicoG/PicoG-App/picoG/Add App.vi", "Name"="PicoG-App.lvlib:picoG.lvclass:Add App.vi", "Referrer"=path "C:/dev/Vireo/PicoG/PicoG-App/picoG/Add App.vi"}, {"Path"=path "../picoG.lvclass", "Name"="PicoG-App.lvlib:picoG.lvclass", "Referrer"=path "C:/dev/Vireo/PicoG/PicoG-App/picoG/Add App.vi"}, {"Path"=path "../picoG.lvclass/picoG.ctl", "Name"="PicoG-App.lvlib:picoG.lvclass:picoG.ctl", "Referrer"=path "C:/dev/Vireo/PicoG/PicoG-App/picoG/Add App.vi"}, {"Path"=path "C:/dev/Vireo/PicoG/PicoG-App/AppListPanel/Sort Panels.vi", "Name"="PicoG-App.lvlib:AppListPanel.lvclass:Sort Panels.vi", "Referrer"=path "C:/dev/Vireo/PicoG/PicoG-App/AppListPanel/Sort Panels.vi"}, {"Path"=path "../AppListPanel.lvclass", "Name"="PicoG-App.lvlib:AppListPanel.lvclass", "Referrer"=path "C:/dev/Vireo/PicoG/PicoG-App/AppListPanel/Sort Panels.vi"}, {"Path"=path "../Sort Order.ctl", "Name"="PicoG-App.lvlib:AppListPanel.lvclass:Sort Order.ctl", "Referrer"=path "C:/dev/Vireo/PicoG/PicoG-App/AppListPanel/Sort Panels.vi"}, {"Path"=path "../AppListPanel.lvclass/AppListPanel.ctl", "Name"="PicoG-App.lvlib:AppListPanel.lvclass:AppListPanel.ctl", "Referrer"=path "C:/dev/Vireo/PicoG/PicoG-App/AppListPanel/Sort Panels.vi"}, {"Path"=path "../Sort By Updated.vi", "Name"="PicoG-App.lvlib:AppListPanel.lvclass:Sort By Updated.vi", "Referrer"=path "C:/dev/Vireo/PicoG/PicoG-App/AppListPanel/Sort Panels.vi"}, {"Path"=path "../Sort By Name.vi", "Name"="PicoG-App.lvlib:AppListPanel.lvclass:Sort By Name.vi", "Referrer"=path "C:/dev/Vireo/PicoG/PicoG-App/AppListPanel/Sort Panels.vi"}, {"Path"=path "<vilib>/IlluminatedG/IG OOPanel/OOPanel/ArrayManager/Sort Panels.vi", "Name"="OOPanel.lvlib:ArrayManager.lvclass:Sort Panels.vi", "Referrer"=path "C:/dev/Vireo/PicoG/PicoG-App/AppListPanel/Sort Panels.vi"}, {"Path"=path "<vilib>/IlluminatedG/IG OOPanel/OOPanel/Panel/Panel.lvclass", "Name"="OOPanel.lvlib:Panel.lvclass", "Referrer"=path "C:/dev/Vireo/PicoG/PicoG-App/AppListPanel/Sort Panels.vi"}, {"Path"=path "C:/dev/Vireo/PicoG/PicoG-App/picoG/Select Platform UI.vi", "Name"="PicoG-App.lvlib:picoG.lvclass:Select Platform UI.vi", "Referrer"=path "C:/dev/Vireo/PicoG/PicoG-App/picoG/Select Platform UI.vi"}, {"Path"=path "../picoG.lvclass", "Name"="PicoG-App.lvlib:picoG.lvclass", "Referrer"=path "C:/dev/Vireo/PicoG/PicoG-App/picoG/Select Platform UI.vi"}, {"Path"=path "../../../Builds/picoG/ppl/PicoG-Core.lvlibp/PicoG-Processor/PicoG-Core/PlatformManager/PlatformManager.lvclass", "Name"="PicoG-Core.lvlibp:PlatformManager.lvclass", "Referrer"=path "C:/dev/Vireo/PicoG/PicoG-App/picoG/Select Platform UI.vi"}, {"Path"=path "../../../Builds/picoG/ppl/PicoG-Core.lvlibp/PicoG-Processor/PicoG-Core/PlatformManager/Platform Names.vi", "Name"="PicoG-Core.lvlibp:PlatformManager.lvclass:Platform Names.vi", "Referrer"=path "C:/dev/Vireo/PicoG/PicoG-App/picoG/Select Platform UI.vi"}, {"Path"=path "C:/dev/Vireo/PicoG/PicoG-App/Device/Init.vi", "Name"="PicoG-App.lvlib:Device.lvclass:Init.vi", "Referrer"=path "C:/dev/Vireo/PicoG/PicoG-App/Device/Init.vi"}, {"Path"=path "../Device.lvclass", "Name"="PicoG-App.lvlib:Device.lvclass", "Referrer"=path "C:/dev/Vireo/PicoG/PicoG-App/Device/Init.vi"}, {"Path"=path "../../../Builds/picoG/ppl/PicoG-Core.lvlibp/PicoG-Processor/PicoG-Core/Platform/Platform.lvclass", "Name"="PicoG-Core.lvlibp:Platform.lvclass", "Referrer"=path "C:/dev/Vireo/PicoG/PicoG-App/Device/Init.vi"}, {"Path"=path "../../../Builds/picoG/ppl/PicoG-Core.lvlibp/PicoG-Processor/PicoG-Core/Resource/Resource.lvclass", "Name"="PicoG-Core.lvlibp:Resource.lvclass", "Referrer"=path "C:/dev/Vireo/PicoG/PicoG-App/Device/Init.vi"}, {"Path"=path "../Resource Ref.ctl", "Name"="PicoG-App.lvlib:Device.lvclass:Resource Ref.ctl", "Referrer"=path "C:/dev/Vireo/PicoG/PicoG-App/Device/Init.vi"}, {"Path"=path "../Ref Data.ctl", "Name"="PicoG-App.lvlib:Device.lvclass:Ref Data.ctl", "Referrer"=path "C:/dev/Vireo/PicoG/PicoG-App/Device/Init.vi"}, {"Path"=path "../Device Key.ctl", "Name"="PicoG-App.lvlib:Device.lvclass:Device Key.ctl", "Referrer"=path "C:/dev/Vireo/PicoG/PicoG-App/Device/Init.vi"}, {"Path"=path "../Device.lvclass/Device.ctl", "Name"="PicoG-App.lvlib:Device.lvclass:Device.ctl", "Referrer"=path "C:/dev/Vireo/PicoG/PicoG-App/Device/Init.vi"}, {"Path"=path "C:/dev/Vireo/PicoG/PicoG-App/Device/Refresh Device Info.vi", "Name"="PicoG-App.lvlib:Device.lvclass:Refresh Device Info.vi", "Referrer"=path "C:/dev/Vireo/PicoG/PicoG-App/Device/Refresh Device Info.vi"}, {"Path"=path "../Device.lvclass", "Name"="PicoG-App.lvlib:Device.lvclass", "Referrer"=path "C:/dev/Vireo/PicoG/PicoG-App/Device/Refresh Device Info.vi"}, {"Path"=path "C:/dev/Vireo/PicoG/PicoG-App/picoG/Confirm Device UI.vi", "Name"="PicoG-App.lvlib:picoG.lvclass:Confirm Device UI.vi", "Referrer"=path "C:/dev/Vireo/PicoG/PicoG-App/picoG/Confirm Device UI.vi"}, {"Path"=path "../picoG.lvclass", "Name"="PicoG-App.lvlib:picoG.lvclass", "Referrer"=path "C:/dev/Vireo/PicoG/PicoG-App/picoG/Confirm Device UI.vi"}, {"Path"=path "../../Device/Device.lvclass", "Name"="PicoG-App.lvlib:Device.lvclass", "Referrer"=path "C:/dev/Vireo/PicoG/PicoG-App/picoG/Confirm Device UI.vi"}, {"Path"=path "../../Device/Get Platform Name.vi", "Name"="PicoG-App.lvlib:Device.lvclass:Get Platform Name.vi", "Referrer"=path "C:/dev/Vireo/PicoG/PicoG-App/picoG/Confirm Device UI.vi"}, {"Path"=path "../../Device/Get Board.vi", "Name"="PicoG-App.lvlib:Device.lvclass:Get Board.vi", "Referrer"=path "C:/dev/Vireo/PicoG/PicoG-App/picoG/Confirm Device UI.vi"}, {"Path"=path "../../Device/Get ID.vi", "Name"="PicoG-App.lvlib:Device.lvclass:Get ID.vi", "Referrer"=path "C:/dev/Vireo/PicoG/PicoG-App/picoG/Confirm Device UI.vi"}, {"Path"=path "../../Device/Get Alias.vi", "Name"="PicoG-App.lvlib:Device.lvclass:Get Alias.vi", "Referrer"=path "C:/dev/Vireo/PicoG/PicoG-App/picoG/Confirm Device UI.vi"}, {"Path"=path "../../Device/Get Version String.vi", "Name"="PicoG-App.lvlib:Device.lvclass:Get Version String.vi", "Referrer"=path "C:/dev/Vireo/PicoG/PicoG-App/picoG/Confirm Device UI.vi"}, {"Path"=path "C:/dev/Vireo/PicoG/PicoG-App/DeviceListPanel/DeviceListPanel.lvclass/DeviceListPanel.ctl", "Name"="PicoG-App.lvlib:DeviceListPanel.lvclass:DeviceListPanel.ctl", "Referrer"=path "C:/dev/Vireo/PicoG/PicoG-App/DeviceListPanel/DeviceListPanel.lvclass/DeviceListPanel.ctl"}, {"Path"=path "..", "Name"="PicoG-App.lvlib:DeviceListPanel.lvclass", "Referrer"=path "C:/dev/Vireo/PicoG/PicoG-App/DeviceListPanel/DeviceListPanel.lvclass/DeviceListPanel.ctl"}, {"Path"=path "../../Ref Data.ctl", "Name"="PicoG-App.lvlib:DeviceListPanel.lvclass:Ref Data.ctl", "Referrer"=path "C:/dev/Vireo/PicoG/PicoG-App/DeviceListPanel/DeviceListPanel.lvclass/DeviceListPanel.ctl"}, {"Path"=path "../../../Device/Device Key.ctl", "Name"="PicoG-App.lvlib:Device.lvclass:Device Key.ctl", "Referrer"=path "C:/dev/Vireo/PicoG/PicoG-App/DeviceListPanel/DeviceListPanel.lvclass/DeviceListPanel.ctl"}, {"Path"=path "../../Device and Panel.ctl", "Name"="PicoG-App.lvlib:DeviceListPanel.lvclass:Device and Panel.ctl", "Referrer"=path "C:/dev/Vireo/PicoG/PicoG-App/DeviceListPanel/DeviceListPanel.lvclass/DeviceListPanel.ctl"}, {"Path"=path "../../../Device/Device.lvclass", "Name"="PicoG-App.lvlib:Device.lvclass", "Referrer"=path "C:/dev/Vireo/PicoG/PicoG-App/DeviceListPanel/DeviceListPanel.lvclass/DeviceListPanel.ctl"}, {"Path"=path "../../../DeviceArrayPanel/DeviceArrayPanel.lvclass", "Name"="PicoG-App.lvlib:DeviceArrayPanel.lvclass", "Referrer"=path "C:/dev/Vireo/PicoG/PicoG-App/DeviceListPanel/DeviceListPanel.lvclass/DeviceListPanel.ctl"}, {"Path"=path "../../Outbound Events.ctl", "Name"="PicoG-App.lvlib:DeviceListPanel.lvclass:Outbound Events.ctl", "Referrer"=path "C:/dev/Vireo/PicoG/PicoG-App/DeviceListPanel/DeviceListPanel.lvclass/DeviceListPanel.ctl"}, {"Path"=path "../../Inbound Events.ctl", "Name"="PicoG-App.lvlib:DeviceListPanel.lvclass:Inbound Events.ctl", "Referrer"=path "C:/dev/Vireo/PicoG/PicoG-App/DeviceListPanel/DeviceListPanel.lvclass/DeviceListPanel.ctl"}, {"Path"=path "<vilib>/IlluminatedG/IG OOPanel/OOPanel/ArrayManager/ArrayManager.lvclass", "Name"="OOPanel.lvlib:ArrayManager.lvclass", "Referrer"=path "C:/dev/Vireo/PicoG/PicoG-App/DeviceListPanel/DeviceListPanel.lvclass/DeviceListPanel.ctl"}, {"Path"=path "C:/dev/Vireo/PicoG/PicoG-App/DeviceArrayPanel/DeviceArrayPanel.lvclass", "Name"="PicoG-App.lvlib:DeviceArrayPanel.lvclass", "Referrer"=path "C:/dev/Vireo/PicoG/PicoG-App/DeviceArrayPanel/DeviceArrayPanel.lvclass"}, {"Path"=path "C:/dev/Vireo/PicoG/PicoG-App/PicoG-App.lvlib", "Name"="PicoG-App.lvlib", "Referrer"=path "C:/dev/Vireo/PicoG/PicoG-App/DeviceArrayPanel/DeviceArrayPanel.lvclass"}, {"Path"=path "C:/dev/Vireo/PicoG/PicoG-App/DeviceArrayPanel/DeviceArrayPanel.lvclass/DeviceArrayPanel.ctl", "Name"="PicoG-App.lvlib:DeviceArrayPanel.lvclass:DeviceArrayPanel.ctl", "Referrer"=path "C:/dev/Vireo/PicoG/PicoG-App/DeviceArrayPanel/DeviceArrayPanel.lvclass"}, {"Path"=path "C:/dev/Vireo/PicoG/PicoG-App/DeviceArrayPanel/Inbound Events.ctl", "Name"="PicoG-App.lvlib:DeviceArrayPanel.lvclass:Inbound Events.ctl", "Referrer"=path "C:/dev/Vireo/PicoG/PicoG-App/DeviceArrayPanel/DeviceArrayPanel.lvclass"}, {"Path"=path "C:/dev/Vireo/PicoG/PicoG-App/DeviceArrayPanel/Ref Data.ctl", "Name"="PicoG-App.lvlib:DeviceArrayPanel.lvclass:Ref Data.ctl", "Referrer"=path "C:/dev/Vireo/PicoG/PicoG-App/DeviceArrayPanel/DeviceArrayPanel.lvclass"}, {"Path"=path "C:/dev/Vireo/PicoG/PicoG-App/DeviceArrayPanel/Init Events.vi", "Name"="PicoG-App.lvlib:DeviceArrayPanel.lvclass:Init Events.vi", "Referrer"=path "C:/dev/Vireo/PicoG/PicoG-App/DeviceArrayPanel/DeviceArrayPanel.lvclass"}, {"Path"=path "C:/dev/Vireo/PicoG/PicoG-App/DeviceArrayPanel/Get Desired Size.vi", "Name"="PicoG-App.lvlib:DeviceArrayPanel.lvclass:Get Desired Size.vi", "Referrer"=path "C:/dev/Vireo/PicoG/PicoG-App/DeviceArrayPanel/DeviceArrayPanel.lvclass"}, {"Path"=path "C:/dev/Vireo/PicoG/PicoG-App/DeviceArrayPanel/Set Device.vi", "Name"="PicoG-App.lvlib:DeviceArrayPanel.lvclass:Set Device.vi", "Referrer"=path "C:/dev/Vireo/PicoG/PicoG-App/DeviceArrayPanel/DeviceArrayPanel.lvclass"}, {"Path"=path "C:/dev/Vireo/PicoG/PicoG-App/DeviceArrayPanel/Set Highlighted.vi", "Name"="PicoG-App.lvlib:DeviceArrayPanel.lvclass:Set Highlighted.vi", "Referrer"=path "C:/dev/Vireo/PicoG/PicoG-App/DeviceArrayPanel/DeviceArrayPanel.lvclass"}, {"Path"=path "C:/dev/Vireo/PicoG/PicoG-App/DeviceArrayPanel/Set Select Event.vi", "Name"="PicoG-App.lvlib:DeviceArrayPanel.lvclass:Set Select Event.vi", "Referrer"=path "C:/dev/Vireo/PicoG/PicoG-App/DeviceArrayPanel/DeviceArrayPanel.lvclass"}, {"Path"=path "C:/dev/Vireo/PicoG/PicoG-App/DeviceArrayPanel/Cleanup.vi", "Name"="PicoG-App.lvlib:DeviceArrayPanel.lvclass:Cleanup.vi", "Referrer"=path "C:/dev/Vireo/PicoG/PicoG-App/DeviceArrayPanel/DeviceArrayPanel.lvclass"}, {"Path"=path "C:/dev/Vireo/PicoG/PicoG-App/DeviceArrayPanel/Ctor.vi", "Name"="PicoG-App.lvlib:DeviceArrayPanel.lvclass:Ctor.vi", "Referrer"=path "C:/dev/Vireo/PicoG/PicoG-App/DeviceArrayPanel/DeviceArrayPanel.lvclass"}, {"Path"=path "C:/dev/Vireo/PicoG/PicoG-App/DeviceArrayPanel/Panel.vi", "Name"="PicoG-App.lvlib:DeviceArrayPanel.lvclass:Panel.vi", "Referrer"=path "C:/dev/Vireo/PicoG/PicoG-App/DeviceArrayPanel/DeviceArrayPanel.lvclass"}, {"Path"=path "C:/Program Files (x86)/National Instruments/LabVIEW 2020/vi.lib/IlluminatedG/IG OOPanel/OOPanel/ArrayPanel/ArrayPanel.lvclass", "Name"="OOPanel.lvlib:ArrayPanel.lvclass", "Referrer"=path "C:/dev/Vireo/PicoG/PicoG-App/DeviceArrayPanel/DeviceArrayPanel.lvclass"}, {"Path"=path "C:/dev/Vireo/PicoG/PicoG-App/DeviceArrayPanel/Set Highlighted.vi", "Name"="PicoG-App.lvlib:DeviceArrayPanel.lvclass:Set Highlighted.vi", "Referrer"=path "C:/dev/Vireo/PicoG/PicoG-App/DeviceArrayPanel/Set Highlighted.vi"}, {"Path"=path "../DeviceArrayPanel.lvclass", "Name"="PicoG-App.lvlib:DeviceArrayPanel.lvclass", "Referrer"=path "C:/dev/Vireo/PicoG/PicoG-App/DeviceArrayPanel/Set Highlighted.vi"}, {"Path"=path "../DeviceArrayPanel.lvclass/DeviceArrayPanel.ctl", "Name"="PicoG-App.lvlib:DeviceArrayPanel.lvclass:DeviceArrayPanel.ctl", "Referrer"=path "C:/dev/Vireo/PicoG/PicoG-App/DeviceArrayPanel/Set Highlighted.vi"}, {"Path"=path "C:/dev/Vireo/PicoG/PicoG-App/App Watcher/Check Apps.vi", "Name"="PicoG-App.lvlib:App Watcher.lvclass:Check Apps.vi", "Referrer"=path "C:/dev/Vireo/PicoG/PicoG-App/App Watcher/Check Apps.vi"}, {"Path"=path "../App Watcher.lvclass", "Name"="PicoG-App.lvlib:App Watcher.lvclass", "Referrer"=path "C:/dev/Vireo/PicoG/PicoG-App/App Watcher/Check Apps.vi"}, {"Path"=path "../App Watcher.lvclass/App Watcher.ctl", "Name"="PicoG-App.lvlib:App Watcher.lvclass:App Watcher.ctl", "Referrer"=path "C:/dev/Vireo/PicoG/PicoG-App/App Watcher/Check Apps.vi"}, {"Path"=path "../App Update Data.ctl", "Name"="PicoG-App.lvlib:App Watcher.lvclass:App Update Data.ctl", "Referrer"=path "C:/dev/Vireo/PicoG/PicoG-App/App Watcher/Check Apps.vi"}, {"Path"=path "../../ViaApp/ViaApp.lvclass", "Name"="PicoG-App.lvlib:ViaApp.lvclass", "Referrer"=path "C:/dev/Vireo/PicoG/PicoG-App/App Watcher/Check Apps.vi"}, {"Path"=path "../../ViaApp/Get Updated.vi", "Name"="PicoG-App.lvlib:ViaApp.lvclass:Get Updated.vi", "Referrer"=path "C:/dev/Vireo/PicoG/PicoG-App/App Watcher/Check Apps.vi"}, {"Path"=path "../../ViaApp/Set Updated.vi", "Name"="PicoG-App.lvlib:ViaApp.lvclass:Set Updated.vi", "Referrer"=path "C:/dev/Vireo/PicoG/PicoG-App/App Watcher/Check Apps.vi"}, {"Path"=path "../../ViaApp/Get Path.vi", "Name"="PicoG-App.lvlib:ViaApp.lvclass:Get Path.vi", "Referrer"=path "C:/dev/Vireo/PicoG/PicoG-App/App Watcher/Check Apps.vi"}, {"Path"=path "C:/dev/Vireo/PicoG/Builds/picoG/ppl/PicoG-Core.lvlibp/PicoG-Processor/PicoG-Core/PlatformManager/Platform Plugin Folder.vi", "Name"="PicoG-Core.lvlibp:PlatformManager.lvclass:Platform Plugin Folder.vi", "Referrer"=path "C:/dev/Vireo/PicoG/Builds/picoG/ppl/PicoG-Core.lvlibp/PicoG-Processor/PicoG-Core/PlatformManager/Platform Plugin Folder.vi"}, {"Path"=path "../PlatformManager.lvclass", "Name"="PicoG-Core.lvlibp:PlatformManager.lvclass", "Referrer"=path "C:/dev/Vireo/PicoG/Builds/picoG/ppl/PicoG-Core.lvlibp/PicoG-Processor/PicoG-Core/PlatformManager/Platform Plugin Folder.vi"}, {"Path"=path "C:/dev/Vireo/PicoG/Builds/picoG/ppl/PicoG-Core.lvlibp/1abvi3w/vi.lib/Utility/LVLibp/Get Exported File List.vi", "Name"="PicoG-Core.lvlibp:NI_PackedLibraryUtility.lvlib:Get Exported File List.vi", "Referrer"=path "C:/dev/Vireo/PicoG/Builds/picoG/ppl/PicoG-Core.lvlibp/1abvi3w/vi.lib/Utility/LVLibp/Get Exported File List.vi"}, {"Path"=path "../NI_PackedLibraryUtility.lvlib", "Name"="PicoG-Core.lvlibp:NI_PackedLibraryUtility.lvlib", "Referrer"=path "C:/dev/Vireo/PicoG/Builds/picoG/ppl/PicoG-Core.lvlibp/1abvi3w/vi.lib/Utility/LVLibp/Get Exported File List.vi"}, {"Path"=path "C:/dev/Vireo/PicoG/Builds/picoG/ppl/PicoG-Core.lvlibp/1abvi3w/vi.lib/Utility/LVClass/Get LV Class Default Value.vi", "Name"="PicoG-Core.lvlibp:Get LV Class Default Value.vi", "Referrer"=path "C:/dev/Vireo/PicoG/Builds/picoG/ppl/PicoG-Core.lvlibp/1abvi3w/vi.lib/Utility/LVClass/Get LV Class Default Value.vi"}, {"Path"=path "../../../../..", "Name"="PicoG-Core.lvlibp", "Referrer"=path "C:/dev/Vireo/PicoG/Builds/picoG/ppl/PicoG-Core.lvlibp/1abvi3w/vi.lib/Utility/LVClass/Get LV Class Default Value.vi"}, {"Path"=path "../../error.llb/Error Cluster From Error Code.vi", "Name"="PicoG-Core.lvlibp:Error Cluster From Error Code.vi", "Referrer"=path "C:/dev/Vireo/PicoG/Builds/picoG/ppl/PicoG-Core.lvlibp/1abvi3w/vi.lib/Utility/LVClass/Get LV Class Default Value.vi"}, {"Path"=path "LabVIEW", "Name"="LabVIEW", "Referrer"=path "C:/dev/Vireo/PicoG/Builds/picoG/ppl/PicoG-Core.lvlibp/1abvi3w/vi.lib/Utility/LVClass/Get LV Class Default Value.vi"}, {"Path"=path "C:/dev/Vireo/PicoG/PicoG-App/Paths.ctl", "Name"="PicoG-App.lvlib:Paths.ctl", "Referrer"=path "C:/dev/Vireo/PicoG/PicoG-App/Paths.ctl"}, {"Path"=path "../PicoG-App.lvlib", "Name"="PicoG-App.lvlib", "Referrer"=path "C:/dev/Vireo/PicoG/PicoG-App/Paths.ctl"}, {"Path"=path "C:/dev/Vireo/PicoG/PicoG-App/picoG/Read Single Device.vi", "Name"="PicoG-App.lvlib:picoG.lvclass:Read Single Device.vi", "Referrer"=path "C:/dev/Vireo/PicoG/PicoG-App/picoG/Read Single Device.vi"}, {"Path"=path "../picoG.lvclass", "Name"="PicoG-App.lvlib:picoG.lvclass", "Referrer"=path "C:/dev/Vireo/PicoG/PicoG-App/picoG/Read Single Device.vi"}, {"Path"=path "<vilib>/Utility/config.llb/Config Data RefNum.ctl", "Name"="NI_LVConfig.lvlib:Config Data RefNum.ctl", "Referrer"=path "C:/dev/Vireo/PicoG/PicoG-App/picoG/Read Single Device.vi"}, {"Path"=path "../../Device/Device.lvclass", "Name"="PicoG-App.lvlib:Device.lvclass", "Referrer"=path "C:/dev/Vireo/PicoG/PicoG-App/picoG/Read Single Device.vi"}, {"Path"=path "../../Device/Device Key.ctl", "Name"="PicoG-App.lvlib:Device.lvclass:Device Key.ctl", "Referrer"=path "C:/dev/Vireo/PicoG/PicoG-App/picoG/Read Single Device.vi"}, {"Path"=path "../../../Builds/picoG/ppl/PicoG-Core.lvlibp/PicoG-Processor/PicoG-Core/Resource/Resource.lvclass", "Name"="PicoG-Core.lvlibp:Resource.lvclass", "Referrer"=path "C:/dev/Vireo/PicoG/PicoG-App/picoG/Read Single Device.vi"}, {"Path"=path "../../../Builds/picoG/ppl/PicoG-Core.lvlibp/PicoG-Processor/PicoG-Core/Resource/Config Item.ctl", "Name"="PicoG-Core.lvlibp:Resource.lvclass:Config Item.ctl", "Referrer"=path "C:/dev/Vireo/PicoG/PicoG-App/picoG/Read Single Device.vi"}, {"Path"=path "<vilib>/Utility/config.llb/Read Key.vi", "Name"="NI_LVConfig.lvlib:Read Key.vi", "Referrer"=path "C:/dev/Vireo/PicoG/PicoG-App/picoG/Read Single Device.vi"}, {"Path"=path "<vilib>/Utility/config.llb/Read Key (String).vi", "Name"="NI_LVConfig.lvlib:Read Key (String).vi", "Referrer"=path "C:/dev/Vireo/PicoG/PicoG-App/picoG/Read Single Device.vi"}, {"Path"=path "<vilib>/Utility/LVClass/Get LV Class Default Value By Name.vi", "Name"="Get LV Class Default Value By Name.vi", "Referrer"=path "C:/dev/Vireo/PicoG/PicoG-App/picoG/Read Single Device.vi"}, {"Path"=path "../../../Builds/picoG/ppl/PicoG-Core.lvlibp/PicoG-Processor/PicoG-Core/Resource/Set Config.vi", "Name"="PicoG-Core.lvlibp:Resource.lvclass:Set Config.vi", "Referrer"=path "C:/dev/Vireo/PicoG/PicoG-App/picoG/Read Single Device.vi"}, {"Path"=path "../../Device/Init from Config.vi", "Name"="PicoG-App.lvlib:Device.lvclass:Init from Config.vi", "Referrer"=path "C:/dev/Vireo/PicoG/PicoG-App/picoG/Read Single Device.vi"}, {"Path"=path "C:/dev/Vireo/PicoG/PicoG-App/ViaApp/ViaApp.lvclass/ViaApp.ctl", "Name"="PicoG-App.lvlib:ViaApp.lvclass:ViaApp.ctl", "Referrer"=path "C:/dev/Vireo/PicoG/PicoG-App/ViaApp/ViaApp.lvclass/ViaApp.ctl"}, {"Path"=path "..", "Name"="PicoG-App.lvlib:ViaApp.lvclass", "Referrer"=path "C:/dev/Vireo/PicoG/PicoG-App/ViaApp/ViaApp.lvclass/ViaApp.ctl"}, {"Path"=path "C:/dev/Vireo/PicoG/PicoG-App/AppListPanel/Ref Data.ctl", "Name"="PicoG-App.lvlib:AppListPanel.lvclass:Ref Data.ctl", "Referrer"=path "C:/dev/Vireo/PicoG/PicoG-App/AppListPanel/Ref Data.ctl"}, {"Path"=path "../AppListPanel.lvclass", "Name"="PicoG-App.lvlib:AppListPanel.lvclass", "Referrer"=path "C:/dev/Vireo/PicoG/PicoG-App/AppListPanel/Ref Data.ctl"}, {"Path"=path "../App Panel.ctl", "Name"="PicoG-App.lvlib:AppListPanel.lvclass:App Panel.ctl", "Referrer"=path "C:/dev/Vireo/PicoG/PicoG-App/AppListPanel/Ref Data.ctl"}, {"Path"=path "../../ViaApp/ViaApp.lvclass", "Name"="PicoG-App.lvlib:ViaApp.lvclass", "Referrer"=path "C:/dev/Vireo/PicoG/PicoG-App/AppListPanel/Ref Data.ctl"}, {"Path"=path "../../GWebAppArrayPanel/GWebAppArrayPanel.lvclass", "Name"="PicoG-App.lvlib:GWebAppArrayPanel.lvclass", "Referrer"=path "C:/dev/Vireo/PicoG/PicoG-App/AppListPanel/Ref Data.ctl"}, {"Path"=path "C:/dev/Vireo/PicoG/PicoG-App/AppListPanel/App Panel.ctl", "Name"="PicoG-App.lvlib:AppListPanel.lvclass:App Panel.ctl", "Referrer"=path "C:/dev/Vireo/PicoG/PicoG-App/AppListPanel/App Panel.ctl"}, {"Path"=path "../AppListPanel.lvclass", "Name"="PicoG-App.lvlib:AppListPanel.lvclass", "Referrer"=path "C:/dev/Vireo/PicoG/PicoG-App/AppListPanel/App Panel.ctl"}, {"Path"=path "../../ViaApp/ViaApp.lvclass", "Name"="PicoG-App.lvlib:ViaApp.lvclass", "Referrer"=path "C:/dev/Vireo/PicoG/PicoG-App/AppListPanel/App Panel.ctl"}, {"Path"=path "../../GWebAppArrayPanel/GWebAppArrayPanel.lvclass", "Name"="PicoG-App.lvlib:GWebAppArrayPanel.lvclass", "Referrer"=path "C:/dev/Vireo/PicoG/PicoG-App/AppListPanel/App Panel.ctl"}, {"Path"=path "C:/dev/Vireo/PicoG/PicoG-App/AppListPanel/Inbound Events.ctl", "Name"="PicoG-App.lvlib:AppListPanel.lvclass:Inbound Events.ctl", "Referrer"=path "C:/dev/Vireo/PicoG/PicoG-App/AppListPanel/Inbound Events.ctl"}, {"Path"=path "../AppListPanel.lvclass", "Name"="PicoG-App.lvlib:AppListPanel.lvclass", "Referrer"=path "C:/dev/Vireo/PicoG/PicoG-App/AppListPanel/Inbound Events.ctl"}, {"Path"=path "../../ViaApp/ViaApp.lvclass", "Name"="PicoG-App.lvlib:ViaApp.lvclass", "Referrer"=path "C:/dev/Vireo/PicoG/PicoG-App/AppListPanel/Inbound Events.ctl"}, {"Path"=path "C:/dev/Vireo/PicoG/PicoG-App/AppListPanel/Outbound Events.ctl", "Name"="PicoG-App.lvlib:AppListPanel.lvclass:Outbound Events.ctl", "Referrer"=path "C:/dev/Vireo/PicoG/PicoG-App/AppListPanel/Outbound Events.ctl"}, {"Path"=path "../AppListPanel.lvclass", "Name"="PicoG-App.lvlib:AppListPanel.lvclass", "Referrer"=path "C:/dev/Vireo/PicoG/PicoG-App/AppListPanel/Outbound Events.ctl"}, {"Path"=path "../../ViaApp/ViaApp.lvclass", "Name"="PicoG-App.lvlib:ViaApp.lvclass", "Referrer"=path "C:/dev/Vireo/PicoG/PicoG-App/AppListPanel/Outbound Events.ctl"}, {"Path"=path "C:/dev/Vireo/PicoG/PicoG-App/picoG/Write Single Device.vi", "Name"="PicoG-App.lvlib:picoG.lvclass:Write Single Device.vi", "Referrer"=path "C:/dev/Vireo/PicoG/PicoG-App/picoG/Write Single Device.vi"}, {"Path"=path "../picoG.lvclass", "Name"="PicoG-App.lvlib:picoG.lvclass", "Referrer"=path "C:/dev/Vireo/PicoG/PicoG-App/picoG/Write Single Device.vi"}, {"Path"=path "<vilib>/Utility/config.llb/Config Data RefNum.ctl", "Name"="NI_LVConfig.lvlib:Config Data RefNum.ctl", "Referrer"=path "C:/dev/Vireo/PicoG/PicoG-App/picoG/Write Single Device.vi"}, {"Path"=path "../../Device/Device.lvclass", "Name"="PicoG-App.lvlib:Device.lvclass", "Referrer"=path "C:/dev/Vireo/PicoG/PicoG-App/picoG/Write Single Device.vi"}, {"Path"=path "../../Device/Get Platform Name.vi", "Name"="PicoG-App.lvlib:Device.lvclass:Get Platform Name.vi", "Referrer"=path "C:/dev/Vireo/PicoG/PicoG-App/picoG/Write Single Device.vi"}, {"Path"=path "../../Device/Get Board.vi", "Name"="PicoG-App.lvlib:Device.lvclass:Get Board.vi", "Referrer"=path "C:/dev/Vireo/PicoG/PicoG-App/picoG/Write Single Device.vi"}, {"Path"=path "../../Device/Get ID.vi", "Name"="PicoG-App.lvlib:Device.lvclass:Get ID.vi", "Referrer"=path "C:/dev/Vireo/PicoG/PicoG-App/picoG/Write Single Device.vi"}, {"Path"=path "../../Device/Get Alias.vi", "Name"="PicoG-App.lvlib:Device.lvclass:Get Alias.vi", "Referrer"=path "C:/dev/Vireo/PicoG/PicoG-App/picoG/Write Single Device.vi"}, {"Path"=path "../../Device/Get Version String.vi", "Name"="PicoG-App.lvlib:Device.lvclass:Get Version String.vi", "Referrer"=path "C:/dev/Vireo/PicoG/PicoG-App/picoG/Write Single Device.vi"}, {"Path"=path "../../Device/Get Resource.vi", "Name"="PicoG-App.lvlib:Device.lvclass:Get Resource.vi", "Referrer"=path "C:/dev/Vireo/PicoG/PicoG-App/picoG/Write Single Device.vi"}, {"Path"=path "<vilib>/Utility/LVClass/Get LV Class Name.vi", "Name"="Get LV Class Name.vi", "Referrer"=path "C:/dev/Vireo/PicoG/PicoG-App/picoG/Write Single Device.vi"}, {"Path"=path "<vilib>/Utility/config.llb/Write Key.vi", "Name"="NI_LVConfig.lvlib:Write Key.vi", "Referrer"=path "C:/dev/Vireo/PicoG/PicoG-App/picoG/Write Single Device.vi"}, {"Path"=path "<vilib>/Utility/config.llb/Write Key (String).vi", "Name"="NI_LVConfig.lvlib:Write Key (String).vi", "Referrer"=path "C:/dev/Vireo/PicoG/PicoG-App/picoG/Write Single Device.vi"}, {"Path"=path "../../../Builds/picoG/ppl/PicoG-Core.lvlibp/PicoG-Processor/PicoG-Core/Resource/Resource.lvclass", "Name"="PicoG-Core.lvlibp:Resource.lvclass", "Referrer"=path "C:/dev/Vireo/PicoG/PicoG-App/picoG/Write Single Device.vi"}, {"Path"=path "C:/dev/Vireo/PicoG/PicoG-App/GWebAppArrayPanel/GWebAppArrayPanel.lvclass/GWebAppArrayPanel.ctl", "Name"="PicoG-App.lvlib:GWebAppArrayPanel.lvclass:GWebAppArrayPanel.ctl", "Referrer"=path "C:/dev/Vireo/PicoG/PicoG-App/GWebAppArrayPanel/GWebAppArrayPanel.lvclass/GWebAppArrayPanel.ctl"}, {"Path"=path "..", "Name"="PicoG-App.lvlib:GWebAppArrayPanel.lvclass", "Referrer"=path "C:/dev/Vireo/PicoG/PicoG-App/GWebAppArrayPanel/GWebAppArrayPanel.lvclass/GWebAppArrayPanel.ctl"}, {"Path"=path "../../Ref Data.ctl", "Name"="PicoG-App.lvlib:GWebAppArrayPanel.lvclass:Ref Data.ctl", "Referrer"=path "C:/dev/Vireo/PicoG/PicoG-App/GWebAppArrayPanel/GWebAppArrayPanel.lvclass/GWebAppArrayPanel.ctl"}, {"Path"=path "../../../ViaApp/ViaApp.lvclass", "Name"="PicoG-App.lvlib:ViaApp.lvclass", "Referrer"=path "C:/dev/Vireo/PicoG/PicoG-App/GWebAppArrayPanel/GWebAppArrayPanel.lvclass/GWebAppArrayPanel.ctl"}, {"Path"=path "../../Outbound Events.ctl", "Name"="PicoG-App.lvlib:GWebAppArrayPanel.lvclass:Outbound Events.ctl", "Referrer"=path "C:/dev/Vireo/PicoG/PicoG-App/GWebAppArrayPanel/GWebAppArrayPanel.lvclass/GWebAppArrayPanel.ctl"}, {"Path"=path "../../Panel Events.ctl", "Name"="PicoG-App.lvlib:GWebAppArrayPanel.lvclass:Panel Events.ctl", "Referrer"=path "C:/dev/Vireo/PicoG/PicoG-App/GWebAppArrayPanel/GWebAppArrayPanel.lvclass/GWebAppArrayPanel.ctl"}, {"Path"=path "C:/dev/Vireo/PicoG/PicoG-App/PlatformArrayPanel/PlatformArrayPanel.lvclass/PlatformArrayPanel.ctl", "Name"="PicoG-App.lvlib:PlatformArrayPanel.lvclass:PlatformArrayPanel.ctl", "Referrer"=path "C:/dev/Vireo/PicoG/PicoG-App/PlatformArrayPanel/PlatformArrayPanel.lvclass/PlatformArrayPanel.ctl"}, {"Path"=path "..", "Name"="PicoG-App.lvlib:PlatformArrayPanel.lvclass", "Referrer"=path "C:/dev/Vireo/PicoG/PicoG-App/PlatformArrayPanel/PlatformArrayPanel.lvclass/PlatformArrayPanel.ctl"}, {"Path"=path "../../../../Builds/picoG/ppl/PicoG-Core.lvlibp/PicoG-Processor/PicoG-Core/Platform/Platform.lvclass", "Name"="PicoG-Core.lvlibp:Platform.lvclass", "Referrer"=path "C:/dev/Vireo/PicoG/PicoG-App/PlatformArrayPanel/PlatformArrayPanel.lvclass/PlatformArrayPanel.ctl"}, {"Path"=path "../../Panel Events.ctl", "Name"="PicoG-App.lvlib:PlatformArrayPanel.lvclass:Panel Events.ctl", "Referrer"=path "C:/dev/Vireo/PicoG/PicoG-App/PlatformArrayPanel/PlatformArrayPanel.lvclass/PlatformArrayPanel.ctl"}, {"Path"=path "../../Outbound Events.ctl", "Name"="PicoG-App.lvlib:PlatformArrayPanel.lvclass:Outbound Events.ctl", "Referrer"=path "C:/dev/Vireo/PicoG/PicoG-App/PlatformArrayPanel/PlatformArrayPanel.lvclass/PlatformArrayPanel.ctl"}, {"Path"=path "C:/dev/Vireo/PicoG/PicoG-App/AppDetailPanel/Ref Data.ctl", "Name"="PicoG-App.lvlib:AppDetailPanel.lvclass:Ref Data.ctl", "Referrer"=path "C:/dev/Vireo/PicoG/PicoG-App/AppDetailPanel/Ref Data.ctl"}, {"Path"=path "../AppDetailPanel.lvclass", "Name"="PicoG-App.lvlib:AppDetailPanel.lvclass", "Referrer"=path "C:/dev/Vireo/PicoG/PicoG-App/AppDetailPanel/Ref Data.ctl"}, {"Path"=path "../../ViaApp/ViaApp.lvclass", "Name"="PicoG-App.lvlib:ViaApp.lvclass", "Referrer"=path "C:/dev/Vireo/PicoG/PicoG-App/AppDetailPanel/Ref Data.ctl"}, {"Path"=path "C:/dev/Vireo/PicoG/PicoG-App/AppDetailPanel/Incoming Events.ctl", "Name"="PicoG-App.lvlib:AppDetailPanel.lvclass:Incoming Events.ctl", "Referrer"=path "C:/dev/Vireo/PicoG/PicoG-App/AppDetailPanel/Incoming Events.ctl"}, {"Path"=path "../AppDetailPanel.lvclass", "Name"="PicoG-App.lvlib:AppDetailPanel.lvclass", "Referrer"=path "C:/dev/Vireo/PicoG/PicoG-App/AppDetailPanel/Incoming Events.ctl"}, {"Path"=path "C:/dev/Vireo/PicoG/PicoG-App/GWebAppArrayPanel/Set Via App.vi", "Name"="PicoG-App.lvlib:GWebAppArrayPanel.lvclass:Set Via App.vi", "Referrer"=path "C:/dev/Vireo/PicoG/PicoG-App/GWebAppArrayPanel/Set Via App.vi"}, {"Path"=path "../GWebAppArrayPanel.lvclass", "Name"="PicoG-App.lvlib:GWebAppArrayPanel.lvclass", "Referrer"=path "C:/dev/Vireo/PicoG/PicoG-App/GWebAppArrayPanel/Set Via App.vi"}, {"Path"=path "../../ViaApp/ViaApp.lvclass", "Name"="PicoG-App.lvlib:ViaApp.lvclass", "Referrer"=path "C:/dev/Vireo/PicoG/PicoG-App/GWebAppArrayPanel/Set Via App.vi"}, {"Path"=path "../GWebAppArrayPanel.lvclass/GWebAppArrayPanel.ctl", "Name"="PicoG-App.lvlib:GWebAppArrayPanel.lvclass:GWebAppArrayPanel.ctl", "Referrer"=path "C:/dev/Vireo/PicoG/PicoG-App/GWebAppArrayPanel/Set Via App.vi"}, {"Path"=path "C:/dev/Vireo/PicoG/PicoG-App/GWebAppArrayPanel/Set Select Event.vi", "Name"="PicoG-App.lvlib:GWebAppArrayPanel.lvclass:Set Select Event.vi", "Referrer"=path "C:/dev/Vireo/PicoG/PicoG-App/GWebAppArrayPanel/Set Select Event.vi"}, {"Path"=path "../GWebAppArrayPanel.lvclass", "Name"="PicoG-App.lvlib:GWebAppArrayPanel.lvclass", "Referrer"=path "C:/dev/Vireo/PicoG/PicoG-App/GWebAppArrayPanel/Set Select Event.vi"}, {"Path"=path "../../ViaApp/ViaApp.lvclass", "Name"="PicoG-App.lvlib:ViaApp.lvclass", "Referrer"=path "C:/dev/Vireo/PicoG/PicoG-App/GWebAppArrayPanel/Set Select Event.vi"}, {"Path"=path "../GWebAppArrayPanel.lvclass/GWebAppArrayPanel.ctl", "Name"="PicoG-App.lvlib:GWebAppArrayPanel.lvclass:GWebAppArrayPanel.ctl", "Referrer"=path "C:/dev/Vireo/PicoG/PicoG-App/GWebAppArrayPanel/Set Select Event.vi"}, {"Path"=path "C:/dev/Vireo/PicoG/PicoG-App/AppListPanel/Sort By Updated.vi", "Name"="PicoG-App.lvlib:AppListPanel.lvclass:Sort By Updated.vi", "Referrer"=path "C:/dev/Vireo/PicoG/PicoG-App/AppListPanel/Sort By Updated.vi"}, {"Path"=path "../AppListPanel.lvclass", "Name"="PicoG-App.lvlib:AppListPanel.lvclass", "Referrer"=path "C:/dev/Vireo/PicoG/PicoG-App/AppListPanel/Sort By Updated.vi"}, {"Path"=path "<vilib>/IlluminatedG/IG OOPanel/OOPanel/Panel/Panel.lvclass", "Name"="OOPanel.lvlib:Panel.lvclass", "Referrer"=path "C:/dev/Vireo/PicoG/PicoG-App/AppListPanel/Sort By Updated.vi"}, {"Path"=path "../../GWebAppArrayPanel/GWebAppArrayPanel.lvclass", "Name"="PicoG-App.lvlib:GWebAppArrayPanel.lvclass", "Referrer"=path "C:/dev/Vireo/PicoG/PicoG-App/AppListPanel/Sort By Updated.vi"}, {"Path"=path "../../GWebAppArrayPanel/Get Via App.vi", "Name"="PicoG-App.lvlib:GWebAppArrayPanel.lvclass:Get Via App.vi", "Referrer"=path "C:/dev/Vireo/PicoG/PicoG-App/AppListPanel/Sort By Updated.vi"}, {"Path"=path "../../ViaApp/Get Updated.vi", "Name"="PicoG-App.lvlib:ViaApp.lvclass:Get Updated.vi", "Referrer"=path "C:/dev/Vireo/PicoG/PicoG-App/AppListPanel/Sort By Updated.vi"}, {"Path"=path "C:/dev/Vireo/PicoG/PicoG-App/AppListPanel/Sort By Name.vi", "Name"="PicoG-App.lvlib:AppListPanel.lvclass:Sort By Name.vi", "Referrer"=path "C:/dev/Vireo/PicoG/PicoG-App/AppListPanel/Sort By Name.vi"}, {"Path"=path "../AppListPanel.lvclass", "Name"="PicoG-App.lvlib:AppListPanel.lvclass", "Referrer"=path "C:/dev/Vireo/PicoG/PicoG-App/AppListPanel/Sort By Name.vi"}, {"Path"=path "<vilib>/IlluminatedG/IG OOPanel/OOPanel/Panel/Panel.lvclass", "Name"="OOPanel.lvlib:Panel.lvclass", "Referrer"=path "C:/dev/Vireo/PicoG/PicoG-App/AppListPanel/Sort By Name.vi"}, {"Path"=path "../../GWebAppArrayPanel/GWebAppArrayPanel.lvclass", "Name"="PicoG-App.lvlib:GWebAppArrayPanel.lvclass", "Referrer"=path "C:/dev/Vireo/PicoG/PicoG-App/AppListPanel/Sort By Name.vi"}, {"Path"=path "../../GWebAppArrayPanel/Get Via App.vi", "Name"="PicoG-App.lvlib:GWebAppArrayPanel.lvclass:Get Via App.vi", "Referrer"=path "C:/dev/Vireo/PicoG/PicoG-App/AppListPanel/Sort By Name.vi"}, {"Path"=path "../../ViaApp/Get Path.vi", "Name"="PicoG-App.lvlib:ViaApp.lvclass:Get Path.vi", "Referrer"=path "C:/dev/Vireo/PicoG/PicoG-App/AppListPanel/Sort By Name.vi"}, {"Path"=path "<vilib>/Utility/libraryn.llb/Get File Extension.vi", "Name"="Get File Extension.vi", "Referrer"=path "C:/dev/Vireo/PicoG/PicoG-App/AppListPanel/Sort By Name.vi"}, {"Path"=path "C:/dev/Vireo/PicoG/Builds/picoG/ppl/PicoG-Core.lvlibp/PicoG-Processor/PicoG-Core/PlatformManager/Platform Names.vi", "Name"="PicoG-Core.lvlibp:PlatformManager.lvclass:Platform Names.vi", "Referrer"=path "C:/dev/Vireo/PicoG/Builds/picoG/ppl/PicoG-Core.lvlibp/PicoG-Processor/PicoG-Core/PlatformManager/Platform Names.vi"}, {"Path"=path "../PlatformManager.lvclass", "Name"="PicoG-Core.lvlibp:PlatformManager.lvclass", "Referrer"=path "C:/dev/Vireo/PicoG/Builds/picoG/ppl/PicoG-Core.lvlibp/PicoG-Processor/PicoG-Core/PlatformManager/Platform Names.vi"}, {"Path"=path "../PlatformManager.lvclass/PlatformManager.ctl", "Name"="PicoG-Core.lvlibp:PlatformManager.lvclass:PlatformManager.ctl", "Referrer"=path "C:/dev/Vireo/PicoG/Builds/picoG/ppl/PicoG-Core.lvlibp/PicoG-Processor/PicoG-Core/PlatformManager/Platform Names.vi"}, {"Path"=path "../../Platform/Platform.lvclass", "Name"="PicoG-Core.lvlibp:Platform.lvclass", "Referrer"=path "C:/dev/Vireo/PicoG/Builds/picoG/ppl/PicoG-Core.lvlibp/PicoG-Processor/PicoG-Core/PlatformManager/Platform Names.vi"}, {"Path"=path "C:/dev/Vireo/PicoG/Builds/picoG/ppl/PicoG-Core.lvlibp/PicoG-Processor/PicoG-Core/Resource/Resource.lvclass", "Name"="PicoG-Core.lvlibp:Resource.lvclass", "Referrer"=path "C:/dev/Vireo/PicoG/Builds/picoG/ppl/PicoG-Core.lvlibp/PicoG-Processor/PicoG-Core/Resource/Resource.lvclass"}, {"Path"=path "C:/dev/Vireo/PicoG/Builds/picoG/ppl/PicoG-Core.lvlibp", "Name"="PicoG-Core.lvlibp", "Referrer"=path "C:/dev/Vireo/PicoG/Builds/picoG/ppl/PicoG-Core.lvlibp/PicoG-Processor/PicoG-Core/Resource/Resource.lvclass"}, {"Path"=path "C:/dev/Vireo/PicoG/Builds/picoG/ppl/PicoG-Core.lvlibp/PicoG-Processor/PicoG-Core/Resource/Resource.lvclass/Resource.ctl", "Name"="PicoG-Core.lvlibp:Resource.lvclass:Resource.ctl", "Referrer"=path "C:/dev/Vireo/PicoG/Builds/picoG/ppl/PicoG-Core.lvlibp/PicoG-Processor/PicoG-Core/Resource/Resource.lvclass"}, {"Path"=path "C:/dev/Vireo/PicoG/Builds/picoG/ppl/PicoG-Core.lvlibp/PicoG-Processor/PicoG-Core/Resource/Get Config.vi", "Name"="PicoG-Core.lvlibp:Resource.lvclass:Get Config.vi", "Referrer"=path "C:/dev/Vireo/PicoG/Builds/picoG/ppl/PicoG-Core.lvlibp/PicoG-Processor/PicoG-Core/Resource/Resource.lvclass"}, {"Path"=path "C:/dev/Vireo/PicoG/Builds/picoG/ppl/PicoG-Core.lvlibp/PicoG-Processor/PicoG-Core/Resource/Set Config.vi", "Name"="PicoG-Core.lvlibp:Resource.lvclass:Set Config.vi", "Referrer"=path "C:/dev/Vireo/PicoG/Builds/picoG/ppl/PicoG-Core.lvlibp/PicoG-Processor/PicoG-Core/Resource/Resource.lvclass"}, {"Path"=path "C:/dev/Vireo/PicoG/Builds/picoG/ppl/PicoG-Core.lvlibp/PicoG-Processor/PicoG-Core/Resource/Friendly Name.vi", "Name"="PicoG-Core.lvlibp:Resource.lvclass:Friendly Name.vi", "Referrer"=path "C:/dev/Vireo/PicoG/Builds/picoG/ppl/PicoG-Core.lvlibp/PicoG-Processor/PicoG-Core/Resource/Resource.lvclass"}, {"Path"=path "C:/dev/Vireo/PicoG/Builds/picoG/ppl/PicoG-Core.lvlibp/PicoG-Processor/PicoG-Core/Resource/Resource Type.vi", "Name"="PicoG-Core.lvlibp:Resource.lvclass:Resource Type.vi", "Referrer"=path "C:/dev/Vireo/PicoG/Builds/picoG/ppl/PicoG-Core.lvlibp/PicoG-Processor/PicoG-Core/Resource/Resource.lvclass"}, {"Path"=path "C:/dev/Vireo/PicoG/Builds/picoG/ppl/PicoG-Core.lvlibp/PicoG-Processor/PicoG-Core/Resource/_Config Updated.vi", "Name"="PicoG-Core.lvlibp:Resource.lvclass:_Config Updated.vi", "Referrer"=path "C:/dev/Vireo/PicoG/Builds/picoG/ppl/PicoG-Core.lvlibp/PicoG-Processor/PicoG-Core/Resource/Resource.lvclass"}, {"Path"=path "C:/dev/Vireo/PicoG/Builds/picoG/ppl/PicoG-Core.lvlibp/PicoG-Processor/PicoG-Core/Resource/_Read.vi", "Name"="PicoG-Core.lvlibp:Resource.lvclass:_Read.vi", "Referrer"=path "C:/dev/Vireo/PicoG/Builds/picoG/ppl/PicoG-Core.lvlibp/PicoG-Processor/PicoG-Core/Resource/Resource.lvclass"}, {"Path"=path "C:/dev/Vireo/PicoG/Builds/picoG/ppl/PicoG-Core.lvlibp/PicoG-Processor/PicoG-Core/Resource/_Write.vi", "Name"="PicoG-Core.lvlibp:Resource.lvclass:_Write.vi", "Referrer"=path "C:/dev/Vireo/PicoG/Builds/picoG/ppl/PicoG-Core.lvlibp/PicoG-Processor/PicoG-Core/Resource/Resource.lvclass"}, {"Path"=path "C:/dev/Vireo/PicoG/Builds/picoG/ppl/PicoG-Core.lvlibp/PicoG-Processor/PicoG-Core/Resource/Config Item.ctl", "Name"="PicoG-Core.lvlibp:Resource.lvclass:Config Item.ctl", "Referrer"=path "C:/dev/Vireo/PicoG/Builds/picoG/ppl/PicoG-Core.lvlibp/PicoG-Processor/PicoG-Core/Resource/Resource.lvclass"}, {"Path"=path "C:/dev/Vireo/PicoG/Builds/picoG/ppl/PicoG-Core.lvlibp/PicoG-Processor/PicoG-Core/Resource/Read Version.vi", "Name"="PicoG-Core.lvlibp:Resource.lvclass:Read Version.vi", "Referrer"=path "C:/dev/Vireo/PicoG/Builds/picoG/ppl/PicoG-Core.lvlibp/PicoG-Processor/PicoG-Core/Resource/Resource.lvclass"}, {"Path"=path "C:/dev/Vireo/PicoG/Builds/picoG/ppl/PicoG-Core.lvlibp/PicoG-Processor/PicoG-Core/Resource/Read Alias.vi", "Name"="PicoG-Core.lvlibp:Resource.lvclass:Read Alias.vi", "Referrer"=path "C:/dev/Vireo/PicoG/Builds/picoG/ppl/PicoG-Core.lvlibp/PicoG-Processor/PicoG-Core/Resource/Resource.lvclass"}, {"Path"=path "C:/dev/Vireo/PicoG/Builds/picoG/ppl/PicoG-Core.lvlibp/PicoG-Processor/PicoG-Core/Resource/Write Alias.vi", "Name"="PicoG-Core.lvlibp:Resource.lvclass:Write Alias.vi", "Referrer"=path "C:/dev/Vireo/PicoG/Builds/picoG/ppl/PicoG-Core.lvlibp/PicoG-Processor/PicoG-Core/Resource/Resource.lvclass"}, {"Path"=path "C:/dev/Vireo/PicoG/Builds/picoG/ppl/PicoG-Core.lvlibp/PicoG-Processor/PicoG-Core/Resource/Read ID.vi", "Name"="PicoG-Core.lvlibp:Resource.lvclass:Read ID.vi", "Referrer"=path "C:/dev/Vireo/PicoG/Builds/picoG/ppl/PicoG-Core.lvlibp/PicoG-Processor/PicoG-Core/Resource/Resource.lvclass"}, {"Path"=path "C:/dev/Vireo/PicoG/Builds/picoG/ppl/PicoG-Core.lvlibp/PicoG-Processor/PicoG-Core/Resource/Read Board.vi", "Name"="PicoG-Core.lvlibp:Resource.lvclass:Read Board.vi", "Referrer"=path "C:/dev/Vireo/PicoG/Builds/picoG/ppl/PicoG-Core.lvlibp/PicoG-Processor/PicoG-Core/Resource/Resource.lvclass"}, {"Path"=path "C:/dev/Vireo/PicoG/Builds/picoG/ppl/PicoG-Core.lvlibp/PicoG-Processor/PicoG-Core/Resource/Read Platform.vi", "Name"="PicoG-Core.lvlibp:Resource.lvclass:Read Platform.vi", "Referrer"=path "C:/dev/Vireo/PicoG/Builds/picoG/ppl/PicoG-Core.lvlibp/PicoG-Processor/PicoG-Core/Resource/Resource.lvclass"}, {"Path"=path "C:/dev/Vireo/PicoG/Builds/picoG/ppl/PicoG-Core.lvlibp/PicoG-Processor/PicoG-Core/Resource/Close.vi", "Name"="PicoG-Core.lvlibp:Resource.lvclass:Close.vi", "Referrer"=path "C:/dev/Vireo/PicoG/Builds/picoG/ppl/PicoG-Core.lvlibp/PicoG-Processor/PicoG-Core/Resource/Resource.lvclass"}, {"Path"=path "C:/dev/Vireo/PicoG/Builds/picoG/ppl/PicoG-Core.lvlibp/PicoG-Processor/PicoG-Core/Resource/Abort.vi", "Name"="PicoG-Core.lvlibp:Resource.lvclass:Abort.vi", "Referrer"=path "C:/dev/Vireo/PicoG/Builds/picoG/ppl/PicoG-Core.lvlibp/PicoG-Processor/PicoG-Core/Resource/Resource.lvclass"}, {"Path"=path "C:/dev/Vireo/PicoG/Builds/picoG/ppl/PicoG-Core.lvlibp/PicoG-Processor/PicoG-Core/Resource/Is At Prompt.vi", "Name"="PicoG-Core.lvlibp:Resource.lvclass:Is At Prompt.vi", "Referrer"=path "C:/dev/Vireo/PicoG/Builds/picoG/ppl/PicoG-Core.lvlibp/PicoG-Processor/PicoG-Core/Resource/Resource.lvclass"}, {"Path"=path "C:/dev/Vireo/PicoG/Builds/picoG/ppl/PicoG-Core.lvlibp/PicoG-Processor/PicoG-Core/Resource/Open.vi", "Name"="PicoG-Core.lvlibp:Resource.lvclass:Open.vi", "Referrer"=path "C:/dev/Vireo/PicoG/Builds/picoG/ppl/PicoG-Core.lvlibp/PicoG-Processor/PicoG-Core/Resource/Resource.lvclass"}, {"Path"=path "C:/dev/Vireo/PicoG/Builds/picoG/ppl/PicoG-Core.lvlibp/PicoG-Processor/PicoG-Core/Resource/Read Until Match.vi", "Name"="PicoG-Core.lvlibp:Resource.lvclass:Read Until Match.vi", "Referrer"=path "C:/dev/Vireo/PicoG/Builds/picoG/ppl/PicoG-Core.lvlibp/PicoG-Processor/PicoG-Core/Resource/Resource.lvclass"}, {"Path"=path "C:/dev/Vireo/PicoG/Builds/picoG/ppl/PicoG-Core.lvlibp/PicoG-Processor/PicoG-Core/Resource/Read.vi", "Name"="PicoG-Core.lvlibp:Resource.lvclass:Read.vi", "Referrer"=path "C:/dev/Vireo/PicoG/Builds/picoG/ppl/PicoG-Core.lvlibp/PicoG-Processor/PicoG-Core/Resource/Resource.lvclass"}, {"Path"=path "C:/dev/Vireo/PicoG/Builds/picoG/ppl/PicoG-Core.lvlibp/PicoG-Processor/PicoG-Core/Resource/Write.vi", "Name"="PicoG-Core.lvlibp:Resource.lvclass:Write.vi", "Referrer"=path "C:/dev/Vireo/PicoG/Builds/picoG/ppl/PicoG-Core.lvlibp/PicoG-Processor/PicoG-Core/Resource/Resource.lvclass"}, {"Path"=path "C:/dev/Vireo/PicoG/PicoG-App/Device/Resource Ref.ctl", "Name"="PicoG-App.lvlib:Device.lvclass:Resource Ref.ctl", "Referrer"=path "C:/dev/Vireo/PicoG/PicoG-App/Device/Resource Ref.ctl"}, {"Path"=path "../Device.lvclass", "Name"="PicoG-App.lvlib:Device.lvclass", "Referrer"=path "C:/dev/Vireo/PicoG/PicoG-App/Device/Resource Ref.ctl"}, {"Path"=path "../../../Builds/picoG/ppl/PicoG-Core.lvlibp/PicoG-Processor/PicoG-Core/Resource/Resource.lvclass", "Name"="PicoG-Core.lvlibp:Resource.lvclass", "Referrer"=path "C:/dev/Vireo/PicoG/PicoG-App/Device/Resource Ref.ctl"}, {"Path"=path "C:/dev/Vireo/PicoG/PicoG-App/Device/Ref Data.ctl", "Name"="PicoG-App.lvlib:Device.lvclass:Ref Data.ctl", "Referrer"=path "C:/dev/Vireo/PicoG/PicoG-App/Device/Ref Data.ctl"}, {"Path"=path "../Device.lvclass", "Name"="PicoG-App.lvlib:Device.lvclass", "Referrer"=path "C:/dev/Vireo/PicoG/PicoG-App/Device/Ref Data.ctl"}, {"Path"=path "../Device Key.ctl", "Name"="PicoG-App.lvlib:Device.lvclass:Device Key.ctl", "Referrer"=path "C:/dev/Vireo/PicoG/PicoG-App/Device/Ref Data.ctl"}, {"Path"=path "C:/dev/Vireo/PicoG/PicoG-App/Device/Device Key.ctl", "Name"="PicoG-App.lvlib:Device.lvclass:Device Key.ctl", "Referrer"=path "C:/dev/Vireo/PicoG/PicoG-App/Device/Device Key.ctl"}, {"Path"=path "../Device.lvclass", "Name"="PicoG-App.lvlib:Device.lvclass", "Referrer"=path "C:/dev/Vireo/PicoG/PicoG-App/Device/Device Key.ctl"}, {"Path"=path "C:/dev/Vireo/PicoG/PicoG-App/Device/Device.lvclass/Device.ctl", "Name"="PicoG-App.lvlib:Device.lvclass:Device.ctl", "Referrer"=path "C:/dev/Vireo/PicoG/PicoG-App/Device/Device.lvclass/Device.ctl"}, {"Path"=path "..", "Name"="PicoG-App.lvlib:Device.lvclass", "Referrer"=path "C:/dev/Vireo/PicoG/PicoG-App/Device/Device.lvclass/Device.ctl"}, {"Path"=path "../../Ref Data.ctl", "Name"="PicoG-App.lvlib:Device.lvclass:Ref Data.ctl", "Referrer"=path "C:/dev/Vireo/PicoG/PicoG-App/Device/Device.lvclass/Device.ctl"}, {"Path"=path "../../Device Key.ctl", "Name"="PicoG-App.lvlib:Device.lvclass:Device Key.ctl", "Referrer"=path "C:/dev/Vireo/PicoG/PicoG-App/Device/Device.lvclass/Device.ctl"}, {"Path"=path "../../Resource Ref.ctl", "Name"="PicoG-App.lvlib:Device.lvclass:Resource Ref.ctl", "Referrer"=path "C:/dev/Vireo/PicoG/PicoG-App/Device/Device.lvclass/Device.ctl"}, {"Path"=path "../../../../Builds/picoG/ppl/PicoG-Core.lvlibp/PicoG-Processor/PicoG-Core/Resource/Resource.lvclass", "Name"="PicoG-Core.lvlibp:Resource.lvclass", "Referrer"=path "C:/dev/Vireo/PicoG/PicoG-App/Device/Device.lvclass/Device.ctl"}, {"Path"=path "C:/dev/Vireo/PicoG/PicoG-App/Device/Get Platform Name.vi", "Name"="PicoG-App.lvlib:Device.lvclass:Get Platform Name.vi", "Referrer"=path "C:/dev/Vireo/PicoG/PicoG-App/Device/Get Platform Name.vi"}, {"Path"=path "../Device.lvclass", "Name"="PicoG-App.lvlib:Device.lvclass", "Referrer"=path "C:/dev/Vireo/PicoG/PicoG-App/Device/Get Platform Name.vi"}, {"Path"=path "../Device.lvclass/Device.ctl", "Name"="PicoG-App.lvlib:Device.lvclass:Device.ctl", "Referrer"=path "C:/dev/Vireo/PicoG/PicoG-App/Device/Get Platform Name.vi"}, {"Path"=path "C:/dev/Vireo/PicoG/PicoG-App/Device/Get Board.vi", "Name"="PicoG-App.lvlib:Device.lvclass:Get Board.vi", "Referrer"=path "C:/dev/Vireo/PicoG/PicoG-App/Device/Get Board.vi"}, {"Path"=path "../Device.lvclass", "Name"="PicoG-App.lvlib:Device.lvclass", "Referrer"=path "C:/dev/Vireo/PicoG/PicoG-App/Device/Get Board.vi"}, {"Path"=path "../Device.lvclass/Device.ctl", "Name"="PicoG-App.lvlib:Device.lvclass:Device.ctl", "Referrer"=path "C:/dev/Vireo/PicoG/PicoG-App/Device/Get Board.vi"}, {"Path"=path "C:/dev/Vireo/PicoG/PicoG-App/Device/Get ID.vi", "Name"="PicoG-App.lvlib:Device.lvclass:Get ID.vi", "Referrer"=path "C:/dev/Vireo/PicoG/PicoG-App/Device/Get ID.vi"}, {"Path"=path "../Device.lvclass", "Name"="PicoG-App.lvlib:Device.lvclass", "Referrer"=path "C:/dev/Vireo/PicoG/PicoG-App/Device/Get ID.vi"}, {"Path"=path "../Device.lvclass/Device.ctl", "Name"="PicoG-App.lvlib:Device.lvclass:Device.ctl", "Referrer"=path "C:/dev/Vireo/PicoG/PicoG-App/Device/Get ID.vi"}, {"Path"=path "C:/dev/Vireo/PicoG/PicoG-App/Device/Get Alias.vi", "Name"="PicoG-App.lvlib:Device.lvclass:Get Alias.vi", "Referrer"=path "C:/dev/Vireo/PicoG/PicoG-App/Device/Get Alias.vi"}, {"Path"=path "../Device.lvclass", "Name"="PicoG-App.lvlib:Device.lvclass", "Referrer"=path "C:/dev/Vireo/PicoG/PicoG-App/Device/Get Alias.vi"}, {"Path"=path "../Device.lvclass/Device.ctl", "Name"="PicoG-App.lvlib:Device.lvclass:Device.ctl", "Referrer"=path "C:/dev/Vireo/PicoG/PicoG-App/Device/Get Alias.vi"}, {"Path"=path "C:/dev/Vireo/PicoG/PicoG-App/Device/Get Version String.vi", "Name"="PicoG-App.lvlib:Device.lvclass:Get Version String.vi", "Referrer"=path "C:/dev/Vireo/PicoG/PicoG-App/Device/Get Version String.vi"}, {"Path"=path "../Device.lvclass", "Name"="PicoG-App.lvlib:Device.lvclass", "Referrer"=path "C:/dev/Vireo/PicoG/PicoG-App/Device/Get Version String.vi"}, {"Path"=path "../Device.lvclass/Device.ctl", "Name"="PicoG-App.lvlib:Device.lvclass:Device.ctl", "Referrer"=path "C:/dev/Vireo/PicoG/PicoG-App/Device/Get Version String.vi"}, {"Path"=path "C:/dev/Vireo/PicoG/PicoG-App/DeviceListPanel/Ref Data.ctl", "Name"="PicoG-App.lvlib:DeviceListPanel.lvclass:Ref Data.ctl", "Referrer"=path "C:/dev/Vireo/PicoG/PicoG-App/DeviceListPanel/Ref Data.ctl"}, {"Path"=path "../DeviceListPanel.lvclass", "Name"="PicoG-App.lvlib:DeviceListPanel.lvclass", "Referrer"=path "C:/dev/Vireo/PicoG/PicoG-App/DeviceListPanel/Ref Data.ctl"}, {"Path"=path "../../Device/Device Key.ctl", "Name"="PicoG-App.lvlib:Device.lvclass:Device Key.ctl", "Referrer"=path "C:/dev/Vireo/PicoG/PicoG-App/DeviceListPanel/Ref Data.ctl"}, {"Path"=path "../Device and Panel.ctl", "Name"="PicoG-App.lvlib:DeviceListPanel.lvclass:Device and Panel.ctl", "Referrer"=path "C:/dev/Vireo/PicoG/PicoG-App/DeviceListPanel/Ref Data.ctl"}, {"Path"=path "../../Device/Device.lvclass", "Name"="PicoG-App.lvlib:Device.lvclass", "Referrer"=path "C:/dev/Vireo/PicoG/PicoG-App/DeviceListPanel/Ref Data.ctl"}, {"Path"=path "../../DeviceArrayPanel/DeviceArrayPanel.lvclass", "Name"="PicoG-App.lvlib:DeviceArrayPanel.lvclass", "Referrer"=path "C:/dev/Vireo/PicoG/PicoG-App/DeviceListPanel/Ref Data.ctl"}, {"Path"=path "C:/dev/Vireo/PicoG/PicoG-App/DeviceListPanel/Device and Panel.ctl", "Name"="PicoG-App.lvlib:DeviceListPanel.lvclass:Device and Panel.ctl", "Referrer"=path "C:/dev/Vireo/PicoG/PicoG-App/DeviceListPanel/Device and Panel.ctl"}, {"Path"=path "../DeviceListPanel.lvclass", "Name"="PicoG-App.lvlib:DeviceListPanel.lvclass", "Referrer"=path "C:/dev/Vireo/PicoG/PicoG-App/DeviceListPanel/Device and Panel.ctl"}, {"Path"=path "../../Device/Device.lvclass", "Name"="PicoG-App.lvlib:Device.lvclass", "Referrer"=path "C:/dev/Vireo/PicoG/PicoG-App/DeviceListPanel/Device and Panel.ctl"}, {"Path"=path "../../DeviceArrayPanel/DeviceArrayPanel.lvclass", "Name"="PicoG-App.lvlib:DeviceArrayPanel.lvclass", "Referrer"=path "C:/dev/Vireo/PicoG/PicoG-App/DeviceListPanel/Device and Panel.ctl"}, {"Path"=path "C:/dev/Vireo/PicoG/PicoG-App/DeviceListPanel/Outbound Events.ctl", "Name"="PicoG-App.lvlib:DeviceListPanel.lvclass:Outbound Events.ctl", "Referrer"=path "C:/dev/Vireo/PicoG/PicoG-App/DeviceListPanel/Outbound Events.ctl"}, {"Path"=path "../DeviceListPanel.lvclass", "Name"="PicoG-App.lvlib:DeviceListPanel.lvclass", "Referrer"=path "C:/dev/Vireo/PicoG/PicoG-App/DeviceListPanel/Outbound Events.ctl"}, {"Path"=path "../../Device/Device.lvclass", "Name"="PicoG-App.lvlib:Device.lvclass", "Referrer"=path "C:/dev/Vireo/PicoG/PicoG-App/DeviceListPanel/Outbound Events.ctl"}, {"Path"=path "C:/dev/Vireo/PicoG/PicoG-App/DeviceListPanel/Inbound Events.ctl", "Name"="PicoG-App.lvlib:DeviceListPanel.lvclass:Inbound Events.ctl", "Referrer"=path "C:/dev/Vireo/PicoG/PicoG-App/DeviceListPanel/Inbound Events.ctl"}, {"Path"=path "../DeviceListPanel.lvclass", "Name"="PicoG-App.lvlib:DeviceListPanel.lvclass", "Referrer"=path "C:/dev/Vireo/PicoG/PicoG-App/DeviceListPanel/Inbound Events.ctl"}, {"Path"=path "../../Device/Device.lvclass", "Name"="PicoG-App.lvlib:Device.lvclass", "Referrer"=path "C:/dev/Vireo/PicoG/PicoG-App/DeviceListPanel/Inbound Events.ctl"}, {"Path"=path "C:/dev/Vireo/PicoG/PicoG-App/DeviceArrayPanel/DeviceArrayPanel.lvclass/DeviceArrayPanel.ctl", "Name"="PicoG-App.lvlib:DeviceArrayPanel.lvclass:DeviceArrayPanel.ctl", "Referrer"=path "C:/dev/Vireo/PicoG/PicoG-App/DeviceArrayPanel/DeviceArrayPanel.lvclass/DeviceArrayPanel.ctl"}, {"Path"=path "..", "Name"="PicoG-App.lvlib:DeviceArrayPanel.lvclass", "Referrer"=path "C:/dev/Vireo/PicoG/PicoG-App/DeviceArrayPanel/DeviceArrayPanel.lvclass/DeviceArrayPanel.ctl"}, {"Path"=path "../../Ref Data.ctl", "Name"="PicoG-App.lvlib:DeviceArrayPanel.lvclass:Ref Data.ctl", "Referrer"=path "C:/dev/Vireo/PicoG/PicoG-App/DeviceArrayPanel/DeviceArrayPanel.lvclass/DeviceArrayPanel.ctl"}, {"Path"=path "../../../Device/Device.lvclass", "Name"="PicoG-App.lvlib:Device.lvclass", "Referrer"=path "C:/dev/Vireo/PicoG/PicoG-App/DeviceArrayPanel/DeviceArrayPanel.lvclass/DeviceArrayPanel.ctl"}, {"Path"=path "../../Inbound Events.ctl", "Name"="PicoG-App.lvlib:DeviceArrayPanel.lvclass:Inbound Events.ctl", "Referrer"=path "C:/dev/Vireo/PicoG/PicoG-App/DeviceArrayPanel/DeviceArrayPanel.lvclass/DeviceArrayPanel.ctl"}, {"Path"=path "C:/dev/Vireo/PicoG/PicoG-App/ViaApp/Get Updated.vi", "Name"="PicoG-App.lvlib:ViaApp.lvclass:Get Updated.vi", "Referrer"=path "C:/dev/Vireo/PicoG/PicoG-App/ViaApp/Get Updated.vi"}, {"Path"=path "../ViaApp.lvclass", "Name"="PicoG-App.lvlib:ViaApp.lvclass", "Referrer"=path "C:/dev/Vireo/PicoG/PicoG-App/ViaApp/Get Updated.vi"}, {"Path"=path "../ViaApp.lvclass/ViaApp.ctl", "Name"="PicoG-App.lvlib:ViaApp.lvclass:ViaApp.ctl", "Referrer"=path "C:/dev/Vireo/PicoG/PicoG-App/ViaApp/Get Updated.vi"}, {"Path"=path "C:/dev/Vireo/PicoG/PicoG-App/ViaApp/Set Updated.vi", "Name"="PicoG-App.lvlib:ViaApp.lvclass:Set Updated.vi", "Referrer"=path "C:/dev/Vireo/PicoG/PicoG-App/ViaApp/Set Updated.vi"}, {"Path"=path "../ViaApp.lvclass", "Name"="PicoG-App.lvlib:ViaApp.lvclass", "Referrer"=path "C:/dev/Vireo/PicoG/PicoG-App/ViaApp/Set Updated.vi"}, {"Path"=path "../ViaApp.lvclass/ViaApp.ctl", "Name"="PicoG-App.lvlib:ViaApp.lvclass:ViaApp.ctl", "Referrer"=path "C:/dev/Vireo/PicoG/PicoG-App/ViaApp/Set Updated.vi"}, {"Path"=path "C:/dev/Vireo/PicoG/Builds/picoG/ppl/PicoG-Core.lvlibp/1abvi3w/vi.lib/Utility/LVLibp/NI_PackedLibraryUtility.lvlib", "Name"="PicoG-Core.lvlibp:NI_PackedLibraryUtility.lvlib", "Referrer"=path "C:/dev/Vireo/PicoG/Builds/picoG/ppl/PicoG-Core.lvlibp/1abvi3w/vi.lib/Utility/LVLibp/NI_PackedLibraryUtility.lvlib"}, {"Path"=path "C:/dev/Vireo/PicoG/Builds/picoG/ppl/PicoG-Core.lvlibp", "Name"="PicoG-Core.lvlibp", "Referrer"=path "C:/dev/Vireo/PicoG/Builds/picoG/ppl/PicoG-Core.lvlibp/1abvi3w/vi.lib/Utility/LVLibp/NI_PackedLibraryUtility.lvlib"}, {"Path"=path "C:/dev/Vireo/PicoG/Builds/picoG/ppl/PicoG-Core.lvlibp/1abvi3w/vi.lib/Utility/LVLibp/Get Exported File List.vi", "Name"="PicoG-Core.lvlibp:NI_PackedLibraryUtility.lvlib:Get Exported File List.vi", "Referrer"=path "C:/dev/Vireo/PicoG/Builds/picoG/ppl/PicoG-Core.lvlibp/1abvi3w/vi.lib/Utility/LVLibp/NI_PackedLibraryUtility.lvlib"}, {"Path"=path "C:/dev/Vireo/PicoG/Builds/picoG/ppl/PicoG-Core.lvlibp", "Name"="PicoG-Core.lvlibp", "Referrer"=path "C:/dev/Vireo/PicoG/Builds/picoG/ppl/PicoG-Core.lvlibp"}, {"Path"=path "C:/dev/Vireo/PicoG/Builds/picoG/ppl/PicoG-Core.lvlibp/PicoG-Processor/PicoG-Core/Command Header Const.vi", "Name"="PicoG-Core.lvlibp:Command Header Const.vi", "Referrer"=path "C:/dev/Vireo/PicoG/Builds/picoG/ppl/PicoG-Core.lvlibp"}, {"Path"=path "C:/dev/Vireo/PicoG/Builds/picoG/ppl/PicoG-Core.lvlibp/PicoG-Processor/PicoG-Core/Command.ctl", "Name"="PicoG-Core.lvlibp:Command.ctl", "Referrer"=path "C:/dev/Vireo/PicoG/Builds/picoG/ppl/PicoG-Core.lvlibp"}, {"Path"=path "C:/dev/Vireo/PicoG/Builds/picoG/ppl/PicoG-Core.lvlibp/PicoG-Processor/minivia.vi", "Name"="PicoG-Core.lvlibp:minivia.vi", "Referrer"=path "C:/dev/Vireo/PicoG/Builds/picoG/ppl/PicoG-Core.lvlibp"}, {"Path"=path "C:/dev/Vireo/PicoG/Builds/picoG/ppl/PicoG-Core.lvlibp/PicoG-Processor/PicoG-Core/From 8601UTC.vi", "Name"="PicoG-Core.lvlibp:From 8601UTC.vi", "Referrer"=path "C:/dev/Vireo/PicoG/Builds/picoG/ppl/PicoG-Core.lvlibp"}, {"Path"=path "C:/dev/Vireo/PicoG/Builds/picoG/ppl/PicoG-Core.lvlibp/PicoG-Processor/Remove Whitespace from VIA.vi", "Name"="PicoG-Core.lvlibp:Remove Whitespace from VIA.vi", "Referrer"=path "C:/dev/Vireo/PicoG/Builds/picoG/ppl/PicoG-Core.lvlibp"}, {"Path"=path "C:/dev/Vireo/PicoG/Builds/picoG/ppl/PicoG-Core.lvlibp/Reuse/VIA Minify all VIs.vi", "Name"="PicoG-Core.lvlibp:VIA Minify all VIs.vi", "Referrer"=path "C:/dev/Vireo/PicoG/Builds/picoG/ppl/PicoG-Core.lvlibp"}, {"Path"=path "C:/dev/Vireo/PicoG/Builds/picoG/ppl/PicoG-Core.lvlibp/Reuse/VIA Minify VI Constants.vi", "Name"="PicoG-Core.lvlibp:VIA Minify VI Constants.vi", "Referrer"=path "C:/dev/Vireo/PicoG/Builds/picoG/ppl/PicoG-Core.lvlibp"}, {"Path"=path "C:/dev/Vireo/PicoG/Builds/picoG/ppl/PicoG-Core.lvlibp/Reuse/VIA Minify VI Locals.vi", "Name"="PicoG-Core.lvlibp:VIA Minify VI Locals.vi", "Referrer"=path "C:/dev/Vireo/PicoG/Builds/picoG/ppl/PicoG-Core.lvlibp"}, {"Path"=path "C:/dev/Vireo/PicoG/Builds/picoG/ppl/PicoG-Core.lvlibp/Reuse/Insert Replacement String.vi", "Name"="PicoG-Core.lvlibp:Insert Replacement String.vi", "Referrer"=path "C:/dev/Vireo/PicoG/Builds/picoG/ppl/PicoG-Core.lvlibp"}, {"Path"=path "C:/dev/Vireo/PicoG/Builds/picoG/ppl/PicoG-Core.lvlibp/PicoG-Processor/PicoG-Core/VisaResource/VisaResource.lvclass", "Name"="PicoG-Core.lvlibp:VisaResource.lvclass", "Referrer"=path "C:/dev/Vireo/PicoG/Builds/picoG/ppl/PicoG-Core.lvlibp"}, {"Path"=path "C:/dev/Vireo/PicoG/Builds/picoG/ppl/PicoG-Core.lvlibp/PicoG-Processor/PicoG-Core/Platform/Platform.lvclass", "Name"="PicoG-Core.lvlibp:Platform.lvclass", "Referrer"=path "C:/dev/Vireo/PicoG/Builds/picoG/ppl/PicoG-Core.lvlibp"}, {"Path"=path "C:/dev/Vireo/PicoG/Builds/picoG/ppl/PicoG-Core.lvlibp/PicoG-Processor/PicoG-Core/Resource/Resource.lvclass", "Name"="PicoG-Core.lvlibp:Resource.lvclass", "Referrer"=path "C:/dev/Vireo/PicoG/Builds/picoG/ppl/PicoG-Core.lvlibp"}, {"Path"=path "C:/dev/Vireo/PicoG/Builds/picoG/ppl/PicoG-Core.lvlibp/PicoG-Processor/PicoG-Core/PlatformManager/PlatformManager.lvclass", "Name"="PicoG-Core.lvlibp:PlatformManager.lvclass", "Referrer"=path "C:/dev/Vireo/PicoG/Builds/picoG/ppl/PicoG-Core.lvlibp"}, {"Path"=path "C:/dev/Vireo/PicoG/Builds/picoG/ppl/PicoG-Core.lvlibp/PicoG-Processor/PicoG-Core/Terminal/Terminal.lvclass", "Name"="PicoG-Core.lvlibp:Terminal.lvclass", "Referrer"=path "C:/dev/Vireo/PicoG/Builds/picoG/ppl/PicoG-Core.lvlibp"}, {"Path"=path "C:/dev/Vireo/PicoG/Builds/picoG/ppl/PicoG-Core.lvlibp/PicoG-Processor/PicoG-Core/Create Error.vi", "Name"="PicoG-Core.lvlibp:Create Error.vi", "Referrer"=path "C:/dev/Vireo/PicoG/Builds/picoG/ppl/PicoG-Core.lvlibp"}, {"Path"=path "C:/dev/Vireo/PicoG/Builds/picoG/ppl/PicoG-Core.lvlibp/1abvi3w/vi.lib/Utility/LVLibp/NI_PackedLibraryUtility.lvlib", "Name"="PicoG-Core.lvlibp:NI_PackedLibraryUtility.lvlib", "Referrer"=path "C:/dev/Vireo/PicoG/Builds/picoG/ppl/PicoG-Core.lvlibp"}, {"Path"=path "C:/dev/Vireo/PicoG/Builds/picoG/ppl/PicoG-Core.lvlibp/1abvi3w/vi.lib/Comparison/Equal/Equal Functor/Equal Functor.lvclass", "Name"="PicoG-Core.lvlibp:Equal Functor.lvclass", "Referrer"=path "C:/dev/Vireo/PicoG/Builds/picoG/ppl/PicoG-Core.lvlibp"}, {"Path"=path "C:/dev/Vireo/PicoG/Builds/picoG/ppl/PicoG-Core.lvlibp/1abvi3w/vi.lib/Comparison/Equal/Equal Comparable/Equal Comparable.lvclass", "Name"="PicoG-Core.lvlibp:Equal Comparable.lvclass", "Referrer"=path "C:/dev/Vireo/PicoG/Builds/picoG/ppl/PicoG-Core.lvlibp"}, {"Path"=path "C:/dev/Vireo/PicoG/Builds/picoG/ppl/PicoG-Core.lvlibp/1abvi3w/vi.lib/Comparison/Less/Less Functor/Less Functor.lvclass", "Name"="PicoG-Core.lvlibp:Less Functor.lvclass", "Referrer"=path "C:/dev/Vireo/PicoG/Builds/picoG/ppl/PicoG-Core.lvlibp"}, {"Path"=path "C:/dev/Vireo/PicoG/Builds/picoG/ppl/PicoG-Core.lvlibp/1abvi3w/vi.lib/Comparison/Less/Less Comparable/Less Comparable.lvclass", "Name"="PicoG-Core.lvlibp:Less Comparable.lvclass", "Referrer"=path "C:/dev/Vireo/PicoG/Builds/picoG/ppl/PicoG-Core.lvlibp"}, {"Path"=path "C:/dev/Vireo/PicoG/Builds/picoG/ppl/PicoG-Core.lvlibp/1abvi3w/vi.lib/Utility/error.llb/Error Cluster From Error Code.vi", "Name"="PicoG-Core.lvlibp:Error Cluster From Error Code.vi", "Referrer"=path "C:/dev/Vireo/PicoG/Builds/picoG/ppl/PicoG-Core.lvlibp"}, {"Path"=path "C:/dev/Vireo/PicoG/Builds/picoG/ppl/PicoG-Core.lvlibp/1abvi3w/vi.lib/Utility/LVClass/Get LV Class Default Value.vi", "Name"="PicoG-Core.lvlibp:Get LV Class Default Value.vi", "Referrer"=path "C:/dev/Vireo/PicoG/Builds/picoG/ppl/PicoG-Core.lvlibp"}, {"Path"=path "C:/dev/Vireo/PicoG/Builds/picoG/ppl/PicoG-Core.lvlibp/1abvi3w/vi.lib/AdvancedString/Delimited String to 1D String Array.vi", "Name"="PicoG-Core.lvlibp:Delimited String to 1D String Array.vi", "Referrer"=path "C:/dev/Vireo/PicoG/Builds/picoG/ppl/PicoG-Core.lvlibp"}, {"Path"=path "C:/dev/Vireo/PicoG/Builds/picoG/ppl/PicoG-Core.lvlibp/1abvi3w/vi.lib/Utility/error.llb/Search and Replace Pattern.vi", "Name"="PicoG-Core.lvlibp:Search and Replace Pattern.vi", "Referrer"=path "C:/dev/Vireo/PicoG/Builds/picoG/ppl/PicoG-Core.lvlibp"}, {"Path"=path "C:/dev/Vireo/PicoG/Builds/picoG/ppl/PicoG-Core.lvlibp/1abvi3w/vi.lib/Instr/_visa.llb/VISA Configure Serial Port (Instr).vi", "Name"="PicoG-Core.lvlibp:VISA Configure Serial Port (Instr).vi", "Referrer"=path "C:/dev/Vireo/PicoG/Builds/picoG/ppl/PicoG-Core.lvlibp"}, {"Path"=path "C:/dev/Vireo/PicoG/Builds/picoG/ppl/PicoG-Core.lvlibp/1abvi3w/vi.lib/Utility/error.llb/whitespace.ctl", "Name"="PicoG-Core.lvlibp:whitespace.ctl", "Referrer"=path "C:/dev/Vireo/PicoG/Builds/picoG/ppl/PicoG-Core.lvlibp"}, {"Path"=path "C:/dev/Vireo/PicoG/Builds/picoG/ppl/PicoG-Core.lvlibp/1abvi3w/vi.lib/Utility/error.llb/Trim Whitespace.vi", "Name"="PicoG-Core.lvlibp:Trim Whitespace.vi", "Referrer"=path "C:/dev/Vireo/PicoG/Builds/picoG/ppl/PicoG-Core.lvlibp"}, {"Path"=path "C:/dev/Vireo/PicoG/Builds/picoG/ppl/PicoG-Core.lvlibp/1abvi3w/vi.lib/Utility/miscctls.llb/LVDateTimeRec.ctl", "Name"="PicoG-Core.lvlibp:LVDateTimeRec.ctl", "Referrer"=path "C:/dev/Vireo/PicoG/Builds/picoG/ppl/PicoG-Core.lvlibp"}, {"Path"=path "C:/dev/Vireo/PicoG/Builds/picoG/ppl/PicoG-Core.lvlibp/1abvi3w/vi.lib/Utility/error.llb/Error Cluster From Error Code.vi", "Name"="PicoG-Core.lvlibp:Error Cluster From Error Code.vi", "Referrer"=path "C:/dev/Vireo/PicoG/Builds/picoG/ppl/PicoG-Core.lvlibp/1abvi3w/vi.lib/Utility/error.llb/Error Cluster From Error Code.vi"}, {"Path"=path "../../../../..", "Name"="PicoG-Core.lvlibp", "Referrer"=path "C:/dev/Vireo/PicoG/Builds/picoG/ppl/PicoG-Core.lvlibp/1abvi3w/vi.lib/Utility/error.llb/Error Cluster From Error Code.vi"}, {"Path"=path "C:/dev/Vireo/PicoG/Builds/picoG/ppl/PicoG-Core.lvlibp/PicoG-Processor/PicoG-Core/Resource/Config Item.ctl", "Name"="PicoG-Core.lvlibp:Resource.lvclass:Config Item.ctl", "Referrer"=path "C:/dev/Vireo/PicoG/Builds/picoG/ppl/PicoG-Core.lvlibp/PicoG-Processor/PicoG-Core/Resource/Config Item.ctl"}, {"Path"=path "../Resource.lvclass", "Name"="PicoG-Core.lvlibp:Resource.lvclass", "Referrer"=path "C:/dev/Vireo/PicoG/Builds/picoG/ppl/PicoG-Core.lvlibp/PicoG-Processor/PicoG-Core/Resource/Config Item.ctl"}, {"Path"=path "C:/dev/Vireo/PicoG/Builds/picoG/ppl/PicoG-Core.lvlibp/PicoG-Processor/PicoG-Core/Resource/Set Config.vi", "Name"="PicoG-Core.lvlibp:Resource.lvclass:Set Config.vi", "Referrer"=path "C:/dev/Vireo/PicoG/Builds/picoG/ppl/PicoG-Core.lvlibp/PicoG-Processor/PicoG-Core/Resource/Set Config.vi"}, {"Path"=path "../Resource.lvclass", "Name"="PicoG-Core.lvlibp:Resource.lvclass", "Referrer"=path "C:/dev/Vireo/PicoG/Builds/picoG/ppl/PicoG-Core.lvlibp/PicoG-Processor/PicoG-Core/Resource/Set Config.vi"}, {"Path"=path "../Config Item.ctl", "Name"="PicoG-Core.lvlibp:Resource.lvclass:Config Item.ctl", "Referrer"=path "C:/dev/Vireo/PicoG/Builds/picoG/ppl/PicoG-Core.lvlibp/PicoG-Processor/PicoG-Core/Resource/Set Config.vi"}, {"Path"=path "C:/dev/Vireo/PicoG/PicoG-App/Device/Init from Config.vi", "Name"="PicoG-App.lvlib:Device.lvclass:Init from Config.vi", "Referrer"=path "C:/dev/Vireo/PicoG/PicoG-App/Device/Init from Config.vi"}, {"Path"=path "../Device.lvclass", "Name"="PicoG-App.lvlib:Device.lvclass", "Referrer"=path "C:/dev/Vireo/PicoG/PicoG-App/Device/Init from Config.vi"}, {"Path"=path "../Device Key.ctl", "Name"="PicoG-App.lvlib:Device.lvclass:Device Key.ctl", "Referrer"=path "C:/dev/Vireo/PicoG/PicoG-App/Device/Init from Config.vi"}, {"Path"=path "../../../Builds/picoG/ppl/PicoG-Core.lvlibp/PicoG-Processor/PicoG-Core/Resource/Resource.lvclass", "Name"="PicoG-Core.lvlibp:Resource.lvclass", "Referrer"=path "C:/dev/Vireo/PicoG/PicoG-App/Device/Init from Config.vi"}, {"Path"=path "C:/dev/Vireo/PicoG/PicoG-App/Device/Get Resource.vi", "Name"="PicoG-App.lvlib:Device.lvclass:Get Resource.vi", "Referrer"=path "C:/dev/Vireo/PicoG/PicoG-App/Device/Get Resource.vi"}, {"Path"=path "../Device.lvclass", "Name"="PicoG-App.lvlib:Device.lvclass", "Referrer"=path "C:/dev/Vireo/PicoG/PicoG-App/Device/Get Resource.vi"}, {"Path"=path "../../../Builds/picoG/ppl/PicoG-Core.lvlibp/PicoG-Processor/PicoG-Core/Resource/Resource.lvclass", "Name"="PicoG-Core.lvlibp:Resource.lvclass", "Referrer"=path "C:/dev/Vireo/PicoG/PicoG-App/Device/Get Resource.vi"}, {"Path"=path "../Device.lvclass/Device.ctl", "Name"="PicoG-App.lvlib:Device.lvclass:Device.ctl", "Referrer"=path "C:/dev/Vireo/PicoG/PicoG-App/Device/Get Resource.vi"}, {"Path"=path "C:/dev/Vireo/PicoG/PicoG-App/GWebAppArrayPanel/Ref Data.ctl", "Name"="PicoG-App.lvlib:GWebAppArrayPanel.lvclass:Ref Data.ctl", "Referrer"=path "C:/dev/Vireo/PicoG/PicoG-App/GWebAppArrayPanel/Ref Data.ctl"}, {"Path"=path "../GWebAppArrayPanel.lvclass", "Name"="PicoG-App.lvlib:GWebAppArrayPanel.lvclass", "Referrer"=path "C:/dev/Vireo/PicoG/PicoG-App/GWebAppArrayPanel/Ref Data.ctl"}, {"Path"=path "../../ViaApp/ViaApp.lvclass", "Name"="PicoG-App.lvlib:ViaApp.lvclass", "Referrer"=path "C:/dev/Vireo/PicoG/PicoG-App/GWebAppArrayPanel/Ref Data.ctl"}, {"Path"=path "../Outbound Events.ctl", "Name"="PicoG-App.lvlib:GWebAppArrayPanel.lvclass:Outbound Events.ctl", "Referrer"=path "C:/dev/Vireo/PicoG/PicoG-App/GWebAppArrayPanel/Ref Data.ctl"}, {"Path"=path "C:/dev/Vireo/PicoG/PicoG-App/GWebAppArrayPanel/Outbound Events.ctl", "Name"="PicoG-App.lvlib:GWebAppArrayPanel.lvclass:Outbound Events.ctl", "Referrer"=path "C:/dev/Vireo/PicoG/PicoG-App/GWebAppArrayPanel/Outbound Events.ctl"}, {"Path"=path "../GWebAppArrayPanel.lvclass", "Name"="PicoG-App.lvlib:GWebAppArrayPanel.lvclass", "Referrer"=path "C:/dev/Vireo/PicoG/PicoG-App/GWebAppArrayPanel/Outbound Events.ctl"}, {"Path"=path "../../ViaApp/ViaApp.lvclass", "Name"="PicoG-App.lvlib:ViaApp.lvclass", "Referrer"=path "C:/dev/Vireo/PicoG/PicoG-App/GWebAppArrayPanel/Outbound Events.ctl"}, {"Path"=path "C:/dev/Vireo/PicoG/PicoG-App/GWebAppArrayPanel/Panel Events.ctl", "Name"="PicoG-App.lvlib:GWebAppArrayPanel.lvclass:Panel Events.ctl", "Referrer"=path "C:/dev/Vireo/PicoG/PicoG-App/GWebAppArrayPanel/Panel Events.ctl"}, {"Path"=path "../GWebAppArrayPanel.lvclass", "Name"="PicoG-App.lvlib:GWebAppArrayPanel.lvclass", "Referrer"=path "C:/dev/Vireo/PicoG/PicoG-App/GWebAppArrayPanel/Panel Events.ctl"}, {"Path"=path "../../ViaApp/ViaApp.lvclass", "Name"="PicoG-App.lvlib:ViaApp.lvclass", "Referrer"=path "C:/dev/Vireo/PicoG/PicoG-App/GWebAppArrayPanel/Panel Events.ctl"}, {"Path"=path "C:/dev/Vireo/PicoG/PicoG-App/PlatformArrayPanel/Panel Events.ctl", "Name"="PicoG-App.lvlib:PlatformArrayPanel.lvclass:Panel Events.ctl", "Referrer"=path "C:/dev/Vireo/PicoG/PicoG-App/PlatformArrayPanel/Panel Events.ctl"}, {"Path"=path "../PlatformArrayPanel.lvclass", "Name"="PicoG-App.lvlib:PlatformArrayPanel.lvclass", "Referrer"=path "C:/dev/Vireo/PicoG/PicoG-App/PlatformArrayPanel/Panel Events.ctl"}, {"Path"=path "C:/dev/Vireo/PicoG/PicoG-App/PlatformArrayPanel/Outbound Events.ctl", "Name"="PicoG-App.lvlib:PlatformArrayPanel.lvclass:Outbound Events.ctl", "Referrer"=path "C:/dev/Vireo/PicoG/PicoG-App/PlatformArrayPanel/Outbound Events.ctl"}, {"Path"=path "../PlatformArrayPanel.lvclass", "Name"="PicoG-App.lvlib:PlatformArrayPanel.lvclass", "Referrer"=path "C:/dev/Vireo/PicoG/PicoG-App/PlatformArrayPanel/Outbound Events.ctl"}, {"Path"=path "../../../Builds/picoG/ppl/PicoG-Core.lvlibp/PicoG-Processor/PicoG-Core/Platform/Platform.lvclass", "Name"="PicoG-Core.lvlibp:Platform.lvclass", "Referrer"=path "C:/dev/Vireo/PicoG/PicoG-App/PlatformArrayPanel/Outbound Events.ctl"}, {"Path"=path "C:/dev/Vireo/PicoG/PicoG-App/DeviceArrayPanel/Ref Data.ctl", "Name"="PicoG-App.lvlib:DeviceArrayPanel.lvclass:Ref Data.ctl", "Referrer"=path "C:/dev/Vireo/PicoG/PicoG-App/DeviceArrayPanel/Ref Data.ctl"}, {"Path"=path "../DeviceArrayPanel.lvclass", "Name"="PicoG-App.lvlib:DeviceArrayPanel.lvclass", "Referrer"=path "C:/dev/Vireo/PicoG/PicoG-App/DeviceArrayPanel/Ref Data.ctl"}, {"Path"=path "../../Device/Device.lvclass", "Name"="PicoG-App.lvlib:Device.lvclass", "Referrer"=path "C:/dev/Vireo/PicoG/PicoG-App/DeviceArrayPanel/Ref Data.ctl"}, {"Path"=path "C:/dev/Vireo/PicoG/PicoG-App/DeviceArrayPanel/Inbound Events.ctl", "Name"="PicoG-App.lvlib:DeviceArrayPanel.lvclass:Inbound Events.ctl", "Referrer"=path "C:/dev/Vireo/PicoG/PicoG-App/DeviceArrayPanel/Inbound Events.ctl"}, {"Path"=path "../DeviceArrayPanel.lvclass", "Name"="PicoG-App.lvlib:DeviceArrayPanel.lvclass", "Referrer"=path "C:/dev/Vireo/PicoG/PicoG-App/DeviceArrayPanel/Inbound Events.ctl"}]
  in  "Paths":path=path "C:/dev/Vireo/PicoG/PicoG-App/picoG Main.vi"
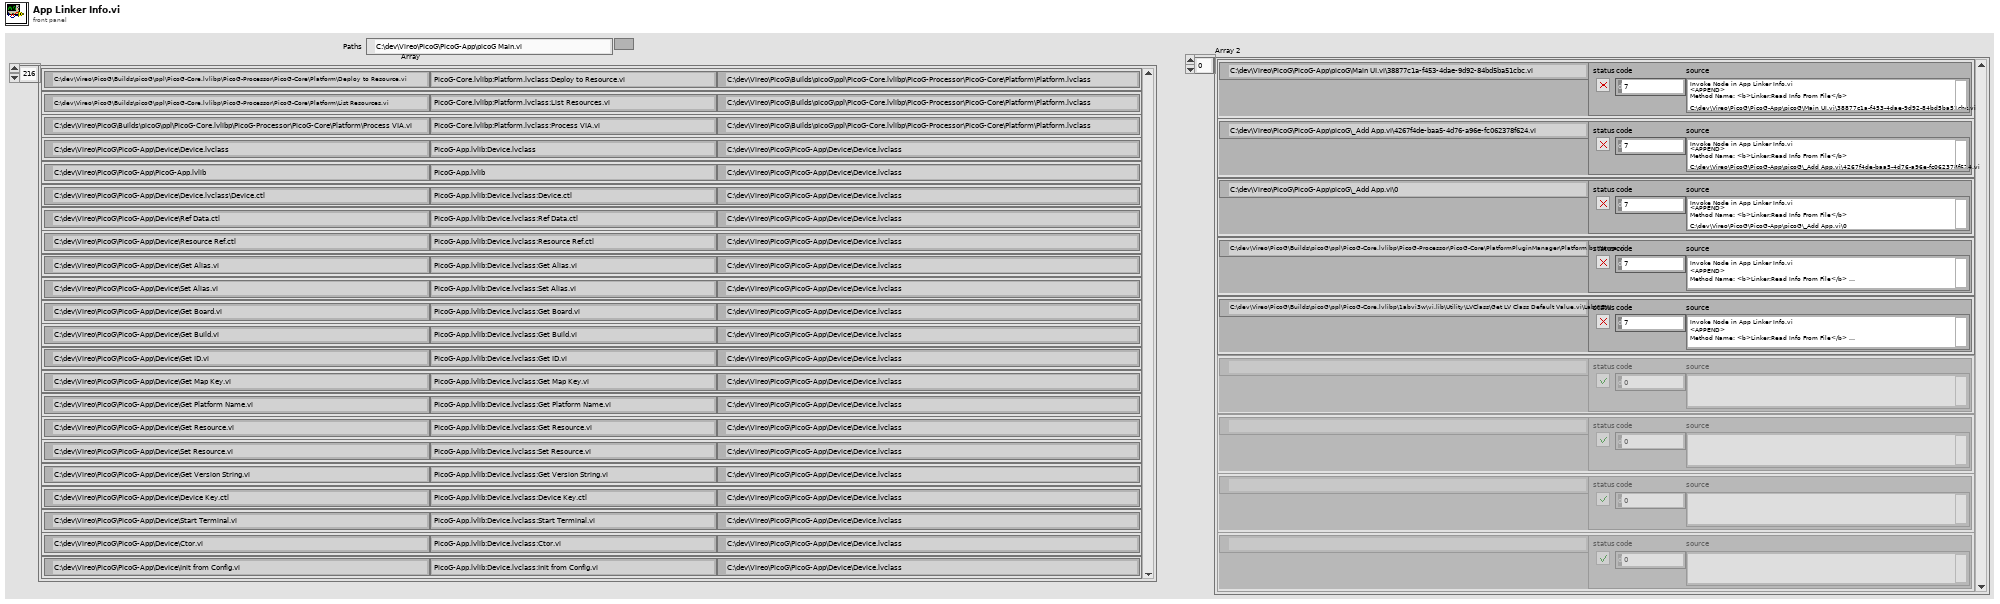
[diagram p1: front panel]
types:
  T1 = cluster{"Paths":path, "error out":errorcluster}[]
  T2 = cluster{"Path":path, "Name":string, "Referrer":path}[]
  T3 = cluster{"Path":path, "Name":string, "Referrer":path}
  T4 = typedef "NI_FileType.lvlib/LVFileType.ctl" = enum32{"Invalid file", "Unknown type", "Instrument", "Control", "Polymorphic VI", "Project", "Library", "LVClass", "XControl", "XNode", "Shared library", ".NET assembly", "ActiveX interface", "CIN", "Run-time menu", "Palette menu", "Help file", "LLB", "XNode Edit Dependency", "Class Private Data Control", "Statechart", "MathScript .m file", "Ladder Diagram", "LVLibp", "XNode Build Dependency"}
  T5 = cluster{"path":path, "delimited name":string, "type":T4, "iState":u32, "iStyle":u16, "wStyle":u16, "buttons":u16, "viflags":u32, "viflags2":u32, "links":u32[]}[]
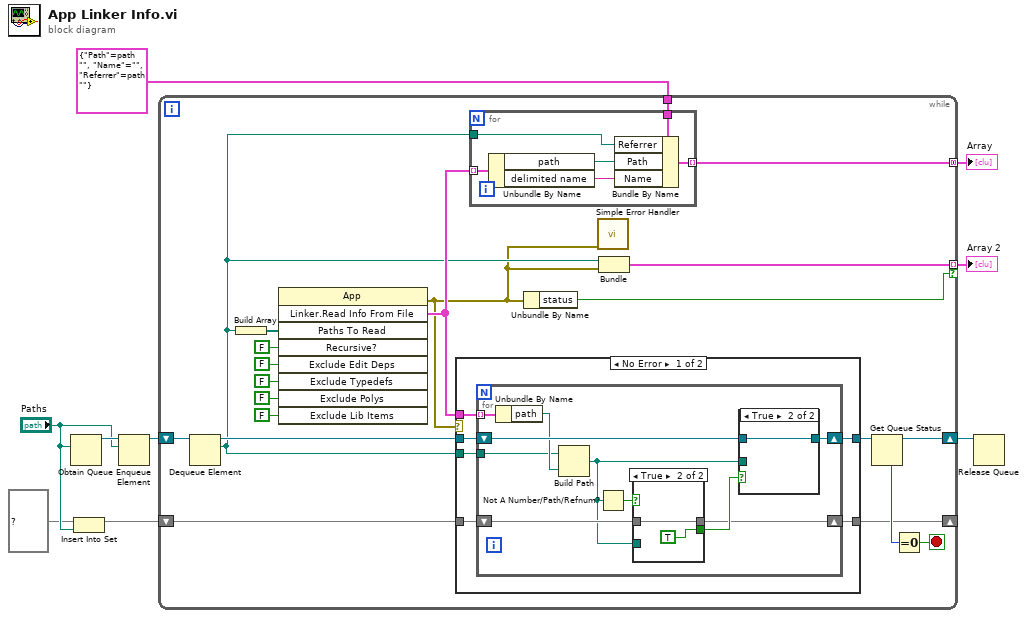
[diagram p0: block diagram]
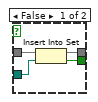
[diagram p2: hidden frame]
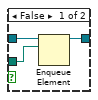
[diagram p3: hidden frame]
diagram:
  n1 = Obtain Queue(element data type="Paths") -> (queue out=w8:refnum<queue>)  [unwired: 4 in, 2 out]
  n2 = Insert Into Set(10:"Paths", 11:set{path} {} ("set in")) -> (3:w9:set{path})  [unwired: 1 out]
  n3 = Enqueue Element(queue=w8, element="Paths") -> (queue out=w6:refnum<queue>)  [unwired: 2 in, 2 out]
  n4 = while {
    shift-right: [w17] -> _
    shift-left: w9 -> [w18]
    shift-right: [w23] -> w4
    shift-left: w6 -> [w25]
    tunnel: T3 {"Path"=path "", "Name"="", "Referrer"=path ""} -> [w15]
    tunnel: [w14] -> w2 mode=concatenating
    tunnel: [w12] -> w1 mode=indexing if=w11
    stop <- w21 stop-if-true
    n5 = Dequeue Element(queue=w25) -> (queue out=w20:refnum<queue>, element=w13:path)  [unwired: 2 in, 2 out]
    n6 = Build Array(w13) -> (w24:path[])
    n7 = invoke class="App" method="Linker.Read Info From File"("Paths To Read"=w24, "Recursive?"=FALSE, "Exclude Edit Deps"=FALSE ("Exclude Edit Time Dependencies"), "Exclude Typedefs"=FALSE, "Exclude Polys"=FALSE ("Exclude Poly VIs"), "Exclude Lib Items"=FALSE ("Exclude Unused Library Items")) -> (error out=w10:errorcluster, "Linker.Read Info From File"=w16:T5)  [unwired: 3 in, 7 out]
    n8 = case shown="No Error" w10 {
      tunnel: w16 -> [w42 _]
      tunnel: w20 -> [w41 w64]
      tunnel: [w38 w64] -> w19
      tunnel: w18 -> [w40 w63]
      tunnel: [w39 w63] -> w17
      tunnel: w13 -> [w37 _]
      frame No Error {
        n9 = for {
          tunnel: w42 -> [w52] mode=indexing
          shift-right: [w49] -> w39
          shift-left: w40 -> [w51]
          shift-right: [w47] -> w38
          shift-left: w41 -> [w48]
          tunnel: w37 -> [w45]
          n10 = Unbundle By Name(w52) -> ("path"=w46:path)
          n11 = Build Path(base path=w45, name or relative path=w46) -> (appended path=w43:path)
          n12 = Not A Number/Path/Refnum?(number/path/refnum=w43) -> (NaN/Path/Refnum?=w44:bool)
          n13 = case shown="True" w44 {
            tunnel: w51 -> [w56 w57]
            tunnel: [w55 TRUE ("already included?")] -> w50
            tunnel: [w54 w57] -> w49
            tunnel: w43 -> [w53 _]
            frame False {
              n14 = Insert Into Set(10:w53, 11:w56) -> (2:w55:bool, 3:w54:set{path})
            }
            frame True {
            }
          }
          n15 = case shown="True" w50 {
            tunnel: w48 -> [w61 w62]
            tunnel: w43 -> [w59 _]
            tunnel: [w60 w62] -> w47
            frame False {
              n16 = Enqueue Element(queue=w61, element=w59) -> (queue out=w60:refnum<queue>)  [unwired: 2 in, 2 out]
            }
            frame True {
            }
          }
        }
      }
      frame Error {
      }
    }
    n17 = for {
      tunnel: w16 -> [w36] mode=indexing
      tunnel: w15 -> [w35]
      tunnel: w13 -> [w32]
      tunnel: [w31] -> w14 mode=indexing
      n18 = Unbundle By Name(w36) -> ("path"=w33:path, "delimited name"=w34:string)
      n19 = Bundle By Name(cluster=w35, "Referrer"=w32, "Path"=w33, "Name"=w34) -> (w31:T3)
    }
    n20 = Unbundle By Name(w10) -> ("status"=w11:bool)
    n21 = call <vilib>:"Simple Error Handler.vi"("error in (no error)"=w10) -> ()  [unwired: 4 in, 5 out]
    n22 = Bundle("Paths"=w13, "error out"=w10) -> (w12:cluster{"Paths":path, "error out":errorcluster})  [unwired: 1 in]
    n23 = Get Queue Status(queue=w19) -> (queue out=w23:refnum<queue>, # elements in queue=w22:i32)  [unwired: 2 in, 6 out]
    n24 = Equal To 0?(x=w22) -> (x = 0?=w21:bool)
  }
  "Array" <- w2
  "Array 2" <- w1
  n25 = Release Queue(queue=w4) -> ()  [unwired: 2 in, 3 out]
